vi "Wago Main Driver.vi"(10 "Remote Port":u16=502, 11 "Remote IP Address":string="172.16.90.113") -> (3 "System Data":string[][](array[string])=[["Station 1 Volt 1", "166.520"], ["Station 1 Volt 2", "0.030"], ["Station 2 Volt 1", "166.120"], ["Station 2 Volt 2", "90.720"], ["Station 3 Volt 1", "166.280"], ["Station 3 Volt 2", "91.440"], ["Station 4 Volt 1", "165.960"], ["Station 4 Volt 2", "94.400"], ["Station 5 Volt 1", "166.040"], ["Station 5 Volt 2", "94.800"], ["Station 6 Volt 1", "166.200"], ["Station 6 Volt 2", "93.280"], ["Station 7 Volt 1", "166.040"], ["Station 7 Volt 2", "90.720"], ["Station 8 Volt 1", "165.720"], ["Station 8 Volt 2", "88.320"], ["Room Humidity (Measured)", "175.560"], ["Room Temperature (Measured)", "183.880"], ["Spare 1", "0.000"], ["Spare 2", "0.000"], ["Supply Temperature (Measured)", "3.100"], ["Cooling Temperature (Measured)", "2.950"], ["Dehumidification Temperatuer (Measured)", "2.210"], ["Unused", "327.670"], ["Volt Rate 1", "5"], ["Volt Rate 2", "5"], ["Volt Rate 3", "0"], ["Volt Rate 4", "0"], ["Volt Rate 5", "0"], ["Volt Rate 6", "0"], ["Volt Rate 7", "0"], ["Volt Rate 8", "0"], ["Volt Window 1", "30"], ["Volt Window 2", "60"], ["Volt Window 3", "0"], ["Volt Window 4", "0"], ["Volt Window 5", "30"], ["Volt Window 6", "60"], ["Volt Window 7", "0"], ["Volt Window 8", "0"], ["Voltage Setpoint 1", "115.260"], ["Voltage Setpoint 2", "115.150"], ["Voltage Setpoint 3", "115.370"], ["Voltage Setpoint 4", "115.080"], ["Voltage Setpoint 5", "115.170"], ["Voltage Setpoint 6", "115.310"], ["Voltage Setpoint 7", "115.310"], ["Voltage Setpoint 8", "114.850"], ["Volt Range 1", "1"], ["Volt Range 2", "1"], ["Volt Range 3", "1"], ["Volt Range 4", "1"], ["Volt Range 5", "1"], ["Volt Range 6", "1"], ["Volt Range 7", "1"], ["Volt Range 8", "1"], ["Volt Polarity 1", "0"], ["Volt Polarity 2", "0"], ["Volt Polarity 3", "0"], ["Volt Polarity 4", "0"], ["Volt Polarity 5", "0"], ["Volt Polarity 6", "0"], ["Volt Polarity 7", "0"], ["Volt Polarity 8", "0"], ["Room Setpoint Temperature", "90.000"], ["Room Setpoint Humidity", "20.000"], ["Room Cool Temperature", "85.000"], ["Room Dehumidification Temperature", "75.000"], ["Room Run", "True"], ["Room OK", "False"], ["Room Testing", "False"], ["Emergency Stop", "True"], ["Chamber Door Switch", "True"], ["Safety Switch", "True"], ["Room Dry P", "200"], ["Room Dry I", "15000"], ["Room Humidity P", "400"], ["Room Humidity I", "15000"], ["Room Heat P", "1000"], ["Room Heat I", "2000"], ["Room Cool Temperature P", "500"], ["Room Cool Temperature I", "6000"], ["Room Dehumidification Temperature P", "500"], ["Room Dehumidification Temperature I", "6000"], ["Dehumidification Control (Wago Output)", "8191"], ["Cool Control (Wago Output)", "8129"], ["Steam Control (Wago Output)", "0"], ["Heat Control (Wago Output)", "12620"], ["Room Temperature (°F)", "90.140"], ["Room Humidity (%)", "41.960"], ["Supply Temperature (°F)", "87.670"], ["Cool Temperature (°F)", "85.060"], ["Dehumidification Temperature (°F)", "71.920"], ["Glycol Temperature (°F)", "0.000"], ["Heat Rate (%)", "23.140"], ["Steam Rate (%)", "0.000"], ["Cool Rate (%)", "24.810"], ["Dehumidification Rate (%)", "0.000"], ["Room Status", "0"], ["Door Enable", "1"], ["Station 1, Door 1", "0"], ["Station 1, Door 2", "0"], ["Station 1, Door 3", "0"], ["Station 2, Door 1", "0"], ["Station 2, Door 2", "0"], ["Station 2, Door 3", "0"], ["Station 3, Door 1", "0"], ["Station 3, Door 2", "0"], ["Station 3, Door 3", "0"], ["Station 4, Door 1", "0"], ["Station 4, Door 2", "0"], ["Station 4, Door 3", "0"], ["Station 5, Door 1", "1607"], ["Station 5, Door 2", "1607"], ["Station 5, Door 3", "1607"], ["Station 6, Door 1", "0"], ["Station 6, Door 2", "0"], ["Station 6, Door 3", "0"], ["Station 7, Door 1", "0"], ["Station 7, Door 2", "0"], ["Station 7, Door 3", "0"], ["Station 8, Door 1", "0"], ["Station 8, Door 2", "0"], ["Station 8, Door 3", "0"], ["Door Opener Enable", "True"], ["Volt Monitor 1", "115.260"], ["Volt Monitor 2", "115.150"], ["Volt Monitor 3", "115.370"], ["Volt Monitor 4", "115.080"], ["Volt Monitor 5", "115.170"], ["Volt Monitor 6", "115.310"], ["Volt Monitor 7", "115.310"], ["Volt Monitor 8", "114.850"], ["Volt Status 1", "1"], ["Volt Status 2", "1"], ["Volt Status 3", "1"], ["Volt Status 4", "1"], ["Volt Status 5", "1"], ["Volt Status 6", "1"], ["Volt Status 7", "1"], ["Volt Status 8", "1"], ["60 Hz Power", "True"], ["50 Hz Power", "False"], ["120V Range", "True"], ["240V Range", "False"], ["Ground Line", "False"], ["Ground Neutral", "True"], ["Measure Ground Leakage Current (mA)", "Measure GL"], ["Room OK", "True"], ["60 Hz Power", "True"], ["50 Hz Power", "False"], ["120V Range", "True"], ["240V Range", "False"], ["Ground Line", "False"], ["Ground Neutral", "True"], ["Measure Ground Leakage Current (mA)", "Disable GL Measure"], ["Fault", "False"], ["60 Hz Power", "True"], ["50 Hz Power", "False"], ["120V Range", "True"], ["240V Range", "False"], ["Ground Line", "False"], ["Ground Neutral", "True"], ["Measure Ground Leakage Current (mA)", "Disable GL Measure"], ["Room Heat", "True"], ["60 Hz Power", "True"], ["50 Hz Power", "False"], ["120V Range", "True"], ["240V Range", "False"], ["Ground Line", "False"], ["Ground Neutral", "True"], ["Measure Ground Leakage Current (mA)", "Disable GL Measure"], ["Room Blower", "True"], ["60 Hz Power", "True"], ["50 Hz Power", "False"], ["120V Range", "True"], ["240V Range", "False"], ["Ground Line", "False"], ["Ground Neutral", "True"], ["Measure Ground Leakage Current (mA)", "Disable GL Measure"], ["Spare", "False"], ["60 Hz Power", "True"], ["50 Hz Power", "False"], ["120V Range", "True"], ["240V Range", "False"], ["Ground Line", "False"], ["Ground Neutral", "True"], ["Measure Ground Leakage Current (mA)", "Disable GL Measure"], ["Room Pump", "True"], ["60 Hz Power", "True"], ["50 Hz Power", "False"], ["120V Range", "True"], ["240V Range", "False"], ["Ground Line", "False"], ["Ground Neutral", "True"], ["Measure Ground Leakage Current (mA)", "Disable GL Measure"], ["Room OK", "False"], ["60 Hz Power", "True"], ["50 Hz Power", "False"], ["120V Range", "True"], ["240V Range", "False"], ["Ground Line", "False"], ["Ground Neutral", "True"], ["Measure Ground Leakage Current (mA)", "Disable GL Measure"], ["Fault", "False"], ["Station 1 Freezer", "False"], ["Station 1 Cab", "False"], ["Station 1 Slide", "False"], ["Station 2 Freezer", "False"], ["Station 2 Cab", "False"], ["Station 2 Slide", "False"], ["Station 3 Freezer", "False"], ["Station 3 Cab", "False"], ["Station 3 Slide", "False"], ["Station 4 Freezer", "False"], ["Station 4 Cab", "False"], ["Station 4 Slide", "False"], ["Station 5 Freezer", "False"], ["Station 5 Cab", "False"], ["Station 5 Slide", "False"], ["Station 6 Freezer", "False"], ["Station 6 Cab", "False"], ["Station 6 Slide", "False"], ["Station 7 Freezer", "False"], ["Station 7 Cab", "False"], ["Station 7 Slide", "False"], ["Station 8 Freezer", "False"], ["Station 8 Cab", "False"], ["Station 8 Slide", "False"], ["Station 1 Volt Increase", "False"], ["Station 1 Volt Decrease", "False"], ["Station 2 Volt Increase", "False"], ["Station 2 Volt Decrease", "False"], ["Station 3 Volt Increase", "False"], ["Station 3 Volt Decrease", "False"], ["Station 4 Volt Increase", "False"], ["Station 4 Volt Decrease", "False"], ["Station 5 Volt Increase", "False"], ["Station 5 Volt Decrease", "False"], ["Station 6 Volt Increase", "False"], ["Station 6 Volt Decrease", "False"], ["Station 7 Volt Increase", "False"], ["Station 7 Volt Decrease", "False"], ["Station 8 Volt Increase", "False"], ["Station 8 Volt Decrease", "False"]])   [LabVIEW 2016]
uses:
  Type Definitions/Wago Main Control.ctl
  Type Definitions/Wago Output Data Process Image.ctl
  Type Definitions/Wago Room Condtions.ctl
  Type Definitions/Wago Door Relays.ctl
  Type Definitions/Wago Contactor Settings.ctl
  Type Definitions/Wago Ground Leakage.ctl
  Type Definitions/Wago Input Process Image.ctl
  Type Definitions/Wago Room PID Settings.ctl
  Type Definitions/Wago Measured Input Data.ctl
  Type Definitions/Wago Room Setpoint Targets.ctl
  Type Definitions/Wago Ground Leakage Relays.ctl
  Type Definitions/Wago Door Settings.ctl
  Type Definitions/Wago Door Relays By Station.ctl
  Type Definitions/Wago Door Operation.ctl
  Trunk/Refrigeration/RTS/Type Definitions/RTS Enable Door Openers.ctl
  Type Definitions/Wago Polarity Selector Relays.ctl
  Type Definitions/Wago Polarity Selector.ctl
  Type Definitions/Wago Room Enable.ctl
  Type Definitions/Wago Room Run.ctl
  Type Definitions/Wago Voltage Adjustment Parameters.ctl
  Trunk/Refrigeration/RTS/Type Definitions/RTS Frequency Selector.ctl
  Trunk/Refrigeration/RTS/Type Definitions/RTS Chamber Temperature Humidity Control.ctl
  Type Definitions/Wago Input Commands.ctl
  <vilib>/NI/Modbus Library/API/Wrapper/Create TCP Master.vi
  <vilib>/NI/Modbus Library/API/Master/Modbus Master.lvclass
  <vilib>/NI/Modbus Library/API/Wrapper/API Main.lvlib
panel:
  out "System Data to Save":string[][](array[string])=[["Room Temperature (°F)", "90.140"], ["Room Humidity (%)", "41.960"], ["Supply Temperature (°F)", "87.670"], ["Cool Temperature (°F)", "85.060"], ["Dehumidification Temperature (°F)", "71.920"], ["Glycol Temperature (°F)", "0.000"], ["Heat Rate (%)", "23.140"], ["Steam Rate (%)", "0.000"], ["Cool Rate (%)", "24.810"], ["Dehumidification Rate (%)", "0.000"], ["Room Status", "0"], ["Door Enable", "1"]]
  in  "Tab Control":enum32{"Setup Tab", "Relay Tab"}(tab)
  in  "Room Setpoints":T1={"Room Setpoint Temperature (*RM Dry Set P1)"=90.0, "Room Setpoint Humidity (*RM Hum Set P1)"=20.0, "Room Cool Temperature (*RM Cool Setp 1)"=65.0, "Room Dehum Temperature (*RM De Hum Set P1)"=60.0} {"Room Dehum Temperature (*RM De Hum Set P1)" min=30.0 max=120.0; "Room Cool Temperature (*RM Cool Setp 1)" min=30.0 max=120.0; "Room Setpoint Humidity (*RM Hum Set P1)" min=5.0 max=98.0; "Room Setpoint Temperature (*RM Dry Set P1)" min=40.0 max=120.0}
  in  "Path":path=path "C:/Technology Lab/NI-2010/Trunk/Refrigeration/RTS/Old System"
  in  "Reload PID":bool
  in  "Room PID Parameters":bool
  in  "Room PID Settings":T2={"Room Dry P(*RM Dry P1)"=2, "Room Dry I (*RM Dry I1)"=1500, "Room Humidity P (*RM Hum P1)"=4, "Room Humidity I (*RM Hum I1)"=1500, "Room Heat P (*RM Heat P1)"=10, "Room Heat I (*RM Heat I1)"=200, "Room Cool Temperature P (*RM Cool P1)"=5, "Room Cool Temperature I (*RM Cool I1)"=600, "Room Dehumid Temperature P (*RM Dehum P1)"=5, "Room Dehumid Temperature I (*RM Dehum I1)"=600} {"Room Dehumid Temperature I (*RM Dehum I1)" max=30000 step=1; "Room Dehumid Temperature P (*RM Dehum P1)" max=30000 step=1; "Room Cool Temperature I (*RM Cool I1)" max=30000 step=1; "Room Cool Temperature P (*RM Cool P1)" max=30000 step=1; "Room Heat I (*RM Heat I1)" max=30000 step=1; "Room Heat P (*RM Heat P1)" max=30000 step=1; "Room Humidity I (*RM Hum I1)" max=30000 step=1; "Room Humidity P (*RM Hum P1)" max=30000 step=1; "Room Dry I (*RM Dry I1)" max=30000 step=1; "Room Dry P(*RM Dry P1)" max=30000 step=1}
  in  "Chamber Setpoint":bool
  in  "Update Voltage Adjustment Parameters":bool
  in  "Voltage Adjustment Parameters":T3={"Volt Rate 1"=30, "Volt Rate 2"=30, "Volt Rate 3"=30, "Volt Rate 4"=30, "Volt Rate 5"=30, "Volt Rate 6"=30, "Volt Rate 7"=30, "Volt Rate 8"=30, "Volt Window 1 & 5"=10, "Volt Window 2 & 6"=10, "Volt Window 3 & 7 "=10, "Volt Window 4 & 8"=10}
  in  "Room OK?":T4
  in  "Room Run":T5
  in  "OK":bool
  in  "Voltage 8":dbl
  in  "Frequency 8":T6 items=["60 Hz", "50 Hz"]
  in  "Voltage 7":dbl
  in  "Frequency 7":T6 items=["60 Hz", "50 Hz"]
  in  "Voltage 6":dbl
  in  "Frequency 6":T6 items=["60 Hz", "50 Hz"]
  in  "Voltage 5":dbl
  in  "Frequency 5":T6 items=["60 Hz", "50 Hz"]
  in  "Voltage 4":dbl
  in  "Frequency 4":T6 items=["60 Hz", "50 Hz"]
  in  "Voltage 3":dbl
  in  "Frequency 3":T6 items=["60 Hz", "50 Hz"]
  in  "Voltage 2":dbl
  in  "Frequency 2":T6 items=["60 Hz", "50 Hz"]
  in  "Voltage":dbl
  in  "Frequency":T6 items=["60 Hz", "50 Hz"]
  in  "Ground Leak Relays":T7
  in  "Polarity Selector":T9
  in  "Station 8 CMD":bool
  in  "Station 7 CMD":bool
  in  "Station 6 CMD":bool
  in  "Station 5 CMD":bool
  in  "Station 4 CMD":bool
  in  "Station 3 CMD":bool
  in  "Station 2 CMD":bool
  in  "Station 1 CMD":bool
  in  "Door Settings":T11={"Station 1"={"Freezer"=enum."Clear Time Close Door", "Cab"=enum."Clear Time Close Door", "Slide"=enum."Clear Time Close Door"}, "Station 2"={"Freezer"=enum."Clear Time Close Door", "Cab"=enum."Clear Time Close Door", "Slide"=enum."Clear Time Close Door"}, "Station 3"={"Freezer"=enum."Clear Time Close Door", "Cab"=enum."Clear Time Close Door", "Slide"=enum."Clear Time Close Door"}, "Station 4"={"Freezer"=enum."Clear Time Close Door", "Cab"=enum."Clear Time Close Door", "Slide"=enum."Clear Time Close Door"}, "Station 5"={"Freezer"=enum."Clear Time Close Door", "Cab"=enum."Clear Time Close Door", "Slide"=enum."Clear Time Close Door"}, "Station 6"={"Freezer"=enum."Clear Time Close Door", "Cab"=enum."Clear Time Close Door", "Slide"=enum."Clear Time Close Door"}, "Station 7"={"Freezer"=enum."Clear Time Close Door", "Cab"=enum."Clear Time Close Door", "Slide"=enum."Clear Time Close Door"}, "Station 8"={"Freezer"=enum."Clear Time Close Door", "Cab"=enum."Clear Time Close Door", "Slide"=enum."Clear Time Close Door"}, "Door Enable"=enum."Enable Door Openers"}
  in  "Station Voltage Send 1":bool
  in  "Station Voltage Send 5":bool
  in  "Station Voltage Send 2":bool
  in  "Station Voltage Send 6":bool
  in  "Station Voltage Send 3":bool
  in  "Station Voltage Send 7":bool
  in  "Station Voltage Send 4":bool
  in  "Station Voltage Send 8":bool
  out "Wago Data Output":T15={"Output Data Process Image"={"Room Door Opener Status"={"Station 1, Door 1"=0, "Station 1, Door 2"=0, "Station 1, Door 3"=0, "Station 2, Door 1"=0, "Station 2, Door 2"=1615, "Station 2, Door 3"=0, "Station 3, Door 1"=1615, "Station 3, Door 2"=1611, "Station 3, Door 3"=0, "Station 4, Door 1"=4807, "Station 4, Door 2"=0, "Station 4, Door 3"=0, "Station 5, Door 1"=1615, "Station 5, Door 2"=0, "Station 5, Door 3"=1611, "Station 6, Door 1"=1611, "Station 6, Door 2"=0, "Station 6, Door 3"=4803, "Station 7, Door 1"=0, "Station 7, Door 2"=0, "Station 7, Door 3"=1611, "Station 8, Door 1"=0, "Station 8, Door 2"=1611, "Station 8, Door 3"=1611}, "Room Conditions (Measured)"={"twDoorEna(*Door Enable)"=1, "twStatus(*Rm Status1)"=0, "twRoomTemp (*Rm Dry1)"=90.14, "twRoomHum (*Rm Hum1)"=23.75, "twSuppTemp(*Rm Supp T1)"=87.49, "twCoolTemp(*Rm Cool T1)"=86.5, "twDehumTemp(*Rm Dehum T1)"=72.19, "twGlycolTemp(*Rm Gly T1-Not Used)"=0.0, "twDehumRate(*Rm Dehum Valve1)"=68.17, "twCoolRate(*Rm Cool Valve1)"=15.6, "twSteamRate(*Rm Steam Valve1)"=0.0, "twHeatRate (*Rm Heat Ctrl1)"=33.98}, "Chamber AO Controls (Controls Chamber)"={"twDehumCtrl (mA)"=249, "twCoolCtrl (mA)"=51, "twSteamCtrl (mA)"=0, "twHeatCtrl (mA)"=155}, "Variac Output(*All Check Out)"={"Station 1 Volt Increase"=FALSE, "Station 1 Volt Decrease"=FALSE, "Station 2 Volt Increase"=FALSE, "Station 2 Volt Decrease"=FALSE, "Station 3 Volt Increase"=FALSE, "Station 3 Volt Decrease"=FALSE, "Station 4 Volt Increase"=FALSE, "Station 4 Volt Decrease"=FALSE, "Station 5 Volt Increase"=FALSE, "Station 5 Volt Decrease"=FALSE, "Station 6 Volt Increase"=FALSE, "Station 6 Volt Decrease"=FALSE, "Station 7 Volt Increase"=FALSE, "Station 7 Volt Decrease"=FALSE, "Station 8 Volt Increase"=FALSE, "Station 8 Volt Decrease"=FALSE}, "Door Output Relays"={"Station 1 Freezer"=FALSE, "Station 1 Cab"=FALSE, "Station 1 Slide"=FALSE, "Station 2 Freezer"=FALSE, "Station 2 Cab"=FALSE, "Station 2 Slide"=FALSE, "Station 3 Freezer"=FALSE, "Station 3 Cab"=FALSE, "Station 3 Slide"=FALSE, "Station 4 Freezer"=FALSE, "Station 4 Cab"=FALSE, "Station 4 Slide"=FALSE, "Station 5 Freezer"=FALSE, "Station 5 Cab"=FALSE, "Station 5 Slide"=FALSE, "Station 6 Freezer"=FALSE, "Station 6 Cab"=FALSE, "Station 6 Slide"=FALSE, "Station 7 Freezer"=FALSE, "Station 7 Cab"=FALSE, "Station 7 Slide"=FALSE, "Station 8 Freezer"=FALSE, "Station 8 Cab"=FALSE, "Station 8 Slide"=FALSE, "Door Opener Enable"=TRUE}, "Wago Input Voltage Monitor (*Target_ All Check Out)"={"twWoltMon1"=115.06, "twWoltMon2"=115.3, "twWoltMon3"=115.37, "twWoltMon4"=115.21, "twWoltMon5"=115.39, "twWoltMon6"=115.22, "twWoltMon7"=115.26, "twWoltMon8"=119.98, "twVoltStat1"=1, "twVoltStat2"=1, "twVoltStat3"=1, "twVoltStat4"=1, "twVoltStat5"=1, "twVoltStat6"=1, "twVoltStat7"=1, "twVoltStat8"=1}, "Contactor Settings(*All Check Out)"={"Station 1"={"60 Hz Power"=TRUE, "50 Hz Power"=FALSE, "120V Range"=TRUE, "240V Range"=FALSE, "Ground Line"=FALSE, "Ground Neutral"=TRUE, "Room OK"=FALSE, "Ground Leakage"=enum."1 - Measure GL"}, "Station 2"={"60 Hz Power"=TRUE, "50 Hz Power"=FALSE, "120V Range"=TRUE, "240V Range"=FALSE, "Ground Line"=FALSE, "Ground Neutral"=TRUE, "Fault"=FALSE, "Ground Leakage"=enum."1 - Measure GL"}, "Station 3"={"60 Hz Power"=TRUE, "50 Hz Power"=FALSE, "120V Range"=TRUE, "240V Range"=FALSE, "Ground Line"=FALSE, "Ground Neutral"=TRUE, "Room Heat"=TRUE, "Ground Leakage"=enum."1 - Measure GL"}, "Station 4"={"60 Hz Power"=TRUE, "50 Hz Power"=FALSE, "120V Range"=TRUE, "240V Range"=FALSE, "Ground Line"=FALSE, "Ground Neutral"=TRUE, "Room Blower"=TRUE, "Ground Leakage"=enum."1 - Measure GL"}, "Station 5"={"60 Hz Power"=TRUE, "50 Hz Power"=FALSE, "120V Range"=TRUE, "240V Range"=FALSE, "Ground Line"=FALSE, "Ground Neutral"=TRUE, "Spare"=FALSE, "Ground Leakage"=enum."0 - Normal GL"}, "Station 6"={"60 Hz Power"=TRUE, "50 Hz Power"=FALSE, "120V Range"=TRUE, "240V Range"=FALSE, "Ground Line"=FALSE, "Ground Neutral"=TRUE, "Room Pump"=TRUE, "Ground Leakage"=enum."0 - Normal GL"}, "Station 7"={"60 Hz Power"=TRUE, "50 Hz Power"=FALSE, "120V Range"=TRUE, "240V Range"=FALSE, "Ground Line"=FALSE, "Ground Neutral"=TRUE, "Spare"=FALSE, "Ground Leakage"=enum."0 - Normal GL"}, "Station 8"={"60 Hz Power"=TRUE, "50 Hz Power"=FALSE, "120V Range"=TRUE, "240V Range"=FALSE, "Ground Line"=FALSE, "Ground Neutral"=TRUE, "Spare"=FALSE, "Ground Leakage"=enum."0 - Normal GL"}}}, "Input Process Image"={"fbEstop"=TRUE, "fbDoors"=TRUE, "fbSafety"=TRUE, "Input Variables"={"Station 1 Volt 1"=65.36, "Station 1 Volt 2"=65.12, "Station 2 Volt 1"=166.04, "Station 2 Volt 2"=77.04, "Station 3 Volt 1"=166.12, "Station 3 Volt 2"=80.08, "Station 4 Volt 1"=166.04, "Station 4 Volt 2"=86.32, "Station 5 Volt 1"=166.2, "Station 5 Volt 2"=89.84, "Station 6 Volt 1"=166.28, "Station 6 Volt 2"=81.76, "Station 7 Volt 1"=166.36, "Station 7 Votl 2"=78.64, "Station 8 Volt 1"=170.28, "Station 8 Volt 2"=75.76}, "Input Data"={"Room Humidity  (Measured)"=127.52, "Room Temperature (Measured)"=183.8, "Spare 1"=0.0, "Spare 2"=0.0, "Supply Temperature (Measured)"=3.1, "Cooling Temperature (Measured)"=3.03, "Dehumidification Temperature (Measured)"=2.21, "Un-used"=327.67}, "Software Constants"={"Volt Rate 1"=0, "Volt Rate 2"=0, "Volt Rate 3"=0, "Volt Rate 4"=0, "Volt Rate 5"=0, "Volt Rate 6"=0, "Volt Rate 7"=0, "Volt Rate 8"=0, "Volt Window 1"=0, "Volt Window 2"=1, "Volt Window 3"=0, "Volt Window 4"=0, "Volt Window 5"=0, "Volt Window 6"=1, "Volt Window 7"=0, "Volt Window 8"=0, "Voltage Range 1"=0, "Voltage Range 2"=0, "Voltage Range 3"=0, "Voltage Range 4"=0, "Voltage Range 5"=0, "Voltage Range 6"=0, "Voltage Range 7"=0, "Voltage Range 8"=0, "Voltage Polarity 1"=0, "Voltage Polarity 2"=0, "Voltage Polarity 3"=0, "Voltage Polarity 4"=0, "Voltage Polarity 5"=0, "Voltage Polarity 6"=0, "Voltage Polarity 7"=0, "Voltage Polarity 8"=0, "Room Run"=TRUE, "Room OK"=FALSE, "Room Testing"=FALSE, "Room PID Settings"={"Room Dry P(*RM Dry P1)"=2, "Room Dry I (*RM Dry I1)"=1500, "Room Humidity P (*RM Hum P1)"=4, "Room Humidity I (*RM Hum I1)"=1500, "Room Heat P (*RM Heat P1)"=10, "Room Heat I (*RM Heat I1)"=200, "Room Cool Temperature P (*RM Cool P1)"=5, "Room Cool Temperature I (*RM Cool I1)"=600, "Room Dehumid Temperature P (*RM Dehum P1)"=5, "Room Dehumid Temperature I (*RM Dehum I1)"=600}}, "Measured Input Data (Target)"={"Voltage Setpoint 1 (*Volt Set1)"=115.06, "Voltage Setpoint 2 (*Volt Set2)"=115.3, "Voltage Setpoint 3 (*Volt Set3)"=115.37, "Voltage Setpoint 4 (*Volt Set4)"=115.21, "Voltage Setpoint 5 (*Volt Set5)"=115.39, "Voltage Setpoint 6 (*Volt Set6)"=115.22, "Voltage Setpoint 7 (*Volt Set7)"=115.26, "Voltage Setpoint 8 (*Volt Set8)"=119.98, "Room Setpoints"={"Room Setpoint Temperature (*RM Dry Set P1)"=90.0, "Room Setpoint Humidity (*RM Hum Set P1)"=20.0, "Room Cool Temperature (*RM Cool Setp 1)"=85.0, "Room Dehum Temperature (*RM De Hum Set P1)"=70.0}}}, "System Send Data"=[], "System Data To Save"=[]} {"Input Process Image"."Software Constants"."Room PID Settings"."Room Dehumid Temperature I (*RM Dehum I1)" max=30000 step=1; "Input Process Image"."Software Constants"."Room PID Settings"."Room Dehumid Temperature P (*RM Dehum P1)" max=30000 step=1; "Input Process Image"."Software Constants"."Room PID Settings"."Room Cool Temperature I (*RM Cool I1)" max=30000 step=1; "Input Process Image"."Software Constants"."Room PID Settings"."Room Cool Temperature P (*RM Cool P1)" max=30000 step=1; "Input Process Image"."Software Constants"."Room PID Settings"."Room Heat I (*RM Heat I1)" max=30000 step=1; "Input Process Image"."Software Constants"."Room PID Settings"."Room Heat P (*RM Heat P1)" max=30000 step=1; "Input Process Image"."Software Constants"."Room PID Settings"."Room Humidity I (*RM Hum I1)" max=30000 step=1; "Input Process Image"."Software Constants"."Room PID Settings"."Room Humidity P (*RM Hum P1)" max=30000 step=1; "Input Process Image"."Software Constants"."Room PID Settings"."Room Dry I (*RM Dry I1)" max=30000 step=1; "Input Process Image"."Software Constants"."Room PID Settings"."Room Dry P(*RM Dry P1)" max=30000 step=1}
  in  "Wago Data Input":T15 {"Input Process Image"."Software Constants"."Room PID Settings"."Room Dehumid Temperature I (*RM Dehum I1)" max=30000 step=1; "Input Process Image"."Software Constants"."Room PID Settings"."Room Dehumid Temperature P (*RM Dehum P1)" max=30000 step=1; "Input Process Image"."Software Constants"."Room PID Settings"."Room Cool Temperature I (*RM Cool I1)" max=30000 step=1; "Input Process Image"."Software Constants"."Room PID Settings"."Room Cool Temperature P (*RM Cool P1)" max=30000 step=1; "Input Process Image"."Software Constants"."Room PID Settings"."Room Heat I (*RM Heat I1)" max=30000 step=1; "Input Process Image"."Software Constants"."Room PID Settings"."Room Heat P (*RM Heat P1)" max=30000 step=1; "Input Process Image"."Software Constants"."Room PID Settings"."Room Humidity I (*RM Hum I1)" max=30000 step=1; "Input Process Image"."Software Constants"."Room PID Settings"."Room Humidity P (*RM Hum P1)" max=30000 step=1; "Input Process Image"."Software Constants"."Room PID Settings"."Room Dry I (*RM Dry I1)" max=30000 step=1; "Input Process Image"."Software Constants"."Room PID Settings"."Room Dry P(*RM Dry P1)" max=30000 step=1}
  out "Error Out":errorcluster
  in  "Error In":errorcluster
  # "Need to pull directly from PLC..I cannont seem to\nfind the correct values :("
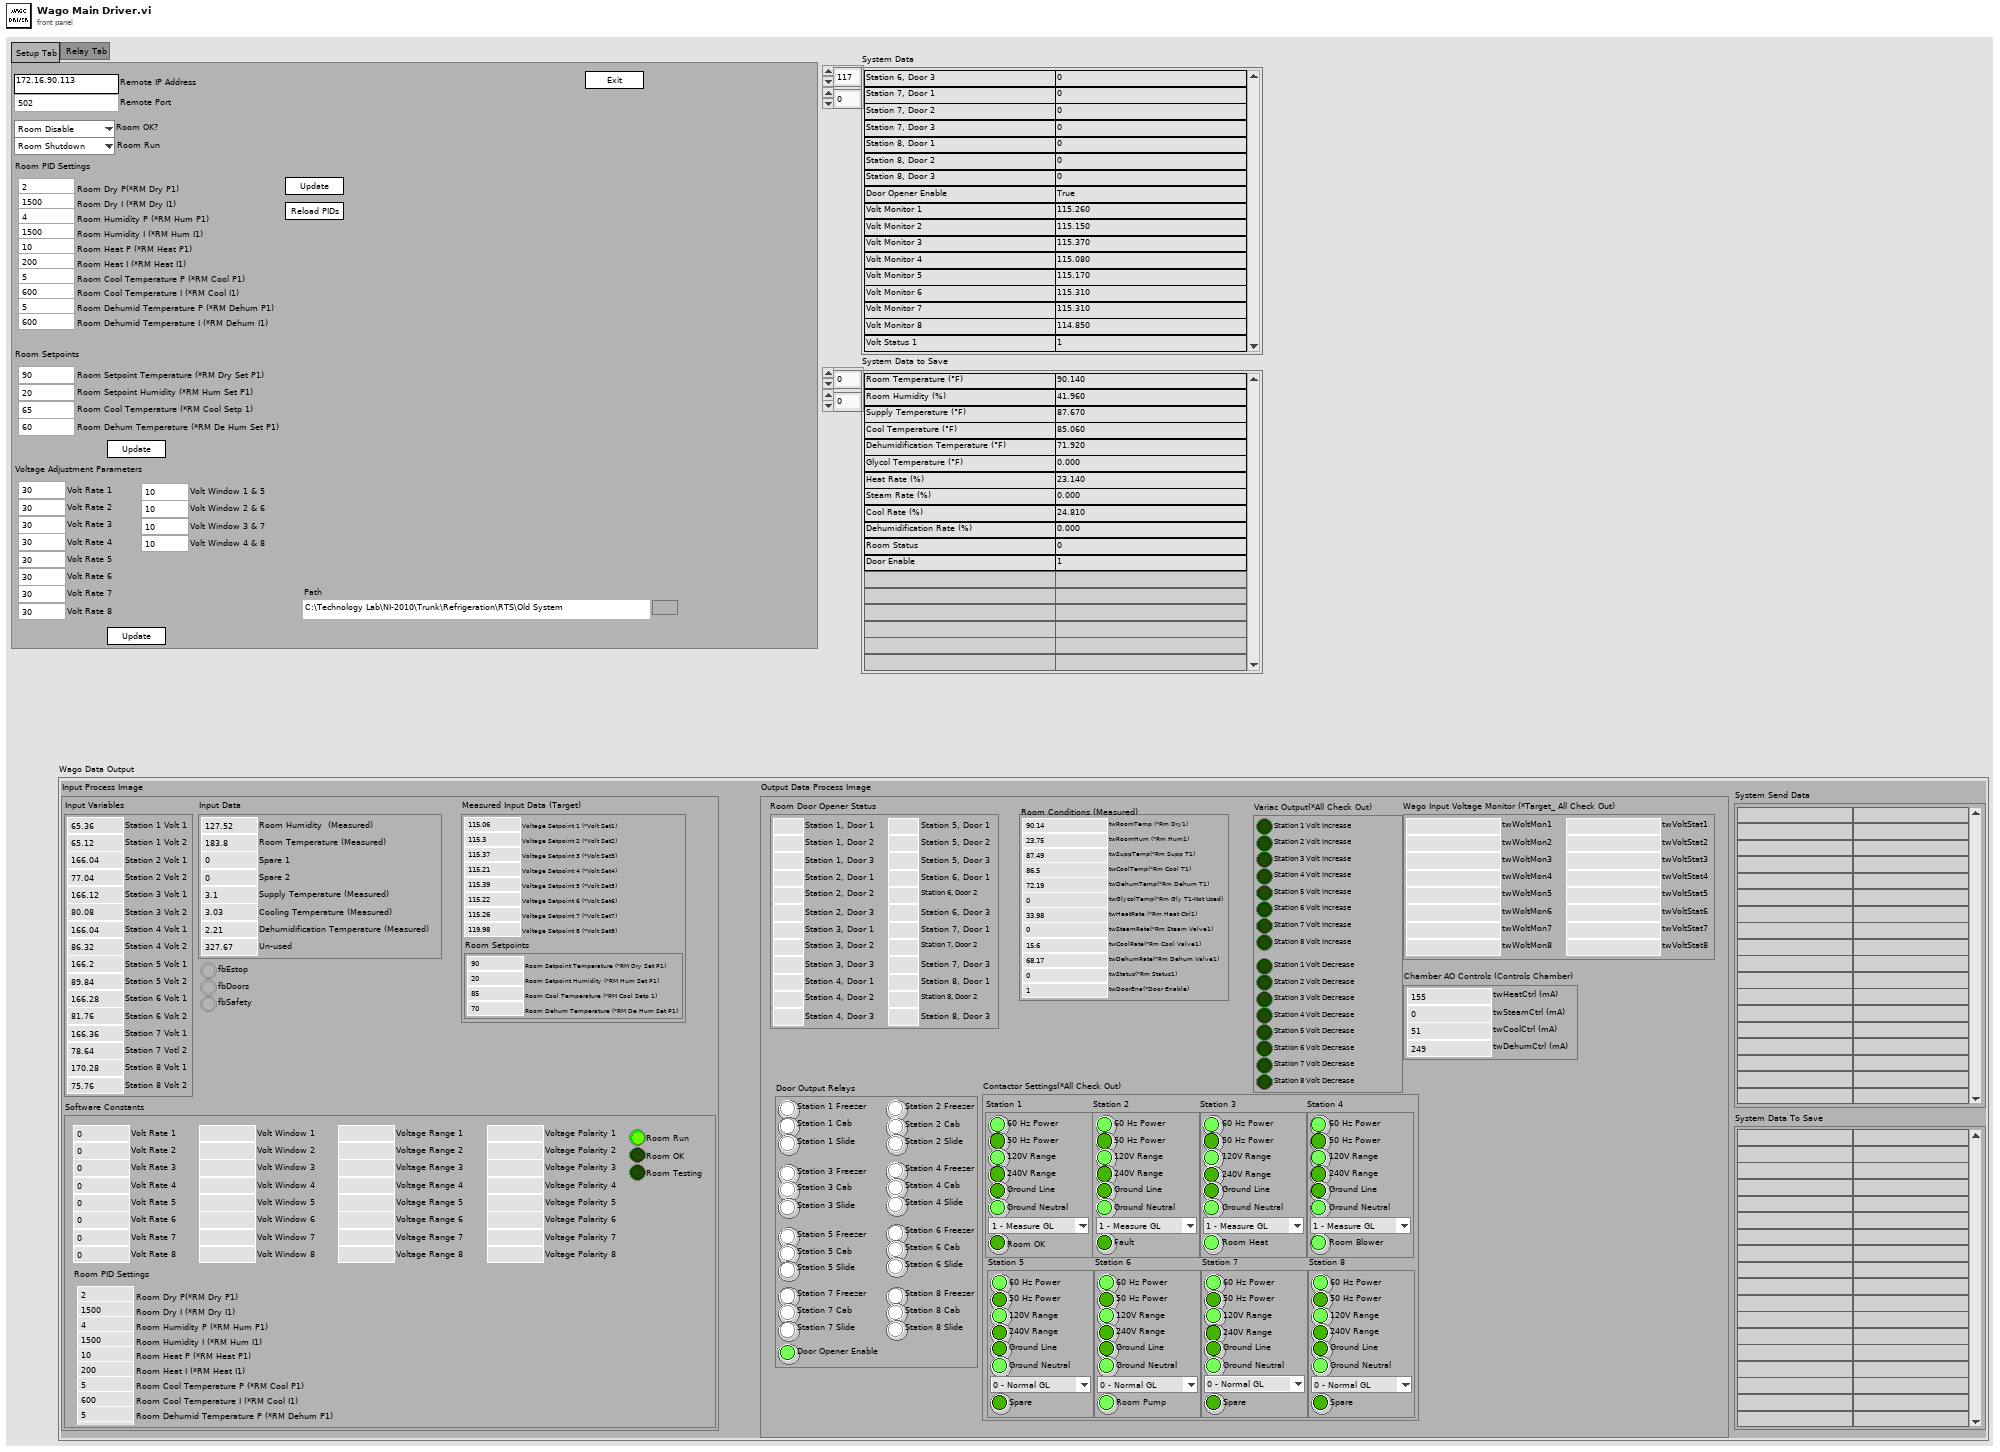
[diagram p1: front panel]
types:
  T1 = typedef "RTS Chamber Temperature Humidity Control.ctl" = cluster{"Room Setpoint Temperature (*RM Dry Set P1)":dbl, "Room Setpoint Humidity (*RM Hum Set P1)":dbl, "Room Cool Temperature (*RM Cool Setp 1)":dbl, "Room Dehum Temperature (*RM De Hum Set P1)":dbl}
  T2 = typedef "Wago Room PID Settings.ctl" = cluster{"Room Dry P(*RM Dry P1)":u16, "Room Dry I (*RM Dry I1)":u16, "Room Humidity P (*RM Hum P1)":u16, "Room Humidity I (*RM Hum I1)":u16, "Room Heat P (*RM Heat P1)":u16, "Room Heat I (*RM Heat I1)":u16, "Room Cool Temperature P (*RM Cool P1)":u16, "Room Cool Temperature I (*RM Cool I1)":u16, "Room Dehumid Temperature P (*RM Dehum P1)":u16, "Room Dehumid Temperature I (*RM Dehum I1)":u16}
  T3 = typedef "Wago Voltage Adjustment Parameters.ctl" = cluster{"Volt Rate 1":u16, "Volt Rate 2":u16, "Volt Rate 3":u16, "Volt Rate 4":u16, "Volt Rate 5":u16, "Volt Rate 6":u16, "Volt Rate 7":u16, "Volt Rate 8":u16, "Volt Window 1 & 5":u16, "Volt Window 2 & 6":u16, "Volt Window 3 & 7 ":u16, "Volt Window 4 & 8":u16}
  T4 = typedef "Wago Room Enable.ctl" = enum16{"Room Disable", "Room OK"}
  T5 = typedef "Wago Room Run.ctl" = enum16{"Room Shutdown", "Room Run"}
  T6 = typedef "RTS Frequency Selector.ctl" = u16
  T7 = typedef "Wago Ground Leakage Relays.ctl" = cluster{"Ground Leakage 1":T8, "Ground Leakage 2":T8, "Ground Leakage 3":T8, "Ground Leakage 4":T8, "Ground Leakage 5":T8, "Ground Leakage 6":T8, "Ground Leakage 7":T8, "Ground Leakage 8":T8}
  T8 = typedef "Wago Ground Leakage.ctl" = enum16{"0 - Normal GL", "1 - Measure GL"}
  T9 = typedef "Wago Polarity Selector Relays.ctl" = cluster{"Station 1":T10, "Station 2":T10, "Station 3":T10, "Station 4":T10, "Station 5":T10, "Station 6":T10, "Station 7":T10, "Station 8":T10}
  T10 = typedef "Wago Polarity Selector.ctl" = enum16{"Ground Neutral", "Ground Line"}
  T11 = typedef "Wago Door Settings.ctl" = cluster{"Station 1":T12, "Station 2":T12, "Station 3":T12, "Station 4":T12, "Station 5":T12, "Station 6":T12, "Station 7":T12, "Station 8":T12, "Door Enable":T14}
  T12 = typedef "Wago Door Relays By Station.ctl" = cluster{"Freezer":T13, "Cab":T13, "Slide":T13}
  T13 = typedef "Wago Door Operation.ctl" = enum16{"Clear Time Close Door", "Open Door", "Close Door", "PLC Timed Door Op"}
  T14 = typedef "RTS Enable Door Openers.ctl" = enum16{"Disable Door Openers", "Enable Door Openers"}
  T15 = typedef "Wago Main Control.ctl" = cluster{"Output Data Process Image":T16, "Input Process Image":T20, "System Send Data":string[][], "System Data To Save":string[][]}
  T16 = typedef "Wago Output Data Process Image.ctl" = cluster{"Room Door Opener Status":cluster{"Station 1, Door 1":u16, "Station 1, Door 2":u16, "Station 1, Door 3":u16, "Station 2, Door 1":u16, "Station 2, Door 2":u16, "Station 2, Door 3":u16, "Station 3, Door 1":u16, "Station 3, Door 2":u16, "Station 3, Door 3":u16, "Station 4, Door 1":u16, "Station 4, Door 2":u16, "Station 4, Door 3":u16, "Station 5, Door 1":u16, "Station 5, Door 2":u16, "Station 5, Door 3":u16, "Station 6, Door 1":u16, "Station 6, Door 2":u16, "Station 6, Door 3":u16, "Station 7, Door 1":u16, "Station 7, Door 2":u16, "Station 7, Door 3":u16, "Station 8, Door 1":u16, "Station 8, Door 2":u16, "Station 8, Door 3":u16}, "Room Conditions (Measured)":T17, "Chamber AO Controls (Controls Chamber)":cluster{"twDehumCtrl (mA)":u16, "twCoolCtrl (mA)":u16, "twSteamCtrl (mA)":u16, "twHeatCtrl (mA)":u16}, "Variac Output(*All Check Out)":cluster{"Station 1 Volt Increase":bool, "Station 1 Volt Decrease":bool, "Station 2 Volt Increase":bool, "Station 2 Volt Decrease":bool, "Station 3 Volt Increase":bool, "Station 3 Volt Decrease":bool, "Station 4 Volt Increase":bool, "Station 4 Volt Decrease":bool, "Station 5 Volt Increase":bool, "Station 5 Volt Decrease":bool, "Station 6 Volt Increase":bool, "Station 6 Volt Decrease":bool, "Station 7 Volt Increase":bool, "Station 7 Volt Decrease":bool, "Station 8 Volt Increase":bool, "Station 8 Volt Decrease":bool}, "Door Output Relays":T18, "Wago Input Voltage Monitor (*Target_ All Check Out)":cluster{"twWoltMon1":dbl, "twWoltMon2":dbl, "twWoltMon3":dbl, "twWoltMon4":dbl, "twWoltMon5":dbl, "twWoltMon6":dbl, "twWoltMon7":dbl, "twWoltMon8":dbl, "twVoltStat1":u16, "twVoltStat2":u16, "twVoltStat3":u16, "twVoltStat4":u16, "twVoltStat5":u16, "twVoltStat6":u16, "twVoltStat7":u16, "twVoltStat8":u16}, "Contactor Settings(*All Check Out)":T19}
  T17 = typedef "Wago Room Condtions.ctl" = cluster{"twDoorEna(*Door Enable)":u16, "twStatus(*Rm Status1)":u16, "twRoomTemp (*Rm Dry1)":dbl, "twRoomHum (*Rm Hum1)":dbl, "twSuppTemp(*Rm Supp T1)":dbl, "twCoolTemp(*Rm Cool T1)":dbl, "twDehumTemp(*Rm Dehum T1)":dbl, "twGlycolTemp(*Rm Gly T1-Not Used)":dbl, "twDehumRate(*Rm Dehum Valve1)":dbl, "twCoolRate(*Rm Cool Valve1)":dbl, "twSteamRate(*Rm Steam Valve1)":dbl, "twHeatRate (*Rm Heat Ctrl1)":dbl}
  T18 = typedef "Wago Door Relays.ctl" = cluster{"Station 1 Freezer":bool, "Station 1 Cab":bool, "Station 1 Slide":bool, "Station 2 Freezer":bool, "Station 2 Cab":bool, "Station 2 Slide":bool, "Station 3 Freezer":bool, "Station 3 Cab":bool, "Station 3 Slide":bool, "Station 4 Freezer":bool, "Station 4 Cab":bool, "Station 4 Slide":bool, "Station 5 Freezer":bool, "Station 5 Cab":bool, "Station 5 Slide":bool, "Station 6 Freezer":bool, "Station 6 Cab":bool, "Station 6 Slide":bool, "Station 7 Freezer":bool, "Station 7 Cab":bool, "Station 7 Slide":bool, "Station 8 Freezer":bool, "Station 8 Cab":bool, "Station 8 Slide":bool, "Door Opener Enable":bool}
  T19 = typedef "Wago Contactor Settings.ctl" = cluster{"Station 1":cluster{"60 Hz Power":bool, "50 Hz Power":bool, "120V Range":bool, "240V Range":bool, "Ground Line":bool, "Ground Neutral":bool, "Room OK":bool, "Ground Leakage":T8}, "Station 2":cluster{"60 Hz Power":bool, "50 Hz Power":bool, "120V Range":bool, "240V Range":bool, "Ground Line":bool, "Ground Neutral":bool, "Fault":bool, "Ground Leakage":T8}, "Station 3":cluster{"60 Hz Power":bool, "50 Hz Power":bool, "120V Range":bool, "240V Range":bool, "Ground Line":bool, "Ground Neutral":bool, "Room Heat":bool, "Ground Leakage":T8}, "Station 4":cluster{"60 Hz Power":bool, "50 Hz Power":bool, "120V Range":bool, "240V Range":bool, "Ground Line":bool, "Ground Neutral":bool, "Room Blower":bool, "Ground Leakage":T8}, "Station 5":cluster{"60 Hz Power":bool, "50 Hz Power":bool, "120V Range":bool, "240V Range":bool, "Ground Line":bool, "Ground Neutral":bool, "Spare":bool, "Ground Leakage":T8}, "Station 6":cluster{"60 Hz Power":bool, "50 Hz Power":bool, "120V Range":bool, "240V Range":bool, "Ground Line":bool, "Ground Neutral":bool, "Room Pump":bool, "Ground Leakage":T8}, "Station 7":cluster{"60 Hz Power":bool, "50 Hz Power":bool, "120V Range":bool, "240V Range":bool, "Ground Line":bool, "Ground Neutral":bool, "Spare":bool, "Ground Leakage":T8}, "Station 8":cluster{"60 Hz Power":bool, "50 Hz Power":bool, "120V Range":bool, "240V Range":bool, "Ground Line":bool, "Ground Neutral":bool, "Spare":bool, "Ground Leakage":T8}}
  T20 = typedef "Wago Input Process Image.ctl" = cluster{"fbEstop":bool, "fbDoors":bool, "fbSafety":bool, "Input Variables":cluster{"Station 1 Volt 1":dbl, "Station 1 Volt 2":dbl, "Station 2 Volt 1":dbl, "Station 2 Volt 2":dbl, "Station 3 Volt 1":dbl, "Station 3 Volt 2":dbl, "Station 4 Volt 1":dbl, "Station 4 Volt 2":dbl, "Station 5 Volt 1":dbl, "Station 5 Volt 2":dbl, "Station 6 Volt 1":dbl, "Station 6 Volt 2":dbl, "Station 7 Volt 1":dbl, "Station 7 Votl 2":dbl, "Station 8 Volt 1":dbl, "Station 8 Volt 2":dbl}, "Input Data":cluster{"Room Humidity  (Measured)":dbl, "Room Temperature (Measured)":dbl, "Spare 1":dbl, "Spare 2":dbl, "Supply Temperature (Measured)":dbl, "Cooling Temperature (Measured)":dbl, "Dehumidification Temperature (Measured)":dbl, "Un-used":dbl}, "Software Constants":cluster{"Volt Rate 1":u16, "Volt Rate 2":u16, "Volt Rate 3":u16, "Volt Rate 4":u16, "Volt Rate 5":u16, "Volt Rate 6":u16, "Volt Rate 7":u16, "Volt Rate 8":u16, "Volt Window 1":u16, "Volt Window 2":u16, "Volt Window 3":u16, "Volt Window 4":u16, "Volt Window 5":u16, "Volt Window 6":u16, "Volt Window 7":u16, "Volt Window 8":u16, "Voltage Range 1":u16, "Voltage Range 2":u16, "Voltage Range 3":u16, "Voltage Range 4":u16, "Voltage Range 5":u16, "Voltage Range 6":u16, "Voltage Range 7":u16, "Voltage Range 8":u16, "Voltage Polarity 1":u16, "Voltage Polarity 2":u16, "Voltage Polarity 3":u16, "Voltage Polarity 4":u16, "Voltage Polarity 5":u16, "Voltage Polarity 6":u16, "Voltage Polarity 7":u16, "Voltage Polarity 8":u16, "Room Run":bool, "Room OK":bool, "Room Testing":bool, "Room PID Settings":T2}, "Measured Input Data (Target)":T21}
  T21 = typedef "Wago Measured Input Data.ctl" = cluster{"Voltage Setpoint 1 (*Volt Set1)":dbl, "Voltage Setpoint 2 (*Volt Set2)":dbl, "Voltage Setpoint 3 (*Volt Set3)":dbl, "Voltage Setpoint 4 (*Volt Set4)":dbl, "Voltage Setpoint 5 (*Volt Set5)":dbl, "Voltage Setpoint 6 (*Volt Set6)":dbl, "Voltage Setpoint 7 (*Volt Set7)":dbl, "Voltage Setpoint 8 (*Volt Set8)":dbl, "Room Setpoints":T22}
  T22 = typedef "Wago Room Setpoint Targets.ctl" = cluster{"Room Setpoint Temperature (*RM Dry Set P1)":dbl, "Room Setpoint Humidity (*RM Hum Set P1)":dbl, "Room Cool Temperature (*RM Cool Setp 1)":dbl, "Room Dehum Temperature (*RM De Hum Set P1)":dbl}
  T23 = enum32{"invalid app kind", "Development System", "Run Time System", "Student Edition", "Embedded LabVIEW", "Evaluation", "Custom"}
  T24 = enum32{"Invalid", "Standard", "Closed", "Hidden", "Minimized", "Maximized"}
  T25 = cluster{"Core":cluster{"Current VI Reference":refnum<vi>, "Close Panel on Exit?":bool}, "Wago Data Input":T15}
  T26 = cluster{"Current VI Reference":refnum<vi>, "Close Panel on Exit?":bool}
  T27 = typedef "Wago Input Commands.ctl" = u16
  T28 = cluster{"Core":cluster{"Current VI Reference":refnum<vi>, "Close Panel on Exit?":bool}, "Your Boolean data":bool, "Your string data":string}
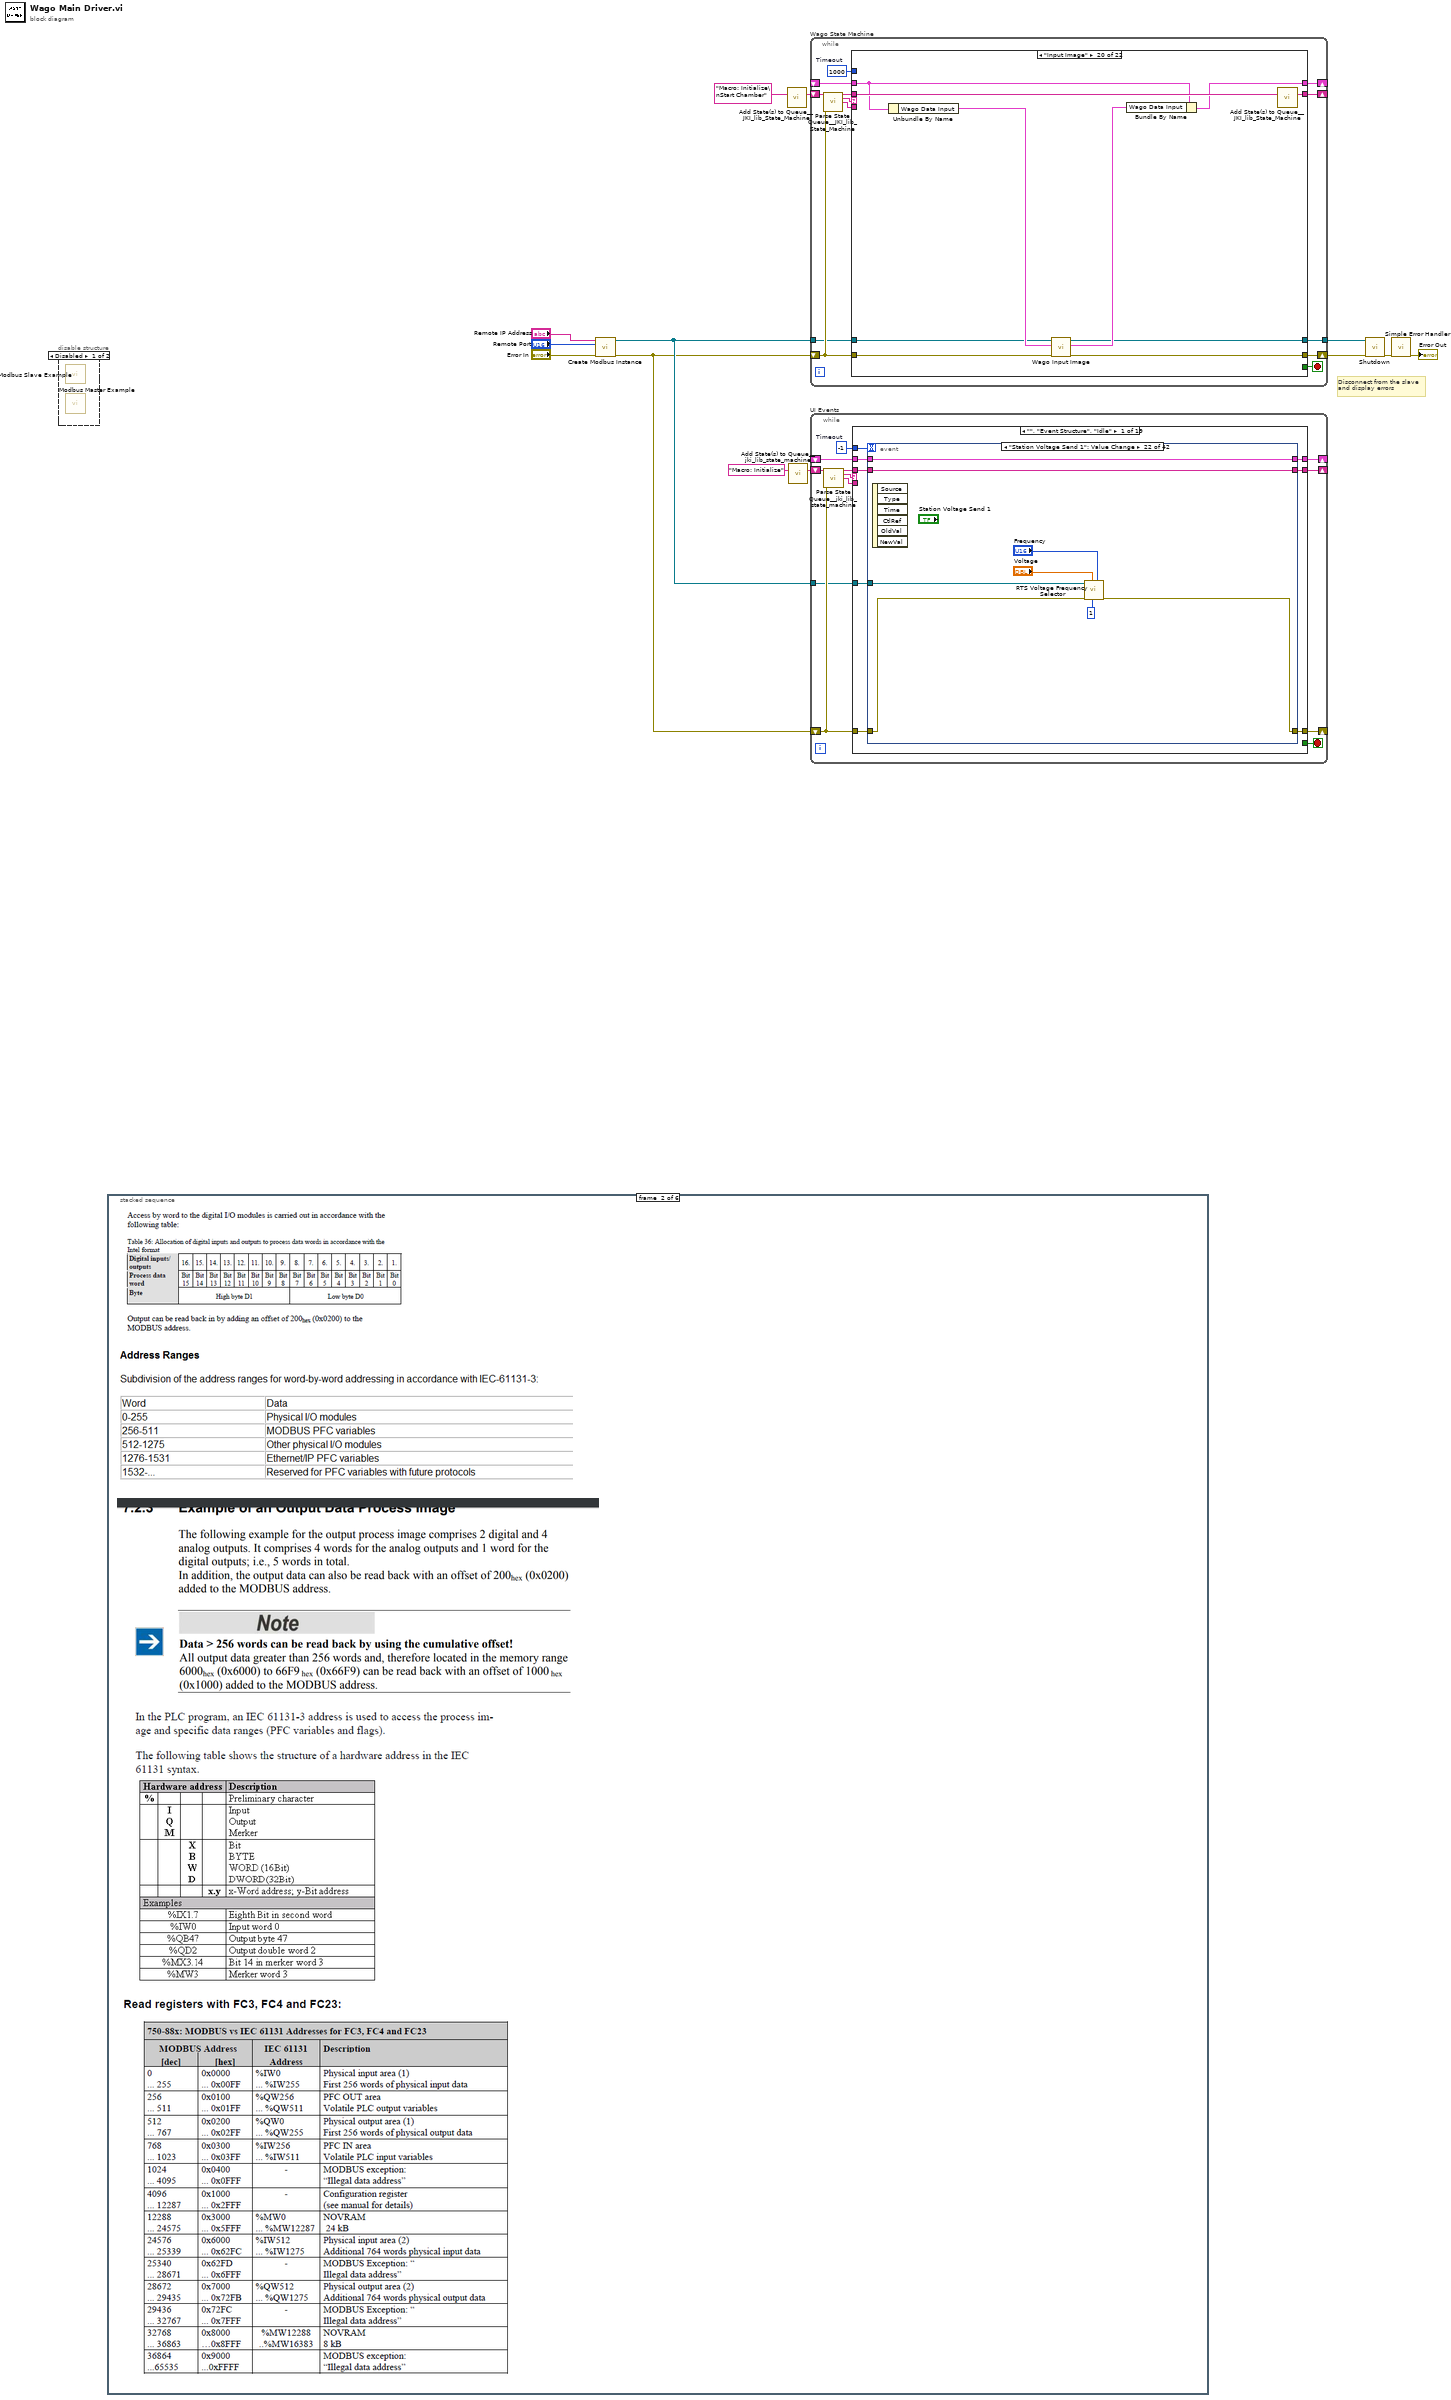
[diagram p0: block diagram]
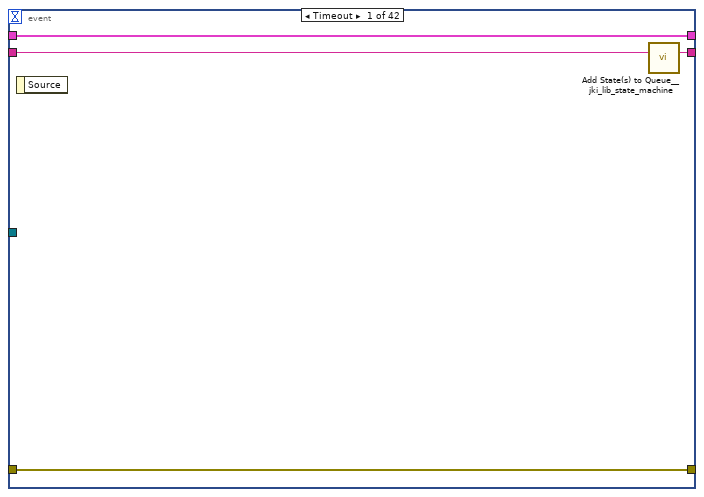
[diagram p2: hidden frame]
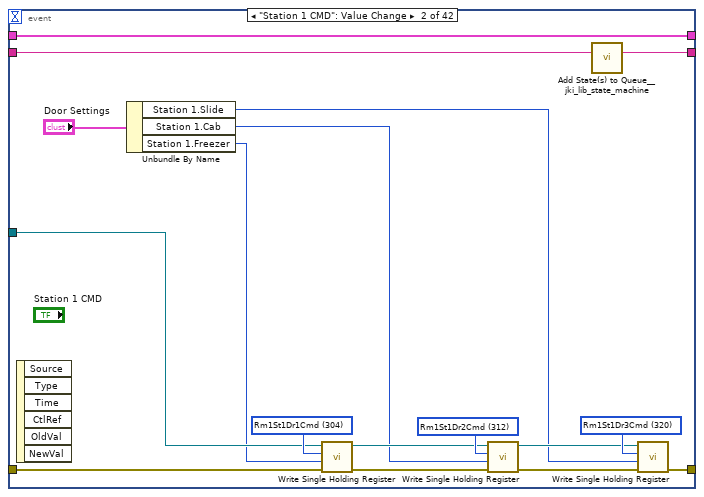
[diagram p3: hidden frame]
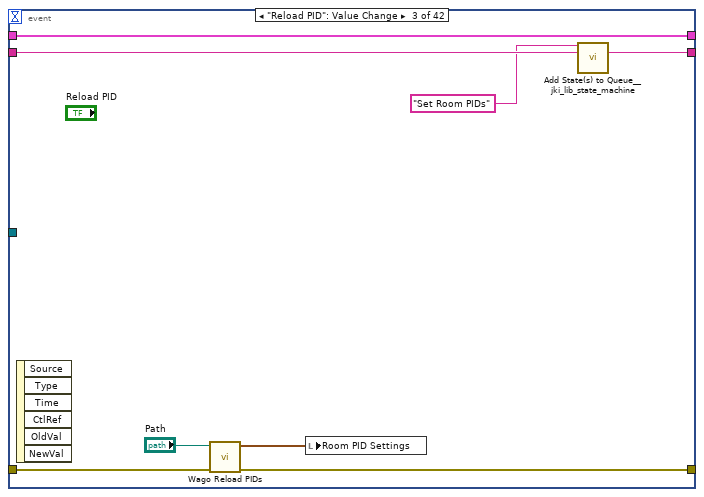
[diagram p4: hidden frame]
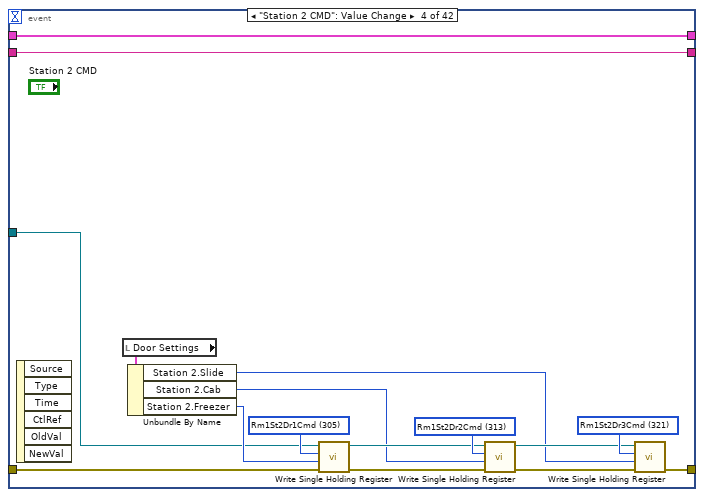
[diagram p5: hidden frame]
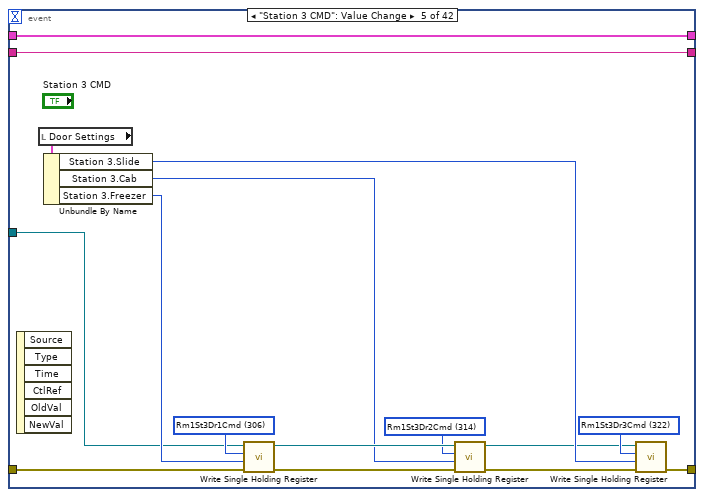
[diagram p6: hidden frame]
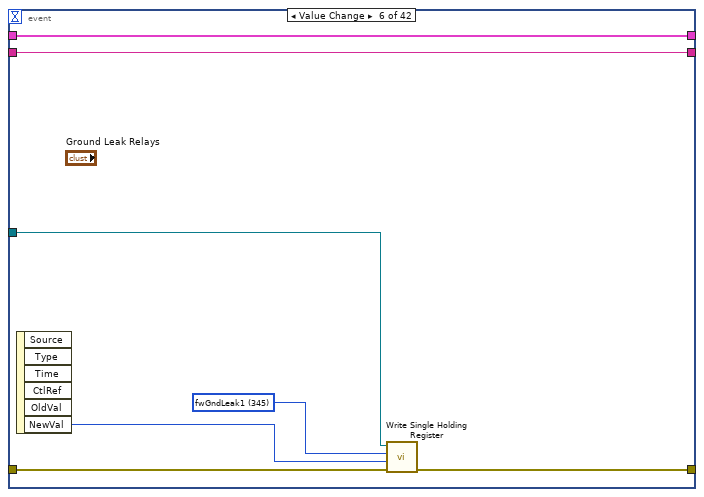
[diagram p7: hidden frame]
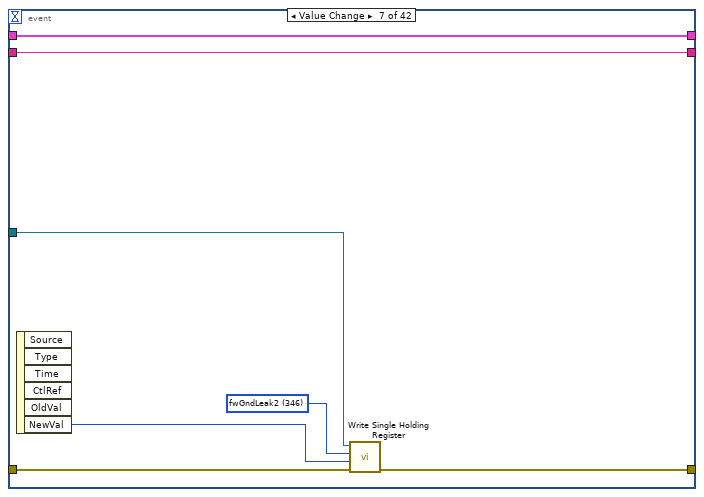
[diagram p8: hidden frame]
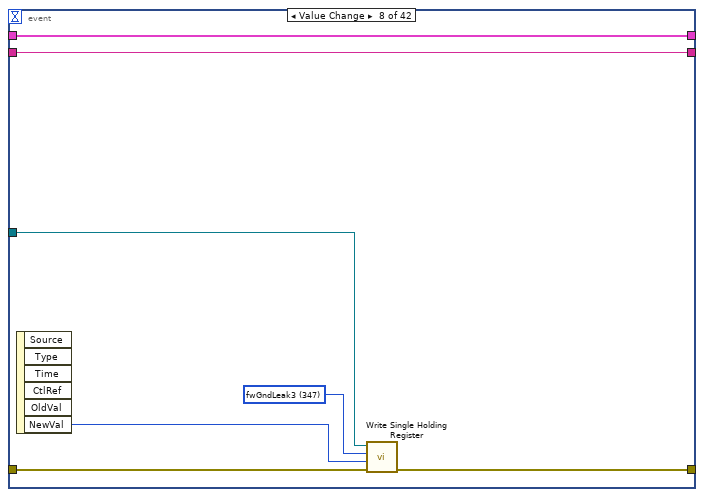
[diagram p9: hidden frame]
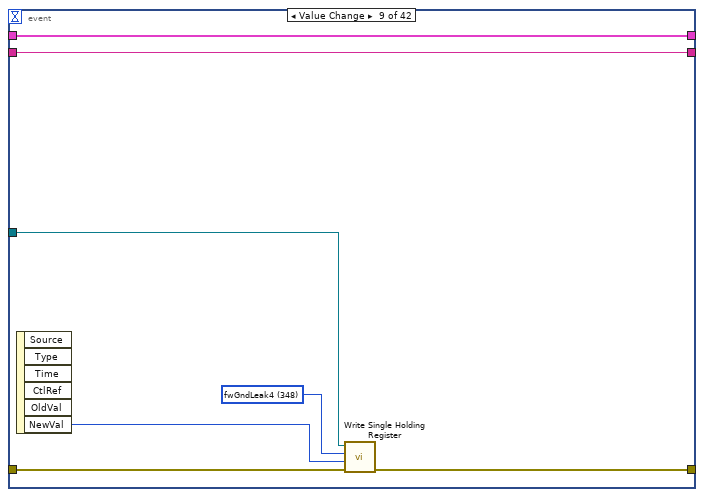
[diagram p10: hidden frame]
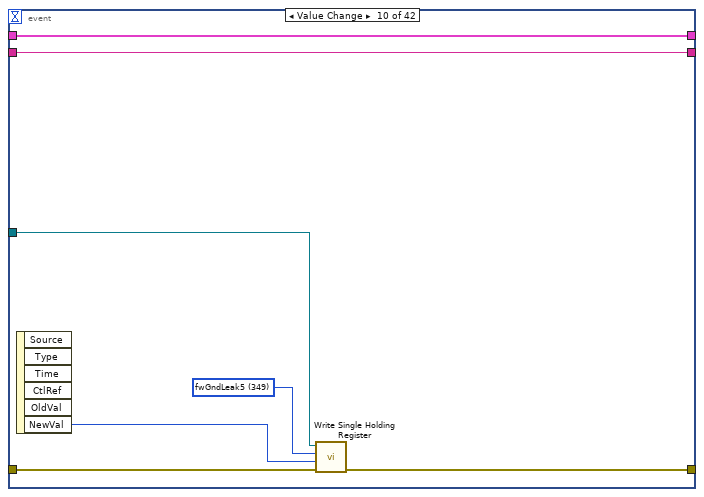
[diagram p11: hidden frame]
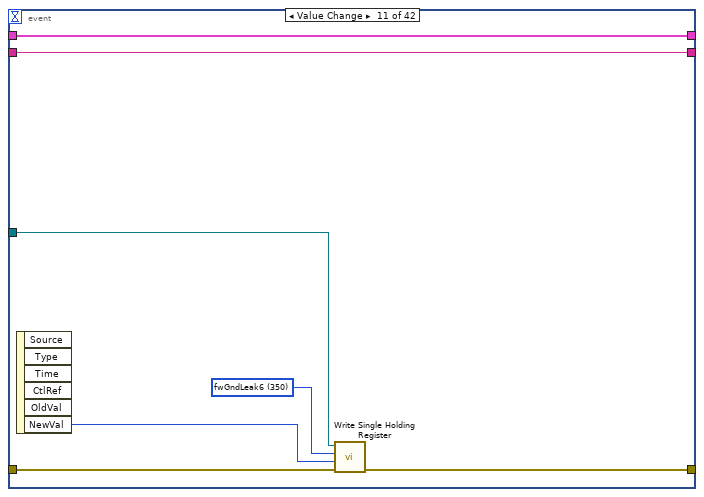
[diagram p12: hidden frame]
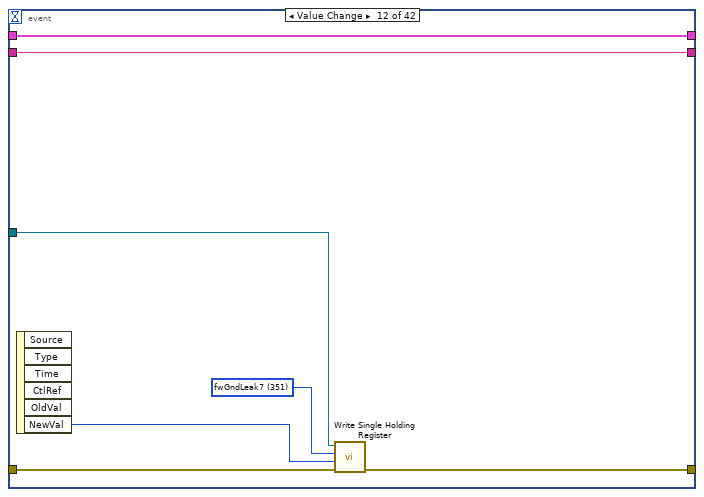
[diagram p13: hidden frame]
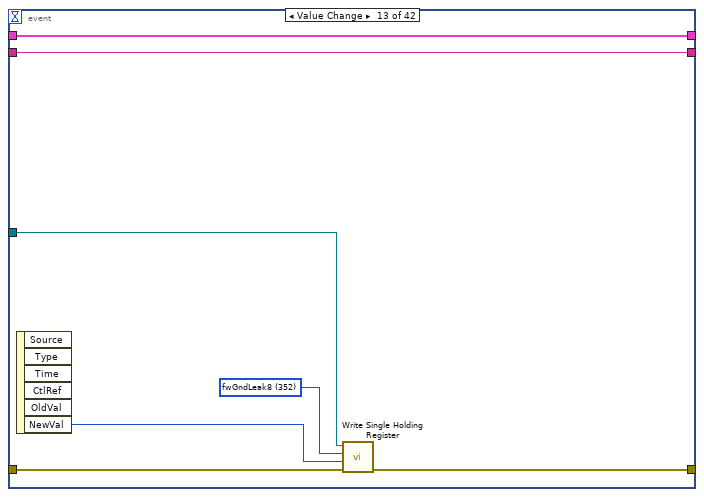
[diagram p14: hidden frame]
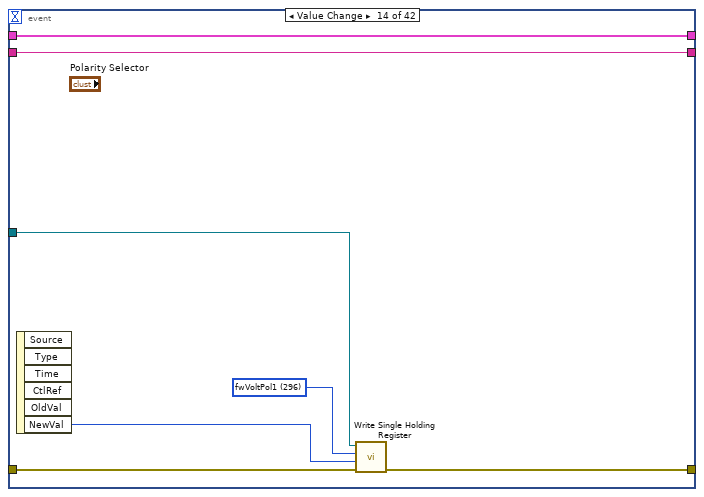
[diagram p15: hidden frame]
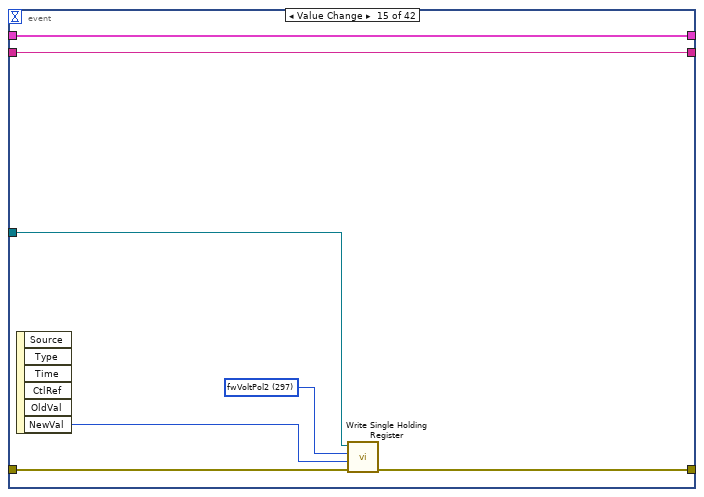
[diagram p16: hidden frame]
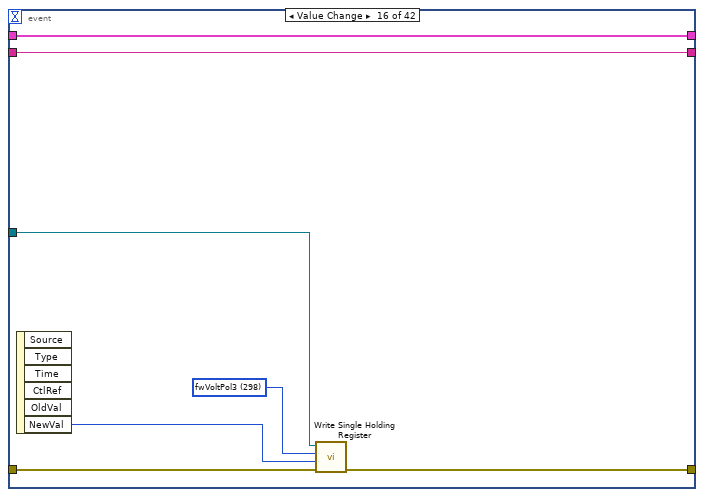
[diagram p17: hidden frame]
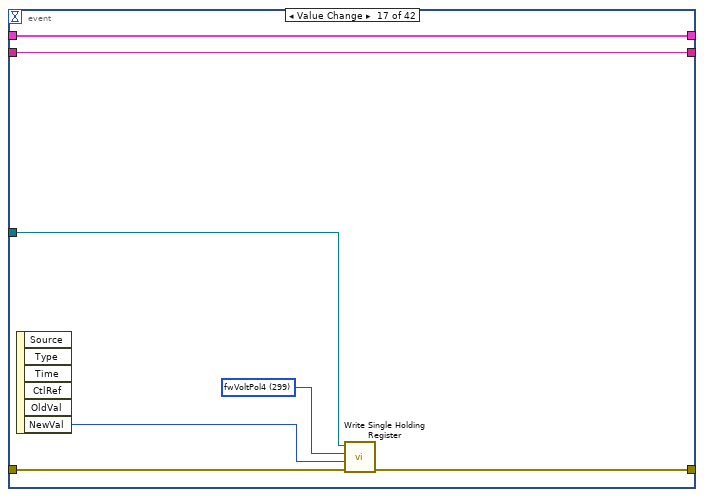
[diagram p18: hidden frame]
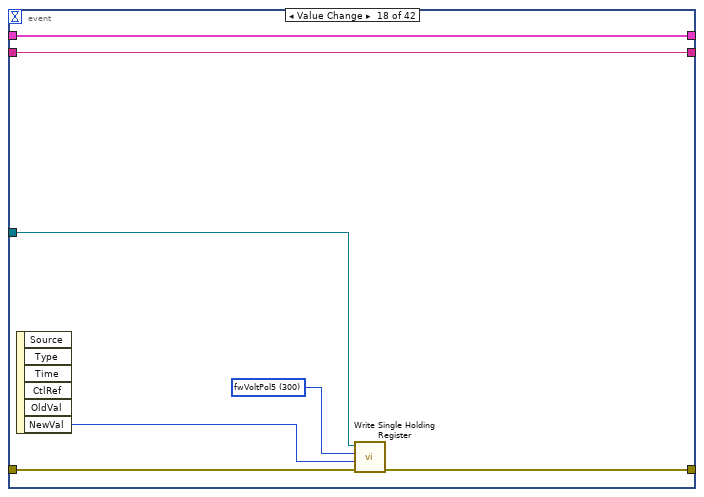
[diagram p19: hidden frame]
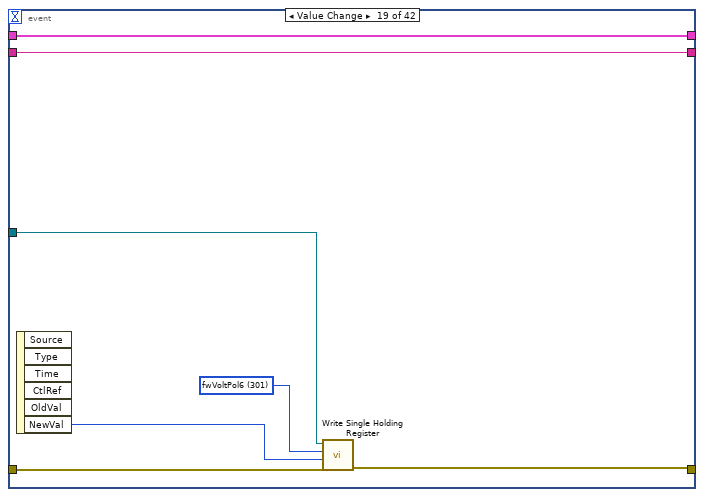
[diagram p20: hidden frame]
diagram:
  # "Disconnect from the slave\nand display errors"
  n1 = disable-structure shown="Disabled" {
    frame Disabled {
      n2 = call <vilib>:"Modbus Slave Example.vi"() -> ()  [unwired: 12 in]
      n3 = call <vilib>:"Modbus Master Example.vi"() -> ()  [unwired: 12 in]
    }
    frame Enabled {
    }
  }
  n4 = stacked-sequence {
    frame #0 {
    }
    frame #1 {
    }
    frame #2 {
    }
    frame #3 {
    }
    frame #4 {
    }
    frame #5 {
    }
  }
  n5 = call-poly <vilib>:"Create Modbus Instance.vi"("error in"="Error In", "port (502)"="Remote Port", "address"="Remote IP Address") -> ("error out"=w1:errorcluster, "TCP master instance"=w2:refnum<class "Modbus Master.lvclass">)  [unwired: 7 in]
  n6 = call <vilib>:"Add State(s) to Queue__JKI_lib_State_Machine.vi"("State(s) in (\"\")"="Macro: Initialize\nStart Chamber") -> ("States Out"=w8:string)  [unwired: 14 in]
  n7 = call <vilib>:"Add State(s) to Queue__jki_lib_state_machine.vi"("State(s) in (\"\")"="Macro: Initialize") -> ("States Out"=w4:string)  [unwired: 14 in]
  n8 = while "Wago State Machine" {
    shift-right: [w19] -> _
    shift-left: _ -> [w18]
    shift-right: [w22] -> w6
    shift-left: w1 -> [w16]
    shift-right: [w21] -> _
    shift-left: w8 -> [w23]
    tunnel: w2 -> [w15]
    tunnel: [w14] -> w5
    stop <- w20 stop-if-true
    w17 = 1000  # Timeout
    n9 = call <vilib>:"Parse State Queue__JKI_lib_State_Machine.vi"("State Queue"=w23, "Error In (no error)"=w16) -> ("Remaining States"=w25:string, "Current State"=w26:string, "Arguments"=w24:string)  [unwired: 11 in]
    n10 = case shown="\"Input Image\"" w26 {
      selector: w26 -> [_ _ w61 _ _ _ _ _ _ _ _ _ _ _ _ _ _ _ _ _ _ _]
      tunnel: w25 -> [w35 w59 w65 w84 w91 w97 w102 w109 w119 w121 w131 w136 w141 w148 w160 w187 w193 w204 w209 w219 w229 w237]
      tunnel: w24 -> [_ _ _ _ _ _ _ _ _ _ _ _ _ w143 w154 _ _ _ _ _ _ _]
      tunnel: w18 -> [w33 w56 w63 w75 w88 w95 w99 _ w120 w122 w126 w133 w139 w146 w156 w184 w190 w201 w206 w214 w224 w232]
      tunnel: [w32 w57 w67 w81 errorcluster {"status"=FALSE, "code"=0, "source"=""} ("error out") w94 w100 w106 w110 w124 w127 w134 w138 w144 w157 w185 w191 w202 w207 w216 w226 w234] -> w22
      tunnel: w16 -> [w31 w57 w66 w81 w87 w94 w100 w106 w111 w124 w128 w134 w138 w145 w158 w185 w191 w202 w207 w217 w227 w234]
      tunnel: [w34 w58 w64 w83 w90 w96 w101 w108 w119 w121 w130 w135 w140 w147 w159 w186 w192 w203 w208 w218 w228 w236] -> w21
      tunnel: [_ _ _ _ _ TRUE _ _ _ _ _ _ _ _ _ _ _ _ _ _ _ _] -> w20
      tunnel: [w30 w56 w63 w82 w88 w95 w99 w107 w120 w122 w126 w133 w139 w146 w156 w184 w190 w201 w206 w213 w223 w232] -> w19
      tunnel: w17 -> [w29 _ _ _ _ _ _ _ _ _ _ _ _ _ _ _ _ _ _ _ _ _]
      tunnel: w15 -> [w28 w55 w60 w72 w85 w92 w98 w103 w113 w123 w125 w132 w137 w142 w153 w183 w188 w194 w205 w211 w221 w235]
      tunnel: [w27 w55 w60 w72 w85 w92 w98 w103 w112 w123 w125 w132 w137 w142 w153 w183 w188 w194 w205 w210 w220 w235] -> w14
      frame "", "Event Structure", "Idle" {
        # "executes when the state queue is empty"
        n11 = event shown="[1] \"OK\": Value Change" {
          selector: _ -> [_ _ _]
          dyn-events: _ -> [_ _ _]
          timeout: w29 -> [_ _ _]
          tunnel: w35 -> [w41 w47 w54]
          tunnel: [w40 w46 w53] -> w34
          tunnel: w33 -> [w38 w44 w51]
          tunnel: [w39 w45 w52] -> w32
          tunnel: w31 -> [w39 w45 w52]
          tunnel: [w38 w44 w51] -> w30
          tunnel: [w36 w42 w48] -> w27
          tunnel: w28 -> [w36 w42 w48]
          event Timeout {
            n12 = event-data() -> ()  [unwired: 1 in, 1 out]
            n13 = call <vilib>:"Add State(s) to Queue__JKI_lib_State_Machine.vi"("State(s) in Front (\"\")"="Input Image\nOutput Image\nOutput Data", "State(s) in (\"\")"=w41) -> ("States Out"=w40:string)  [unwired: 13 in]
          }
          event "OK": Value Change {
            n14 = event-data() -> ()  [unwired: 1 in, 1 out]
            n15 = call <vilib>:"Add State(s) to Queue__JKI_lib_State_Machine.vi"("State(s) in Front (\"\")"="Macro: Exit", "State(s) in (\"\")"=w47) -> ("States Out"=w46:string)  [unwired: 13 in]
          }
          event Panel Close? {
            # "Discard the event because we'll close the front panel ourselves in Macro: Exit"
            # "Close Panel button (pressed) Event\n(this executes Macro: Exit to terminate the VI)"
            n16 = event-data() -> ()  [unwired: 1 in, 1 out]
            n17 = event-data("Discard?"=TRUE) -> ()  [unwired: 1 in, 1 out]
            n18 = call <vilib>:"Add State(s) to Queue__JKI_lib_State_Machine.vi"("State(s) in Front (\"\")"="Macro: Exit", "State(s) in (\"\")"=w54) -> ("States Out"=w53:string)  [unwired: 13 in]
          }
        }
      }
      frame "---------- Core ----------" {
        # "Do not put any code in this frame.\n(it is a separator no-op)"
        n19 = call <vilib>:"Add State(s) to Queue__JKI_lib_State_Machine.vi"("State(s) in (\"\")"=w59) -> ("States Out"=w58:string)  [unwired: 14 in]
      }
      frame Default {
        w70 = 42 items=["No error", "Argument error", "Memory is full", "Out of zone", "End of file", "File already open", "Generic file I/O error", "File not found", "File permission error", "Disk is full", "Duplicate path", "Too many files open", "System feature not enabled", "Resource file not found", "Cannot add resource", "Resource not found", "Image not found", "Image memory error", "Pen does not exist", "Config type invalid", "Config token not found", "Config parse error", "Config memory error", "Bad external code format", "Bad external code offset", "External code not present", "Null window", "Destroy window error", "Null menu", "Print aborted", "Bad print record", "Print driver error", "Windows error during printing", "Memory error during printing", "Print dialog error", "Generic print error", "Invalid device refnum", "Device not found", "Device parameter error", "Device unit error", "Cannot open device", "Device call aborted", "Generic error", "Cancelled by user", "Object ID too low", "Object ID too high", "Object not in heap", "Unknown heap", "Unknown object (invalid DefProc)", "Unknown object (DefProc not in table)", "Message out of range", "Invalid (null) method", "Unknown message", "Manager call not supported", "Bad address", "Network operation in progress", "Network operation timed out", "Connection is busy", "Network attribute not supported", "Network error", "Address in use", "System out of memory", "Connection aborted", "Connection refused", "Not connected", "Already connected", "Connection closed", "Initialization error (interapplication manager)", "Bad occurrence", "Wait on unbound occurrence handler", "Occurrence queue overflow", "Datalog type conflict", "Unused", "Unrecognized type (interapplication manager)", "Memory corrupt", "Failed to make temporary DLL", "Old CIN version", "Drag socket not found", "Failed to load drop-object", "Failed to register OLE object", "Failed to release OLE object", "Format specifier type mismatch", "Unknown format specifier", "Too few format specifiers", "Too many format specifiers", "Scan failed", "Newer CIN version", "Error converting to variant", "Runtime menu error", "Password tampered", "Variant attribute not found", "Incompatible variant data type", "Event data is not available", "Event Store is not present", "Occurrence is not found", "Event Queue is not created", "Event info is not available", "Refnum passed is NULL", "Error retrieving Class GUID", "Error retrieving CoClass GUID", "Error retrieving TypeLib GUID.", "Bad built application magic bytes.", "Specific driver is different from the specific driver associated with the Logical Name.", "There is no session opened to the class driver.", "Max Error", "MAX - Error with config objects", "MAX - Error loading configuration", "MAX - Group not supported"]
        # "Current State"
        # "Do not delete, rename, or modify this frame.\n(this is used to capture unhandled states and typos)"
        # "Handle mistyped state name (developer tool)"
        n20 = Format Into String(format string="Software Exception: Unhandled State \"%s\"." ("message"), error in=w66, w61) -> (resulting string=w69:string, error out=w68:errorcluster)  [unwired: 1 in]
        n21 = call <vilib>:"Error Cluster From Error Code.vi"("show call chain? (False)"=TRUE, "error in (no error)"=w68, "error message (\"\")"=w69, "error code (0)"=w70) -> ("error out"=w67:errorcluster)  [unwired: 5 in]
        n22 = call <vilib>:"Add State(s) to Queue__JKI_lib_State_Machine.vi"("State(s) in (\"\")"=w65) -> ("States Out"=w64:string)  [unwired: 14 in]
      }
      frame "Initialize Core Data" {
        # "Do not delete, rename, or modify this frame.\n(this is used to determine panel behavior on exit)"
        # "originally closed?"
        # "exe?"
        # "If panel starts closed or is an EXE, then close it when we exit"
        n23 = property class="VI"() -> ("Front Panel.Open"=w80:bool)  [unwired: 2 in, 2 out]
        n24 = property class="App"() -> ("App.Kind"=w79:T23)  [unwired: 2 in, 2 out]
        n25 = control-ref of="Current VI Reference"() -> (w73:refnum<vi>)
        n26 = Not(x=w80) -> (.not. x?=w77:bool)
        n27 = Equal?(x=w79, y=T23."Run Time System" ("Application:Kind")) -> (x = y?=w76:bool)
        n28 = Or(x=w77, y=w76) -> (x .or. y?=w74:bool)
        n29 = Bundle By Name(cluster=w75, "Core.Current VI Reference"=w73, "Core.Close Panel on Exit?"=w74) -> (w82:T25)
        n30 = call <vilib>:"Add State(s) to Queue__JKI_lib_State_Machine.vi"("State(s) in (\"\")"=w84) -> ("States Out"=w83:string)  [unwired: 14 in]
      }
      frame "Error Handler" {
        # "Unhandled Error -- Display it"
        # "Handle any errors here.\nYou can also output any states to clean-up after errors occur"
        # "Clear error"
        n31 = call <vilib>:"General Error Handler.vi"("error in (no error)"=w87) -> ()  [unwired: 10 in, 5 out]
        n32 = call <vilib>:"Add State(s) to Queue__JKI_lib_State_Machine.vi"("State(s) in Front (\"\")"="/* Post Error States", "State(s) in (\"\")"=w91) -> ("States Out"=w90:string)  [unwired: 13 in]
      }
      frame "Exit" {
        # "Do not put any code in this frame.\n(No errors that occur here will be handled.)"
        n33 = call <vilib>:"Add State(s) to Queue__JKI_lib_State_Machine.vi"("State(s) in (\"\")"=w97) -> ("States Out"=w96:string)  [unwired: 14 in]
      }
      frame "---------- Data ----------" {
        # "Do not put any code in this frame.\n(It is a separator no-op. You can make a copy of this frame to create a new Data frame)"
        n34 = call <vilib>:"Add State(s) to Queue__JKI_lib_State_Machine.vi"("State(s) in (\"\")"=w102) -> ("States Out"=w101:string)  [unwired: 14 in]
      }
      frame "Data: Initialize" {
        w105 = T26 {"Current VI Reference"=refnum, "Close Panel on Exit?"=FALSE}  # Core
        # "Initialize the shift-register data, here.\n(data names are defined by what you wire into the bundle function)"
        n35 = Bundle("Core"=w105, "Wago Data Input"="Wago Data Input") -> (w107:T25)  [unwired: 1 in]
        n36 = call <vilib>:"Add State(s) to Queue__JKI_lib_State_Machine.vi"("State(s) in (\"\")"=w109) -> ("States Out"=w108:string)  [unwired: 14 in]
      }
      frame "Start Chamber" {
        w114 = u16 1 ("register to write")
        w117 = T27 332 items=["fwS1Volt1"=0, "fwS1Volt2"=1, "fwS2Volt1"=2, "fwS2Volt2"=3, "fwS3Volt1"=4, "fwS3Volt2"=5, "fwS4Volt1"=6, "fwS4Volt2"=7, "fwS5Volt1"=8, "fwS5Volt2"=9, "fwS6Volt1"=10, "fwS6Volt2 "=11, "fwS7Volt1"=12, "fwS7Volt2"=13, "fwS8Volt1"=14, "fwS8Volt2"=15, "fwRoomHum"=16, "fwRoomTemp"=17, "fwAISpare1"=18, "fwAISpare2"=19, "fwSuppTemp"=20, "fwCoolTemp"=21, "fwDehumTemp"=22, "fwUnused"=23, "Bool Inputs"=24, "gwVoltRate1"=256, "gwVoltRate2"=257, "gwVoltRate3"=258, "gwVoltRate4"=259, "gwVoltRate5"=260, "gwVoltRate6"=261, "gwVoltRate7"=262, "gwVoltRate8"=263, "gwVoltWindow5/1"=264, "gwVoltWindow6/2"=265, "gwVoltWindow7/3"=266, "gwVoltWindow8/4"=267, "fwVoltSet1"=272, "fwVoltSet2"=273, "fwVoltSet3"=274, "fwVoltSet4"=275, "fwVoltSet5"=276, "fwVoltSet6"=277, "fwVoltSet7"=278, "fwVoltSet8"=279, "fwVoltRng1"=280, "fwVoltRng2"=281, "fwVoltRng3"=282, "fwVoltRng4"=283, "fwVoltRng5"=284, "fwVoltRng6"=285, "fwVoltRng7"=286, "fwVoltRng8"=287, "fwVoltPol1"=296, "fwVoltPol2"=297, "fwVoltPol3"=298, "fwVoltPol4"=299, "fwVoltPol5"=300, "fwVoltPol6"=301, "fwVoltPol7"=302, "fwVoltPol8"=303, "Rm1St1Dr1Cmd"=304, "Rm1St2Dr1Cmd"=305, "Rm1St3Dr1Cmd"=306, "Rm1St4Dr1Cmd"=307, "Rm1St5Dr1Cmd"=308, "Rm1St6Dr1Cmd"=309, "Rm1St7Dr1Cmd"=310, "Rm1St8Dr1Cmd"=311, "Rm1St1Dr2Cmd"=312, "Rm1St2Dr2Cmd"=313, "Rm1St3Dr2Cmd"=314, "Rm1St4Dr2Cmd"=315, "Rm1St5Dr2Cmd"=316, "Rm1St6Dr2Cmd"=317, "Rm1St7Dr2Cmd"=318, "Rm1St8Dr2Cmd"=319, "Rm1St1Dr3Cmd"=320, "Rm1St2Dr3Cmd"=321, "Rm1St3Dr3Cmd"=322, "Rm1St4Dr3Cmd"=323, "Rm1St5Dr3Cmd"=324, "Rm1St6Dr3Cmd"=325, "Rm1St7Dr3Cmd"=326, "Rm1St8Dr3Cmd"=327, "fwRmTempSP"=328, "fwRmHumSP"=329, "fwCoolTempSP"=330, "fwDehumTempSP"=331, "fwRmRun"=332, "fwRmOk"=333, "fwTesting"=334, "fwRmDryP"=335, "fwRmDryI"=336, "fwRmHumP"=337, "fwRmHumI"=338, "fwRmHeatP"=339, "fwRmHeatI"=340, "fwCoolTempP"=341, "fwCoolTempI"=342, "fwDehumTempP"=343, "fwDehumTempI"=344, "fwGndLeak1"=345, "fwGndLeak2"=346, "fwGndLeak3"=347, "fwGndLeak4"=348, "fwGndLeak5"=349, "fwGndLeak6"=350, "fwGndLeak7"=351, "fwGndLeak8"=352, "Rm1OpenerCmd"=353] ("Ring")
        w118 = T27 333 items=["fwS1Volt1"=0, "fwS1Volt2"=1, "fwS2Volt1"=2, "fwS2Volt2"=3, "fwS3Volt1"=4, "fwS3Volt2"=5, "fwS4Volt1"=6, "fwS4Volt2"=7, "fwS5Volt1"=8, "fwS5Volt2"=9, "fwS6Volt1"=10, "fwS6Volt2 "=11, "fwS7Volt1"=12, "fwS7Volt2"=13, "fwS8Volt1"=14, "fwS8Volt2"=15, "fwRoomHum"=16, "fwRoomTemp"=17, "fwAISpare1"=18, "fwAISpare2"=19, "fwSuppTemp"=20, "fwCoolTemp"=21, "fwDehumTemp"=22, "fwUnused"=23, "Bool Inputs"=24, "gwVoltRate1"=256, "gwVoltRate2"=257, "gwVoltRate3"=258, "gwVoltRate4"=259, "gwVoltRate5"=260, "gwVoltRate6"=261, "gwVoltRate7"=262, "gwVoltRate8"=263, "gwVoltWindow5/1"=264, "gwVoltWindow6/2"=265, "gwVoltWindow7/3"=266, "gwVoltWindow8/4"=267, "fwVoltSet1"=272, "fwVoltSet2"=273, "fwVoltSet3"=274, "fwVoltSet4"=275, "fwVoltSet5"=276, "fwVoltSet6"=277, "fwVoltSet7"=278, "fwVoltSet8"=279, "fwVoltRng1"=280, "fwVoltRng2"=281, "fwVoltRng3"=282, "fwVoltRng4"=283, "fwVoltRng5"=284, "fwVoltRng6"=285, "fwVoltRng7"=286, "fwVoltRng8"=287, "fwVoltPol1"=296, "fwVoltPol2"=297, "fwVoltPol3"=298, "fwVoltPol4"=299, "fwVoltPol5"=300, "fwVoltPol6"=301, "fwVoltPol7"=302, "fwVoltPol8"=303, "Rm1St1Dr1Cmd"=304, "Rm1St2Dr1Cmd"=305, "Rm1St3Dr1Cmd"=306, "Rm1St4Dr1Cmd"=307, "Rm1St5Dr1Cmd"=308, "Rm1St6Dr1Cmd"=309, "Rm1St7Dr1Cmd"=310, "Rm1St8Dr1Cmd"=311, "Rm1St1Dr2Cmd"=312, "Rm1St2Dr2Cmd"=313, "Rm1St3Dr2Cmd"=314, "Rm1St4Dr2Cmd"=315, "Rm1St5Dr2Cmd"=316, "Rm1St6Dr2Cmd"=317, "Rm1St7Dr2Cmd"=318, "Rm1St8Dr2Cmd"=319, "Rm1St1Dr3Cmd"=320, "Rm1St2Dr3Cmd"=321, "Rm1St3Dr3Cmd"=322, "Rm1St4Dr3Cmd"=323, "Rm1St5Dr3Cmd"=324, "Rm1St6Dr3Cmd"=325, "Rm1St7Dr3Cmd"=326, "Rm1St8Dr3Cmd"=327, "fwRmTempSP"=328, "fwRmHumSP"=329, "fwCoolTempSP"=330, "fwDehumTempSP"=331, "fwRmRun"=332, "fwRmOk"=333, "fwTesting"=334, "fwRmDryP"=335, "fwRmDryI"=336, "fwRmHumP"=337, "fwRmHumI"=338, "fwRmHeatP"=339, "fwRmHeatI"=340, "fwCoolTempP"=341, "fwCoolTempI"=342, "fwDehumTempP"=343, "fwDehumTempI"=344, "fwGndLeak1"=345, "fwGndLeak2"=346, "fwGndLeak3"=347, "fwGndLeak4"=348, "fwGndLeak5"=349, "fwGndLeak6"=350, "fwGndLeak7"=351, "fwGndLeak8"=352, "Rm1OpenerCmd"=353] ("Ring")
        n37 = call-dynamic "Write Single Holding Register.vi"("error in"=w111, "register to write"=w114, "address"=w118, "Modbus master in"=w113) -> ("error out"=w116:errorcluster, "Modbus master out"=w115:refnum<class "Modbus Master.lvclass">)  [unwired: 6 in]
        n38 = call-dynamic "Write Single Holding Register.vi"("error in"=w116, "register to write"=w114, "address"=w117, "Modbus master in"=w115) -> ("error out"=w110:errorcluster, "Modbus master out"=w112:refnum<class "Modbus Master.lvclass">)  [unwired: 6 in]
      }
      frame "Load Chamber PIDs" {
        # "Initialize the shift-register data, here.\n(data names are defined by what you wire into the bundle function)"
      }
      frame "Data: Cleanup" {
        # "Cleanup any data and references, here.\n(this is called automatically, by the Macro: Exit)"
        n39 = Unbundle By Name(w126) -> ("Core.Current VI Reference"=w129:refnum<vi>)
        n40 = Close Reference(reference=w129, error in (no error)=w128) -> (error out=w127:errorcluster)
        n41 = call <vilib>:"Add State(s) to Queue__JKI_lib_State_Machine.vi"("State(s) in (\"\")"=w131) -> ("States Out"=w130:string)  [unwired: 14 in]
      }
      frame "---------- UI ----------" {
        # "Do not put any code in this frame.\n(It is a separator no-op. You can make a copy of this frame to create a new UI frame)"
        n42 = call <vilib>:"Add State(s) to Queue__JKI_lib_State_Machine.vi"("State(s) in (\"\")"=w136) -> ("States Out"=w135:string)  [unwired: 14 in]
      }
      frame "UI: Initialize" {
        # "Start the chamber"
        n43 = call <vilib>:"Add State(s) to Queue__JKI_lib_State_Machine.vi"("State(s) in (\"\")"=w141) -> ("States Out"=w140:string)  [unwired: 14 in]
      }
      frame "UI: Cursor Set" {
        # "Argument"
        # "Set and Unset Cursor Busy.\n(Usage: \"UI: Cursor Set >> Busy|Idle\")"
        n44 = case shown="\"Idle\", Default" w143 {
          tunnel: w145 -> [w150 w152]
          tunnel: [w149 w151] -> w144
          frame "Idle", Default {
            n45 = call <vilib>:"Unset Busy.vi"("error in (no error)"=w150) -> ("error out"=w149:errorcluster)  [unwired: 10 in]
          }
          frame "Busy" {
            n46 = call <vilib>:"Set Busy.vi"("error in (no error)"=w152) -> ("error out"=w151:errorcluster)  [unwired: 9 in, 1 out]
          }
        }
        n47 = call <vilib>:"Add State(s) to Queue__JKI_lib_State_Machine.vi"("State(s) in (\"\")"=w148) -> ("States Out"=w147:string)  [unwired: 14 in]
      }
      frame "UI: Front Panel State" {
        # "Argument"
        # "Set Front Panel Open or Closed\n(Usage: \"UI: Front Panel State >> Open|Close\")"
        n48 = Unbundle By Name(w156) -> ("Core.Current VI Reference"=w155:refnum<vi>)
        n49 = case shown="\"Open\", Default" w154 {
          tunnel: w158 -> [w164 w177]
          tunnel: [w166 w178] -> w157
          tunnel: w155 -> [w165 w175]
          frame "Open", Default {
            n50 = property class="VI"(reference=w165, error in=w164) -> (reference out=w162:refnum<vi>, error out=w163:errorcluster, "Front Panel.Open"=w161:bool)
            n51 = case shown="False" w161 {
              tunnel: [w169 w172] -> w166
              tunnel: w163 -> [w168 w172]
              tunnel: w162 -> [w167 _]
              frame False {
                n52 = invoke class="VI" method="FP.Open"(reference=w167, error in=w168, "Activate"=TRUE, "State"=T24."Standard") -> (error out=w169:errorcluster)  [unwired: 1 in, 4 out]
              }
              frame True {
              }
            }
          }
          frame "Close" {
            n53 = property class="VI"(reference=w175, error in=w177) -> (reference out=w174:refnum<vi>, error out=w176:errorcluster, "Front Panel.Open"=w173:bool)
            n54 = case shown="True" w173 {
              tunnel: [w179 w182] -> w178
              tunnel: w176 -> [w179 w181]
              tunnel: w174 -> [_ w180]
              frame False {
              }
              frame True {
                n55 = invoke class="VI" method="FP.Close"(reference=w180, error in=w181) -> (error out=w182:errorcluster)  [unwired: 1 in, 2 out]
              }
            }
          }
        }
        n56 = call <vilib>:"Add State(s) to Queue__JKI_lib_State_Machine.vi"("State(s) in (\"\")"=w160) -> ("States Out"=w159:string)  [unwired: 14 in]
      }
      frame "---------- Macro ----------" {
        # "Do not put any code in this frame.\n(It is a separator no-op. You can make a copy of this frame to create a new Macro frame)"
        n57 = call <vilib>:"Add State(s) to Queue__JKI_lib_State_Machine.vi"("State(s) in (\"\")"=w187) -> ("States Out"=w186:string)  [unwired: 14 in]
      }
      frame "Macro: Initialize" {
        w189 = "Data: Initialize\nInitialize Core Data\nUI: Initialize\nUI: Front Panel State >> Open"  # Data: Initialize Initialize Core Data UI: Initialize UI: Front Panel State >> Open
        # "Initialization Macro\n(This is called once, when the VI starts)"
        n58 = call <vilib>:"Add State(s) to Queue__JKI_lib_State_Machine.vi"("State(s) in Front (\"\")"=w189, "State(s) in (\"\")"=w193) -> ("States Out"=w192:string)  [unwired: 13 in]
      }
      frame "Macro: Exit" {
        # "Exit Macro\n(This is called once, when the VI exits)"
        n59 = Unbundle By Name(w201) -> ("Core.Close Panel on Exit?"=w200:bool)
        n60 = Select(t="UI: Front Panel State >> Close", s=w200, f="") -> (s? t:f=w197:string)
        n61 = call <vilib>:"Add State(s) to Queue__JKI_lib_State_Machine.vi"("State(s) in (\"\")"=w197, "State(s) at Back (\"\")"="Data: Cleanup\nExit") -> ("States Out"=w195:string)  [unwired: 13 in]
        n62 = call <vilib>:"Add State(s) to Queue__JKI_lib_State_Machine.vi"("State(s) in Front (\"\")"=w195, "State(s) in (\"\")"=w204) -> ("States Out"=w203:string)  [unwired: 13 in]
      }
      frame "---------- New Category ----------" {
        # "Template Separator\n(You can make a copy of, or modify, this frame)"
        n63 = call <vilib>:"Add State(s) to Queue__JKI_lib_State_Machine.vi"("State(s) in (\"\")"=w209) -> ("States Out"=w208:string)  [unwired: 14 in]
      }
      frame "Input Image" {
        n64 = Unbundle By Name(w214) -> ("Wago Data Input"=w215:T15)
        n65 = call "Wago Input Image.vi"("Error In"=w217, "Wago Data Input"=w215, "Modbus Master in"=w211) -> ("Error Out"=w216:errorcluster, "Wago Data Output"=w212:T15, "Modbus master out"=w210:refnum<class "Modbus Master.lvclass">)  [unwired: 6 in]
        n66 = Bundle By Name(cluster=w214, "Wago Data Input"=w212) -> (w213:T25)
        n67 = call <vilib>:"Add State(s) to Queue__JKI_lib_State_Machine.vi"("State(s) in (\"\")"=w219) -> ("States Out"=w218:string)  [unwired: 14 in]
      }
      frame "Output Image" {
        n68 = Unbundle By Name(w224) -> ("Wago Data Input"=w225:T15)
        n69 = call "Wago Output Image.vi"("error in (no error)"=w227, "Wago Data"=w225, "Modbus Master in"=w221) -> ("error out"=w226:errorcluster, "Wago Data Output"=w222:T15, "Modbus Master out"=w220:refnum<class "Modbus Master.lvclass">)  [unwired: 6 in]
        n70 = Bundle By Name(cluster=w224, "Wago Data Input"=w222) -> (w223:T25)
        n71 = call <vilib>:"Add State(s) to Queue__JKI_lib_State_Machine.vi"("State(s) in (\"\")"=w229) -> ("States Out"=w228:string)  [unwired: 14 in]
      }
      frame "Output Data" {
        n72 = Unbundle By Name(w232) -> ("Wago Data Input"=→"Wago Data Output":T15, "Wago Data Input.System Send Data"=→"System Data":string[][], "Wago Data Input.System Data To Save"=→"System Data to Save":string[][])
        n73 = call <vilib>:"Add State(s) to Queue__JKI_lib_State_Machine.vi"("State(s) in (\"\")"=w237) -> ("States Out"=w236:string)  [unwired: 14 in]
      }
    }
  }
  n74 = while "UI Events" {
    shift-right: [w242] -> _
    shift-left: _ -> [w241]
    shift-right: [w245] -> _
    shift-left: w1 -> [w239]
    shift-right: [w244] -> _
    shift-left: w4 -> [w246]
    tunnel: w2 -> [w238]
    stop <- w243 stop-if-true
    w240 = -1  # Timeout
    n75 = call <vilib>:"Parse State Queue__jki_lib_state_machine.vi"("State Queue"=w246, "Error In (no error)"=w239) -> ("Remaining States"=w248:string, "Current State"=w249:string, "Arguments"=w247:string)  [unwired: 11 in]
    n76 = case shown="\"\", \"Event Structure\", \"Idle\"" w249 {
      selector: w249 -> [_ _ w628 _ _ _ _ _ _ _ _ _ _ _ _ _ _ _ _]
      tunnel: w248 -> [w257 w627 w632 w650 w656 w661 w665 w672 w678 w682 w686 w692 w703 w729 w734 w744 w748 w755 w759]
      tunnel: w247 -> [_ _ _ _ _ _ _ _ _ _ _ w687 w697 _ _ _ _ _ _]
      tunnel: w241 -> [w255 w624 w630 w641 w653 w659 w662 _ w673 w679 w684 w690 w699 w726 w731 w741 w745 w753 w756]
      tunnel: [w254 w625 w634 w647 errorcluster {"status"=FALSE, "code"=0, "source"=""} ("error out") w658 w663 w669 w674 w680 w683 w688 w700 w727 w732 w742 w746 w750 w757] -> w245
      tunnel: w239 -> [w253 w625 w633 w647 w652 w658 w663 w669 w675 w680 w683 w689 w701 w727 w732 w742 w746 w751 w757]
      tunnel: [w256 w626 w631 w649 w655 w660 w664 w671 w677 w681 w685 w691 w702 w728 w733 w743 w747 w754 w758] -> w244
      tunnel: [_ _ _ _ _ TRUE _ _ _ _ _ _ _ _ _ _ _ _ _] -> w243
      tunnel: [w252 w624 w630 w648 w653 w659 w662 w670 w673 w679 w684 w690 w699 w726 w731 w741 w745 w753 w756] -> w242
      tunnel: w240 -> [w251 _ _ _ _ _ _ _ _ _ _ _ _ _ _ _ _ _ _]
      tunnel: w238 -> [w250 _ _ _ _ _ _ _ _ _ _ _ _ _ _ _ _ w749 _]
      frame "", "Event Structure", "Idle" {
        n77 = event shown="[21] \"Station Voltage Send 1\": Value Change" {
          selector: _ -> [_ _ _ _ _ _ _ _ _ _ _ _ _ _ _ _ _ _ _ _ _ _ _ _ _ _ _ _ _ _ _ _ _ _ _ _ _ _ _ _ _ _]
          dyn-events: _ -> [_ _ _ _ _ _ _ _ _ _ _ _ _ _ _ _ _ _ _ _ _ _ _ _ _ _ _ _ _ _ _ _ _ _ _ _ _ _ _ _ _ _]
          timeout: w251 -> [_ _ _ _ _ _ _ _ _ _ _ _ _ _ _ _ _ _ _ _ _ _ _ _ _ _ _ _ _ _ _ _ _ _ _ _ _ _ _ _ _ _]
          tunnel: w257 -> [w261 w263 w285 w301 w317 w324 w331 w338 w345 w352 w359 w361 w373 w380 w387 w394 w401 w408 w415 w422 w424 w437 w445 w453 w462 w469 w477 w485 w494 w509 w511 w541 w557 w563 w580 w587 w595 w600 w604 w611 w617 w623]
          tunnel: [w260 w262 w284 w301 w317 w324 w331 w338 w345 w352 w359 w361 w373 w380 w387 w394 w401 w408 w415 w422 w424 w437 w445 w453 w462 w469 w477 w485 w494 w509 w511 w541 w557 w563 w580 w587 w595 w600 w603 w611 w616 w622] -> w256
          tunnel: w255 -> [w258 w275 w286 w302 w318 w325 w332 w339 w346 w353 w360 w362 w374 w381 w388 w395 w402 w409 w416 w423 w425 w438 w446 w454 w461 w470 w478 w486 w493 w510 w512 w542 w558 w564 w581 w588 w594 w601 w606 w612 w614 w620]
          tunnel: [w259 w270 w281 w289 w309 w321 w328 w335 w342 w349 w356 w365 w370 w377 w384 w391 w398 w405 w412 w419 w429 w434 w442 w450 w458 w466 w471 w479 w487 w497 w515 w529 w545 w567 w577 w585 w591 w598 w605 w609 w615 w621] -> w254
          tunnel: w253 -> [w259 w277 w282 w292 w310 w322 w329 w336 w343 w350 w357 w366 w371 w378 w385 w392 w399 w406 w413 w420 w427 w436 w443 w451 w459 w467 w472 w480 w488 w496 w514 w528 w544 w565 w578 w586 w592 w599 w605 w610 w615 w621]
          tunnel: [w258 w275 w286 w302 w318 w325 w332 w339 w346 w353 w360 w362 w374 w381 w388 w395 w402 w409 w416 w423 w425 w438 w446 w454 w461 w470 w478 w486 w493 w510 w512 w542 w558 w564 w581 w588 w594 w601 w606 w612 w614 w620] -> w252
          tunnel: w250 -> [_ w276 _ w287 w308 w319 w327 w334 w341 w348 w355 w364 w369 w375 w382 w390 w397 w404 w411 w418 w428 w435 w441 w449 w460 w465 w475 w483 w491 w495 w513 w527 w543 w566 w576 w582 w590 w597 _ w608 _ _]
          event Timeout {
            n78 = event-data() -> ()  [unwired: 1 in, 1 out]
            n79 = call <vilib>:"Add State(s) to Queue__jki_lib_state_machine.vi"("State(s) in (\"\")"=w261) -> ("States Out"=w260:string)  [unwired: 14 in]
          }
          event "Station 1 CMD": Value Change {
            w273 = T27 320 items=["fwS1Volt1"=0, "fwS1Volt2"=1, "fwS2Volt1"=2, "fwS2Volt2"=3, "fwS3Volt1"=4, "fwS3Volt2"=5, "fwS4Volt1"=6, "fwS4Volt2"=7, "fwS5Volt1"=8, "fwS5Volt2"=9, "fwS6Volt1"=10, "fwS6Volt2 "=11, "fwS7Volt1"=12, "fwS7Volt2"=13, "fwS8Volt1"=14, "fwS8Volt2"=15, "fwRoomHum"=16, "fwRoomTemp"=17, "fwAISpare1"=18, "fwAISpare2"=19, "fwSuppTemp"=20, "fwCoolTemp"=21, "fwDehumTemp"=22, "fwUnused"=23, "Bool Inputs"=24, "gwVoltRate1"=256, "gwVoltRate2"=257, "gwVoltRate3"=258, "gwVoltRate4"=259, "gwVoltRate5"=260, "gwVoltRate6"=261, "gwVoltRate7"=262, "gwVoltRate8"=263, "gwVoltWindow5/1"=264, "gwVoltWindow6/2"=265, "gwVoltWindow7/3"=266, "gwVoltWindow8/4"=267, "fwVoltSet1"=272, "fwVoltSet2"=273, "fwVoltSet3"=274, "fwVoltSet4"=275, "fwVoltSet5"=276, "fwVoltSet6"=277, "fwVoltSet7"=278, "fwVoltSet8"=279, "fwVoltRng1"=280, "fwVoltRng2"=281, "fwVoltRng3"=282, "fwVoltRng4"=283, "fwVoltRng5"=284, "fwVoltRng6"=285, "fwVoltRng7"=286, "fwVoltRng8"=287, "fwVoltPol1"=296, "fwVoltPol2"=297, "fwVoltPol3"=298, "fwVoltPol4"=299, "fwVoltPol5"=300, "fwVoltPol6"=301, "fwVoltPol7"=302, "fwVoltPol8"=303, "Rm1St1Dr1Cmd"=304, "Rm1St2Dr1Cmd"=305, "Rm1St3Dr1Cmd"=306, "Rm1St4Dr1Cmd"=307, "Rm1St5Dr1Cmd"=308, "Rm1St6Dr1Cmd"=309, "Rm1St7Dr1Cmd"=310, "Rm1St8Dr1Cmd"=311, "Rm1St1Dr2Cmd"=312, "Rm1St2Dr2Cmd"=313, "Rm1St3Dr2Cmd"=314, "Rm1St4Dr2Cmd"=315, "Rm1St5Dr2Cmd"=316, "Rm1St6Dr2Cmd"=317, "Rm1St7Dr2Cmd"=318, "Rm1St8Dr2Cmd"=319, "Rm1St1Dr3Cmd"=320, "Rm1St2Dr3Cmd"=321, "Rm1St3Dr3Cmd"=322, "Rm1St4Dr3Cmd"=323, "Rm1St5Dr3Cmd"=324, "Rm1St6Dr3Cmd"=325, "Rm1St7Dr3Cmd"=326, "Rm1St8Dr3Cmd"=327, "fwRmTempSP"=328, "fwRmHumSP"=329, "fwCoolTempSP"=330, "fwDehumTempSP"=331, "fwRmRun"=332, "fwRmOk"=333, "fwTesting"=334, "fwRmDryP"=335, "fwRmDryI"=336, "fwRmHumP"=337, "fwRmHumI"=338, "fwRmHeatP"=339, "fwRmHeatI"=340, "fwCoolTempP"=341, "fwCoolTempI"=342, "fwDehumTempP"=343, "fwDehumTempI"=344, "fwGndLeak1"=345, "fwGndLeak2"=346, "fwGndLeak3"=347, "fwGndLeak4"=348, "fwGndLeak5"=349, "fwGndLeak6"=350, "fwGndLeak7"=351, "fwGndLeak8"=352, "Rm1OpenerCmd"=353] ("Ring")
            w274 = T27 312 items=["fwS1Volt1"=0, "fwS1Volt2"=1, "fwS2Volt1"=2, "fwS2Volt2"=3, "fwS3Volt1"=4, "fwS3Volt2"=5, "fwS4Volt1"=6, "fwS4Volt2"=7, "fwS5Volt1"=8, "fwS5Volt2"=9, "fwS6Volt1"=10, "fwS6Volt2 "=11, "fwS7Volt1"=12, "fwS7Volt2"=13, "fwS8Volt1"=14, "fwS8Volt2"=15, "fwRoomHum"=16, "fwRoomTemp"=17, "fwAISpare1"=18, "fwAISpare2"=19, "fwSuppTemp"=20, "fwCoolTemp"=21, "fwDehumTemp"=22, "fwUnused"=23, "Bool Inputs"=24, "gwVoltRate1"=256, "gwVoltRate2"=257, "gwVoltRate3"=258, "gwVoltRate4"=259, "gwVoltRate5"=260, "gwVoltRate6"=261, "gwVoltRate7"=262, "gwVoltRate8"=263, "gwVoltWindow5/1"=264, "gwVoltWindow6/2"=265, "gwVoltWindow7/3"=266, "gwVoltWindow8/4"=267, "fwVoltSet1"=272, "fwVoltSet2"=273, "fwVoltSet3"=274, "fwVoltSet4"=275, "fwVoltSet5"=276, "fwVoltSet6"=277, "fwVoltSet7"=278, "fwVoltSet8"=279, "fwVoltRng1"=280, "fwVoltRng2"=281, "fwVoltRng3"=282, "fwVoltRng4"=283, "fwVoltRng5"=284, "fwVoltRng6"=285, "fwVoltRng7"=286, "fwVoltRng8"=287, "fwVoltPol1"=296, "fwVoltPol2"=297, "fwVoltPol3"=298, "fwVoltPol4"=299, "fwVoltPol5"=300, "fwVoltPol6"=301, "fwVoltPol7"=302, "fwVoltPol8"=303, "Rm1St1Dr1Cmd"=304, "Rm1St2Dr1Cmd"=305, "Rm1St3Dr1Cmd"=306, "Rm1St4Dr1Cmd"=307, "Rm1St5Dr1Cmd"=308, "Rm1St6Dr1Cmd"=309, "Rm1St7Dr1Cmd"=310, "Rm1St8Dr1Cmd"=311, "Rm1St1Dr2Cmd"=312, "Rm1St2Dr2Cmd"=313, "Rm1St3Dr2Cmd"=314, "Rm1St4Dr2Cmd"=315, "Rm1St5Dr2Cmd"=316, "Rm1St6Dr2Cmd"=317, "Rm1St7Dr2Cmd"=318, "Rm1St8Dr2Cmd"=319, "Rm1St1Dr3Cmd"=320, "Rm1St2Dr3Cmd"=321, "Rm1St3Dr3Cmd"=322, "Rm1St4Dr3Cmd"=323, "Rm1St5Dr3Cmd"=324, "Rm1St6Dr3Cmd"=325, "Rm1St7Dr3Cmd"=326, "Rm1St8Dr3Cmd"=327, "fwRmTempSP"=328, "fwRmHumSP"=329, "fwCoolTempSP"=330, "fwDehumTempSP"=331, "fwRmRun"=332, "fwRmOk"=333, "fwTesting"=334, "fwRmDryP"=335, "fwRmDryI"=336, "fwRmHumP"=337, "fwRmHumI"=338, "fwRmHeatP"=339, "fwRmHeatI"=340, "fwCoolTempP"=341, "fwCoolTempI"=342, "fwDehumTempP"=343, "fwDehumTempI"=344, "fwGndLeak1"=345, "fwGndLeak2"=346, "fwGndLeak3"=347, "fwGndLeak4"=348, "fwGndLeak5"=349, "fwGndLeak6"=350, "fwGndLeak7"=351, "fwGndLeak8"=352, "Rm1OpenerCmd"=353] ("Ring")
            w278 = T27 304 items=["fwS1Volt1"=0, "fwS1Volt2"=1, "fwS2Volt1"=2, "fwS2Volt2"=3, "fwS3Volt1"=4, "fwS3Volt2"=5, "fwS4Volt1"=6, "fwS4Volt2"=7, "fwS5Volt1"=8, "fwS5Volt2"=9, "fwS6Volt1"=10, "fwS6Volt2 "=11, "fwS7Volt1"=12, "fwS7Volt2"=13, "fwS8Volt1"=14, "fwS8Volt2"=15, "fwRoomHum"=16, "fwRoomTemp"=17, "fwAISpare1"=18, "fwAISpare2"=19, "fwSuppTemp"=20, "fwCoolTemp"=21, "fwDehumTemp"=22, "fwUnused"=23, "Bool Inputs"=24, "gwVoltRate1"=256, "gwVoltRate2"=257, "gwVoltRate3"=258, "gwVoltRate4"=259, "gwVoltRate5"=260, "gwVoltRate6"=261, "gwVoltRate7"=262, "gwVoltRate8"=263, "gwVoltWindow5/1"=264, "gwVoltWindow6/2"=265, "gwVoltWindow7/3"=266, "gwVoltWindow8/4"=267, "fwVoltSet1"=272, "fwVoltSet2"=273, "fwVoltSet3"=274, "fwVoltSet4"=275, "fwVoltSet5"=276, "fwVoltSet6"=277, "fwVoltSet7"=278, "fwVoltSet8"=279, "fwVoltRng1"=280, "fwVoltRng2"=281, "fwVoltRng3"=282, "fwVoltRng4"=283, "fwVoltRng5"=284, "fwVoltRng6"=285, "fwVoltRng7"=286, "fwVoltRng8"=287, "fwVoltPol1"=296, "fwVoltPol2"=297, "fwVoltPol3"=298, "fwVoltPol4"=299, "fwVoltPol5"=300, "fwVoltPol6"=301, "fwVoltPol7"=302, "fwVoltPol8"=303, "Rm1St1Dr1Cmd"=304, "Rm1St2Dr1Cmd"=305, "Rm1St3Dr1Cmd"=306, "Rm1St4Dr1Cmd"=307, "Rm1St5Dr1Cmd"=308, "Rm1St6Dr1Cmd"=309, "Rm1St7Dr1Cmd"=310, "Rm1St8Dr1Cmd"=311, "Rm1St1Dr2Cmd"=312, "Rm1St2Dr2Cmd"=313, "Rm1St3Dr2Cmd"=314, "Rm1St4Dr2Cmd"=315, "Rm1St5Dr2Cmd"=316, "Rm1St6Dr2Cmd"=317, "Rm1St7Dr2Cmd"=318, "Rm1St8Dr2Cmd"=319, "Rm1St1Dr3Cmd"=320, "Rm1St2Dr3Cmd"=321, "Rm1St3Dr3Cmd"=322, "Rm1St4Dr3Cmd"=323, "Rm1St5Dr3Cmd"=324, "Rm1St6Dr3Cmd"=325, "Rm1St7Dr3Cmd"=326, "Rm1St8Dr3Cmd"=327, "fwRmTempSP"=328, "fwRmHumSP"=329, "fwCoolTempSP"=330, "fwDehumTempSP"=331, "fwRmRun"=332, "fwRmOk"=333, "fwTesting"=334, "fwRmDryP"=335, "fwRmDryI"=336, "fwRmHumP"=337, "fwRmHumI"=338, "fwRmHeatP"=339, "fwRmHeatI"=340, "fwCoolTempP"=341, "fwCoolTempI"=342, "fwDehumTempP"=343, "fwDehumTempI"=344, "fwGndLeak1"=345, "fwGndLeak2"=346, "fwGndLeak3"=347, "fwGndLeak4"=348, "fwGndLeak5"=349, "fwGndLeak6"=350, "fwGndLeak7"=351, "fwGndLeak8"=352, "Rm1OpenerCmd"=353] ("Ring")
            n80 = event-data() -> ()  [unwired: 1 in, 6 out]
            n81 = Unbundle By Name("Door Settings") -> ("Station 1.Slide"=w264:T13, "Station 1.Cab"=w265:T13, "Station 1.Freezer"=w266:T13)
            n82 = call-dynamic "Write Single Holding Register.vi"("error in"=w277, "register to write"=w266, "address"=w278, "Modbus master in"=w276) -> ("error out"=w272:errorcluster, "Modbus master out"=w269:refnum<class "Modbus Master.lvclass">)  [unwired: 6 in]
            n83 = call-dynamic "Write Single Holding Register.vi"("error in"=w272, "register to write"=w265, "address"=w274, "Modbus master in"=w269) -> ("error out"=w271:errorcluster, "Modbus master out"=w268:refnum<class "Modbus Master.lvclass">)  [unwired: 6 in]
            n84 = call <vilib>:"Add State(s) to Queue__jki_lib_state_machine.vi"("State(s) in (\"\")"=w263) -> ("States Out"=w262:string)  [unwired: 14 in]
            n85 = call-dynamic "Write Single Holding Register.vi"("error in"=w271, "register to write"=w264, "address"=w273, "Modbus master in"=w268) -> ("error out"=w270:errorcluster)  [unwired: 6 in, 1 out]
          }
          event "Reload PID": Value Change {
            n86 = event-data() -> ()  [unwired: 1 in, 6 out]
            n87 = call "Wago Reload PIDs.vi"("Error In"=w282, "Path"="Path") -> ("Error Out"=w281:errorcluster, "Room PID Settings"=w280:T2)  [unwired: 8 in]
            n88 = local write "Room PID Settings"(w280) -> ()
            n89 = call <vilib>:"Add State(s) to Queue__jki_lib_state_machine.vi"("State(s) in Front (\"\")"="Set Room PIDs" ("State(s) in Front (\"\")"), "State(s) in (\"\")"=w285) -> ("States Out"=w284:string)  [unwired: 13 in]
          }
          event "Station 2 CMD": Value Change {
            w298 = T27 321 items=["fwS1Volt1"=0, "fwS1Volt2"=1, "fwS2Volt1"=2, "fwS2Volt2"=3, "fwS3Volt1"=4, "fwS3Volt2"=5, "fwS4Volt1"=6, "fwS4Volt2"=7, "fwS5Volt1"=8, "fwS5Volt2"=9, "fwS6Volt1"=10, "fwS6Volt2 "=11, "fwS7Volt1"=12, "fwS7Volt2"=13, "fwS8Volt1"=14, "fwS8Volt2"=15, "fwRoomHum"=16, "fwRoomTemp"=17, "fwAISpare1"=18, "fwAISpare2"=19, "fwSuppTemp"=20, "fwCoolTemp"=21, "fwDehumTemp"=22, "fwUnused"=23, "Bool Inputs"=24, "gwVoltRate1"=256, "gwVoltRate2"=257, "gwVoltRate3"=258, "gwVoltRate4"=259, "gwVoltRate5"=260, "gwVoltRate6"=261, "gwVoltRate7"=262, "gwVoltRate8"=263, "gwVoltWindow5/1"=264, "gwVoltWindow6/2"=265, "gwVoltWindow7/3"=266, "gwVoltWindow8/4"=267, "fwVoltSet1"=272, "fwVoltSet2"=273, "fwVoltSet3"=274, "fwVoltSet4"=275, "fwVoltSet5"=276, "fwVoltSet6"=277, "fwVoltSet7"=278, "fwVoltSet8"=279, "fwVoltRng1"=280, "fwVoltRng2"=281, "fwVoltRng3"=282, "fwVoltRng4"=283, "fwVoltRng5"=284, "fwVoltRng6"=285, "fwVoltRng7"=286, "fwVoltRng8"=287, "fwVoltPol1"=296, "fwVoltPol2"=297, "fwVoltPol3"=298, "fwVoltPol4"=299, "fwVoltPol5"=300, "fwVoltPol6"=301, "fwVoltPol7"=302, "fwVoltPol8"=303, "Rm1St1Dr1Cmd"=304, "Rm1St2Dr1Cmd"=305, "Rm1St3Dr1Cmd"=306, "Rm1St4Dr1Cmd"=307, "Rm1St5Dr1Cmd"=308, "Rm1St6Dr1Cmd"=309, "Rm1St7Dr1Cmd"=310, "Rm1St8Dr1Cmd"=311, "Rm1St1Dr2Cmd"=312, "Rm1St2Dr2Cmd"=313, "Rm1St3Dr2Cmd"=314, "Rm1St4Dr2Cmd"=315, "Rm1St5Dr2Cmd"=316, "Rm1St6Dr2Cmd"=317, "Rm1St7Dr2Cmd"=318, "Rm1St8Dr2Cmd"=319, "Rm1St1Dr3Cmd"=320, "Rm1St2Dr3Cmd"=321, "Rm1St3Dr3Cmd"=322, "Rm1St4Dr3Cmd"=323, "Rm1St5Dr3Cmd"=324, "Rm1St6Dr3Cmd"=325, "Rm1St7Dr3Cmd"=326, "Rm1St8Dr3Cmd"=327, "fwRmTempSP"=328, "fwRmHumSP"=329, "fwCoolTempSP"=330, "fwDehumTempSP"=331, "fwRmRun"=332, "fwRmOk"=333, "fwTesting"=334, "fwRmDryP"=335, "fwRmDryI"=336, "fwRmHumP"=337, "fwRmHumI"=338, "fwRmHeatP"=339, "fwRmHeatI"=340, "fwCoolTempP"=341, "fwCoolTempI"=342, "fwDehumTempP"=343, "fwDehumTempI"=344, "fwGndLeak1"=345, "fwGndLeak2"=346, "fwGndLeak3"=347, "fwGndLeak4"=348, "fwGndLeak5"=349, "fwGndLeak6"=350, "fwGndLeak7"=351, "fwGndLeak8"=352, "Rm1OpenerCmd"=353] ("Ring")
            w299 = T27 313 items=["fwS1Volt1"=0, "fwS1Volt2"=1, "fwS2Volt1"=2, "fwS2Volt2"=3, "fwS3Volt1"=4, "fwS3Volt2"=5, "fwS4Volt1"=6, "fwS4Volt2"=7, "fwS5Volt1"=8, "fwS5Volt2"=9, "fwS6Volt1"=10, "fwS6Volt2 "=11, "fwS7Volt1"=12, "fwS7Volt2"=13, "fwS8Volt1"=14, "fwS8Volt2"=15, "fwRoomHum"=16, "fwRoomTemp"=17, "fwAISpare1"=18, "fwAISpare2"=19, "fwSuppTemp"=20, "fwCoolTemp"=21, "fwDehumTemp"=22, "fwUnused"=23, "Bool Inputs"=24, "gwVoltRate1"=256, "gwVoltRate2"=257, "gwVoltRate3"=258, "gwVoltRate4"=259, "gwVoltRate5"=260, "gwVoltRate6"=261, "gwVoltRate7"=262, "gwVoltRate8"=263, "gwVoltWindow5/1"=264, "gwVoltWindow6/2"=265, "gwVoltWindow7/3"=266, "gwVoltWindow8/4"=267, "fwVoltSet1"=272, "fwVoltSet2"=273, "fwVoltSet3"=274, "fwVoltSet4"=275, "fwVoltSet5"=276, "fwVoltSet6"=277, "fwVoltSet7"=278, "fwVoltSet8"=279, "fwVoltRng1"=280, "fwVoltRng2"=281, "fwVoltRng3"=282, "fwVoltRng4"=283, "fwVoltRng5"=284, "fwVoltRng6"=285, "fwVoltRng7"=286, "fwVoltRng8"=287, "fwVoltPol1"=296, "fwVoltPol2"=297, "fwVoltPol3"=298, "fwVoltPol4"=299, "fwVoltPol5"=300, "fwVoltPol6"=301, "fwVoltPol7"=302, "fwVoltPol8"=303, "Rm1St1Dr1Cmd"=304, "Rm1St2Dr1Cmd"=305, "Rm1St3Dr1Cmd"=306, "Rm1St4Dr1Cmd"=307, "Rm1St5Dr1Cmd"=308, "Rm1St6Dr1Cmd"=309, "Rm1St7Dr1Cmd"=310, "Rm1St8Dr1Cmd"=311, "Rm1St1Dr2Cmd"=312, "Rm1St2Dr2Cmd"=313, "Rm1St3Dr2Cmd"=314, "Rm1St4Dr2Cmd"=315, "Rm1St5Dr2Cmd"=316, "Rm1St6Dr2Cmd"=317, "Rm1St7Dr2Cmd"=318, "Rm1St8Dr2Cmd"=319, "Rm1St1Dr3Cmd"=320, "Rm1St2Dr3Cmd"=321, "Rm1St3Dr3Cmd"=322, "Rm1St4Dr3Cmd"=323, "Rm1St5Dr3Cmd"=324, "Rm1St6Dr3Cmd"=325, "Rm1St7Dr3Cmd"=326, "Rm1St8Dr3Cmd"=327, "fwRmTempSP"=328, "fwRmHumSP"=329, "fwCoolTempSP"=330, "fwDehumTempSP"=331, "fwRmRun"=332, "fwRmOk"=333, "fwTesting"=334, "fwRmDryP"=335, "fwRmDryI"=336, "fwRmHumP"=337, "fwRmHumI"=338, "fwRmHeatP"=339, "fwRmHeatI"=340, "fwCoolTempP"=341, "fwCoolTempI"=342, "fwDehumTempP"=343, "fwDehumTempI"=344, "fwGndLeak1"=345, "fwGndLeak2"=346, "fwGndLeak3"=347, "fwGndLeak4"=348, "fwGndLeak5"=349, "fwGndLeak6"=350, "fwGndLeak7"=351, "fwGndLeak8"=352, "Rm1OpenerCmd"=353] ("Ring")
            w300 = T27 305 items=["fwS1Volt1"=0, "fwS1Volt2"=1, "fwS2Volt1"=2, "fwS2Volt2"=3, "fwS3Volt1"=4, "fwS3Volt2"=5, "fwS4Volt1"=6, "fwS4Volt2"=7, "fwS5Volt1"=8, "fwS5Volt2"=9, "fwS6Volt1"=10, "fwS6Volt2 "=11, "fwS7Volt1"=12, "fwS7Volt2"=13, "fwS8Volt1"=14, "fwS8Volt2"=15, "fwRoomHum"=16, "fwRoomTemp"=17, "fwAISpare1"=18, "fwAISpare2"=19, "fwSuppTemp"=20, "fwCoolTemp"=21, "fwDehumTemp"=22, "fwUnused"=23, "Bool Inputs"=24, "gwVoltRate1"=256, "gwVoltRate2"=257, "gwVoltRate3"=258, "gwVoltRate4"=259, "gwVoltRate5"=260, "gwVoltRate6"=261, "gwVoltRate7"=262, "gwVoltRate8"=263, "gwVoltWindow5/1"=264, "gwVoltWindow6/2"=265, "gwVoltWindow7/3"=266, "gwVoltWindow8/4"=267, "fwVoltSet1"=272, "fwVoltSet2"=273, "fwVoltSet3"=274, "fwVoltSet4"=275, "fwVoltSet5"=276, "fwVoltSet6"=277, "fwVoltSet7"=278, "fwVoltSet8"=279, "fwVoltRng1"=280, "fwVoltRng2"=281, "fwVoltRng3"=282, "fwVoltRng4"=283, "fwVoltRng5"=284, "fwVoltRng6"=285, "fwVoltRng7"=286, "fwVoltRng8"=287, "fwVoltPol1"=296, "fwVoltPol2"=297, "fwVoltPol3"=298, "fwVoltPol4"=299, "fwVoltPol5"=300, "fwVoltPol6"=301, "fwVoltPol7"=302, "fwVoltPol8"=303, "Rm1St1Dr1Cmd"=304, "Rm1St2Dr1Cmd"=305, "Rm1St3Dr1Cmd"=306, "Rm1St4Dr1Cmd"=307, "Rm1St5Dr1Cmd"=308, "Rm1St6Dr1Cmd"=309, "Rm1St7Dr1Cmd"=310, "Rm1St8Dr1Cmd"=311, "Rm1St1Dr2Cmd"=312, "Rm1St2Dr2Cmd"=313, "Rm1St3Dr2Cmd"=314, "Rm1St4Dr2Cmd"=315, "Rm1St5Dr2Cmd"=316, "Rm1St6Dr2Cmd"=317, "Rm1St7Dr2Cmd"=318, "Rm1St8Dr2Cmd"=319, "Rm1St1Dr3Cmd"=320, "Rm1St2Dr3Cmd"=321, "Rm1St3Dr3Cmd"=322, "Rm1St4Dr3Cmd"=323, "Rm1St5Dr3Cmd"=324, "Rm1St6Dr3Cmd"=325, "Rm1St7Dr3Cmd"=326, "Rm1St8Dr3Cmd"=327, "fwRmTempSP"=328, "fwRmHumSP"=329, "fwCoolTempSP"=330, "fwDehumTempSP"=331, "fwRmRun"=332, "fwRmOk"=333, "fwTesting"=334, "fwRmDryP"=335, "fwRmDryI"=336, "fwRmHumP"=337, "fwRmHumI"=338, "fwRmHeatP"=339, "fwRmHeatI"=340, "fwCoolTempP"=341, "fwCoolTempI"=342, "fwDehumTempP"=343, "fwDehumTempI"=344, "fwGndLeak1"=345, "fwGndLeak2"=346, "fwGndLeak3"=347, "fwGndLeak4"=348, "fwGndLeak5"=349, "fwGndLeak6"=350, "fwGndLeak7"=351, "fwGndLeak8"=352, "Rm1OpenerCmd"=353] ("Ring")
            n90 = event-data() -> ()  [unwired: 1 in, 6 out]
            n91 = local read "Door Settings"() -> (w288:T11)
            n92 = Unbundle By Name(w288) -> ("Station 2.Slide"=w293:T13, "Station 2.Cab"=w294:T13, "Station 2.Freezer"=w295:T13)
            n93 = call-dynamic "Write Single Holding Register.vi"("error in"=w292, "register to write"=w295, "address"=w300, "Modbus master in"=w287) -> ("error out"=w291:errorcluster, "Modbus master out"=w297:refnum<class "Modbus Master.lvclass">)  [unwired: 6 in]
            n94 = call-dynamic "Write Single Holding Register.vi"("error in"=w291, "register to write"=w294, "address"=w299, "Modbus master in"=w297) -> ("error out"=w290:errorcluster, "Modbus master out"=w296:refnum<class "Modbus Master.lvclass">)  [unwired: 6 in]
            n95 = call-dynamic "Write Single Holding Register.vi"("error in"=w290, "register to write"=w293, "address"=w298, "Modbus master in"=w296) -> ("error out"=w289:errorcluster)  [unwired: 6 in, 1 out]
          }
          event "Station 3 CMD": Value Change {
            w306 = T27 322 items=["fwS1Volt1"=0, "fwS1Volt2"=1, "fwS2Volt1"=2, "fwS2Volt2"=3, "fwS3Volt1"=4, "fwS3Volt2"=5, "fwS4Volt1"=6, "fwS4Volt2"=7, "fwS5Volt1"=8, "fwS5Volt2"=9, "fwS6Volt1"=10, "fwS6Volt2 "=11, "fwS7Volt1"=12, "fwS7Volt2"=13, "fwS8Volt1"=14, "fwS8Volt2"=15, "fwRoomHum"=16, "fwRoomTemp"=17, "fwAISpare1"=18, "fwAISpare2"=19, "fwSuppTemp"=20, "fwCoolTemp"=21, "fwDehumTemp"=22, "fwUnused"=23, "Bool Inputs"=24, "gwVoltRate1"=256, "gwVoltRate2"=257, "gwVoltRate3"=258, "gwVoltRate4"=259, "gwVoltRate5"=260, "gwVoltRate6"=261, "gwVoltRate7"=262, "gwVoltRate8"=263, "gwVoltWindow5/1"=264, "gwVoltWindow6/2"=265, "gwVoltWindow7/3"=266, "gwVoltWindow8/4"=267, "fwVoltSet1"=272, "fwVoltSet2"=273, "fwVoltSet3"=274, "fwVoltSet4"=275, "fwVoltSet5"=276, "fwVoltSet6"=277, "fwVoltSet7"=278, "fwVoltSet8"=279, "fwVoltRng1"=280, "fwVoltRng2"=281, "fwVoltRng3"=282, "fwVoltRng4"=283, "fwVoltRng5"=284, "fwVoltRng6"=285, "fwVoltRng7"=286, "fwVoltRng8"=287, "fwVoltPol1"=296, "fwVoltPol2"=297, "fwVoltPol3"=298, "fwVoltPol4"=299, "fwVoltPol5"=300, "fwVoltPol6"=301, "fwVoltPol7"=302, "fwVoltPol8"=303, "Rm1St1Dr1Cmd"=304, "Rm1St2Dr1Cmd"=305, "Rm1St3Dr1Cmd"=306, "Rm1St4Dr1Cmd"=307, "Rm1St5Dr1Cmd"=308, "Rm1St6Dr1Cmd"=309, "Rm1St7Dr1Cmd"=310, "Rm1St8Dr1Cmd"=311, "Rm1St1Dr2Cmd"=312, "Rm1St2Dr2Cmd"=313, "Rm1St3Dr2Cmd"=314, "Rm1St4Dr2Cmd"=315, "Rm1St5Dr2Cmd"=316, "Rm1St6Dr2Cmd"=317, "Rm1St7Dr2Cmd"=318, "Rm1St8Dr2Cmd"=319, "Rm1St1Dr3Cmd"=320, "Rm1St2Dr3Cmd"=321, "Rm1St3Dr3Cmd"=322, "Rm1St4Dr3Cmd"=323, "Rm1St5Dr3Cmd"=324, "Rm1St6Dr3Cmd"=325, "Rm1St7Dr3Cmd"=326, "Rm1St8Dr3Cmd"=327, "fwRmTempSP"=328, "fwRmHumSP"=329, "fwCoolTempSP"=330, "fwDehumTempSP"=331, "fwRmRun"=332, "fwRmOk"=333, "fwTesting"=334, "fwRmDryP"=335, "fwRmDryI"=336, "fwRmHumP"=337, "fwRmHumI"=338, "fwRmHeatP"=339, "fwRmHeatI"=340, "fwCoolTempP"=341, "fwCoolTempI"=342, "fwDehumTempP"=343, "fwDehumTempI"=344, "fwGndLeak1"=345, "fwGndLeak2"=346, "fwGndLeak3"=347, "fwGndLeak4"=348, "fwGndLeak5"=349, "fwGndLeak6"=350, "fwGndLeak7"=351, "fwGndLeak8"=352, "Rm1OpenerCmd"=353] ("Ring")
            w307 = T27 314 items=["fwS1Volt1"=0, "fwS1Volt2"=1, "fwS2Volt1"=2, "fwS2Volt2"=3, "fwS3Volt1"=4, "fwS3Volt2"=5, "fwS4Volt1"=6, "fwS4Volt2"=7, "fwS5Volt1"=8, "fwS5Volt2"=9, "fwS6Volt1"=10, "fwS6Volt2 "=11, "fwS7Volt1"=12, "fwS7Volt2"=13, "fwS8Volt1"=14, "fwS8Volt2"=15, "fwRoomHum"=16, "fwRoomTemp"=17, "fwAISpare1"=18, "fwAISpare2"=19, "fwSuppTemp"=20, "fwCoolTemp"=21, "fwDehumTemp"=22, "fwUnused"=23, "Bool Inputs"=24, "gwVoltRate1"=256, "gwVoltRate2"=257, "gwVoltRate3"=258, "gwVoltRate4"=259, "gwVoltRate5"=260, "gwVoltRate6"=261, "gwVoltRate7"=262, "gwVoltRate8"=263, "gwVoltWindow5/1"=264, "gwVoltWindow6/2"=265, "gwVoltWindow7/3"=266, "gwVoltWindow8/4"=267, "fwVoltSet1"=272, "fwVoltSet2"=273, "fwVoltSet3"=274, "fwVoltSet4"=275, "fwVoltSet5"=276, "fwVoltSet6"=277, "fwVoltSet7"=278, "fwVoltSet8"=279, "fwVoltRng1"=280, "fwVoltRng2"=281, "fwVoltRng3"=282, "fwVoltRng4"=283, "fwVoltRng5"=284, "fwVoltRng6"=285, "fwVoltRng7"=286, "fwVoltRng8"=287, "fwVoltPol1"=296, "fwVoltPol2"=297, "fwVoltPol3"=298, "fwVoltPol4"=299, "fwVoltPol5"=300, "fwVoltPol6"=301, "fwVoltPol7"=302, "fwVoltPol8"=303, "Rm1St1Dr1Cmd"=304, "Rm1St2Dr1Cmd"=305, "Rm1St3Dr1Cmd"=306, "Rm1St4Dr1Cmd"=307, "Rm1St5Dr1Cmd"=308, "Rm1St6Dr1Cmd"=309, "Rm1St7Dr1Cmd"=310, "Rm1St8Dr1Cmd"=311, "Rm1St1Dr2Cmd"=312, "Rm1St2Dr2Cmd"=313, "Rm1St3Dr2Cmd"=314, "Rm1St4Dr2Cmd"=315, "Rm1St5Dr2Cmd"=316, "Rm1St6Dr2Cmd"=317, "Rm1St7Dr2Cmd"=318, "Rm1St8Dr2Cmd"=319, "Rm1St1Dr3Cmd"=320, "Rm1St2Dr3Cmd"=321, "Rm1St3Dr3Cmd"=322, "Rm1St4Dr3Cmd"=323, "Rm1St5Dr3Cmd"=324, "Rm1St6Dr3Cmd"=325, "Rm1St7Dr3Cmd"=326, "Rm1St8Dr3Cmd"=327, "fwRmTempSP"=328, "fwRmHumSP"=329, "fwCoolTempSP"=330, "fwDehumTempSP"=331, "fwRmRun"=332, "fwRmOk"=333, "fwTesting"=334, "fwRmDryP"=335, "fwRmDryI"=336, "fwRmHumP"=337, "fwRmHumI"=338, "fwRmHeatP"=339, "fwRmHeatI"=340, "fwCoolTempP"=341, "fwCoolTempI"=342, "fwDehumTempP"=343, "fwDehumTempI"=344, "fwGndLeak1"=345, "fwGndLeak2"=346, "fwGndLeak3"=347, "fwGndLeak4"=348, "fwGndLeak5"=349, "fwGndLeak6"=350, "fwGndLeak7"=351, "fwGndLeak8"=352, "Rm1OpenerCmd"=353] ("Ring")
            w316 = T27 306 items=["fwS1Volt1"=0, "fwS1Volt2"=1, "fwS2Volt1"=2, "fwS2Volt2"=3, "fwS3Volt1"=4, "fwS3Volt2"=5, "fwS4Volt1"=6, "fwS4Volt2"=7, "fwS5Volt1"=8, "fwS5Volt2"=9, "fwS6Volt1"=10, "fwS6Volt2 "=11, "fwS7Volt1"=12, "fwS7Volt2"=13, "fwS8Volt1"=14, "fwS8Volt2"=15, "fwRoomHum"=16, "fwRoomTemp"=17, "fwAISpare1"=18, "fwAISpare2"=19, "fwSuppTemp"=20, "fwCoolTemp"=21, "fwDehumTemp"=22, "fwUnused"=23, "Bool Inputs"=24, "gwVoltRate1"=256, "gwVoltRate2"=257, "gwVoltRate3"=258, "gwVoltRate4"=259, "gwVoltRate5"=260, "gwVoltRate6"=261, "gwVoltRate7"=262, "gwVoltRate8"=263, "gwVoltWindow5/1"=264, "gwVoltWindow6/2"=265, "gwVoltWindow7/3"=266, "gwVoltWindow8/4"=267, "fwVoltSet1"=272, "fwVoltSet2"=273, "fwVoltSet3"=274, "fwVoltSet4"=275, "fwVoltSet5"=276, "fwVoltSet6"=277, "fwVoltSet7"=278, "fwVoltSet8"=279, "fwVoltRng1"=280, "fwVoltRng2"=281, "fwVoltRng3"=282, "fwVoltRng4"=283, "fwVoltRng5"=284, "fwVoltRng6"=285, "fwVoltRng7"=286, "fwVoltRng8"=287, "fwVoltPol1"=296, "fwVoltPol2"=297, "fwVoltPol3"=298, "fwVoltPol4"=299, "fwVoltPol5"=300, "fwVoltPol6"=301, "fwVoltPol7"=302, "fwVoltPol8"=303, "Rm1St1Dr1Cmd"=304, "Rm1St2Dr1Cmd"=305, "Rm1St3Dr1Cmd"=306, "Rm1St4Dr1Cmd"=307, "Rm1St5Dr1Cmd"=308, "Rm1St6Dr1Cmd"=309, "Rm1St7Dr1Cmd"=310, "Rm1St8Dr1Cmd"=311, "Rm1St1Dr2Cmd"=312, "Rm1St2Dr2Cmd"=313, "Rm1St3Dr2Cmd"=314, "Rm1St4Dr2Cmd"=315, "Rm1St5Dr2Cmd"=316, "Rm1St6Dr2Cmd"=317, "Rm1St7Dr2Cmd"=318, "Rm1St8Dr2Cmd"=319, "Rm1St1Dr3Cmd"=320, "Rm1St2Dr3Cmd"=321, "Rm1St3Dr3Cmd"=322, "Rm1St4Dr3Cmd"=323, "Rm1St5Dr3Cmd"=324, "Rm1St6Dr3Cmd"=325, "Rm1St7Dr3Cmd"=326, "Rm1St8Dr3Cmd"=327, "fwRmTempSP"=328, "fwRmHumSP"=329, "fwCoolTempSP"=330, "fwDehumTempSP"=331, "fwRmRun"=332, "fwRmOk"=333, "fwTesting"=334, "fwRmDryP"=335, "fwRmDryI"=336, "fwRmHumP"=337, "fwRmHumI"=338, "fwRmHeatP"=339, "fwRmHeatI"=340, "fwCoolTempP"=341, "fwCoolTempI"=342, "fwDehumTempP"=343, "fwDehumTempI"=344, "fwGndLeak1"=345, "fwGndLeak2"=346, "fwGndLeak3"=347, "fwGndLeak4"=348, "fwGndLeak5"=349, "fwGndLeak6"=350, "fwGndLeak7"=351, "fwGndLeak8"=352, "Rm1OpenerCmd"=353] ("Ring")
            n96 = event-data() -> ()  [unwired: 1 in, 6 out]
            n97 = local read "Door Settings"() -> (w311:T11)
            n98 = Unbundle By Name(w311) -> ("Station 3.Slide"=w312:T13, "Station 3.Cab"=w313:T13, "Station 3.Freezer"=w314:T13)
            n99 = call-dynamic "Write Single Holding Register.vi"("error in"=w310, "register to write"=w314, "address"=w316, "Modbus master in"=w308) -> ("error out"=w304:errorcluster, "Modbus master out"=w315:refnum<class "Modbus Master.lvclass">)  [unwired: 6 in]
            n100 = call-dynamic "Write Single Holding Register.vi"("error in"=w304, "register to write"=w313, "address"=w307, "Modbus master in"=w315) -> ("error out"=w303:errorcluster, "Modbus master out"=w305:refnum<class "Modbus Master.lvclass">)  [unwired: 6 in]
            n101 = call-dynamic "Write Single Holding Register.vi"("error in"=w303, "register to write"=w312, "address"=w306, "Modbus master in"=w305) -> ("error out"=w309:errorcluster)  [unwired: 6 in, 1 out]
          }
          event Value Change {
            w323 = T27 345 items=["fwS1Volt1"=0, "fwS1Volt2"=1, "fwS2Volt1"=2, "fwS2Volt2"=3, "fwS3Volt1"=4, "fwS3Volt2"=5, "fwS4Volt1"=6, "fwS4Volt2"=7, "fwS5Volt1"=8, "fwS5Volt2"=9, "fwS6Volt1"=10, "fwS6Volt2 "=11, "fwS7Volt1"=12, "fwS7Volt2"=13, "fwS8Volt1"=14, "fwS8Volt2"=15, "fwRoomHum"=16, "fwRoomTemp"=17, "fwAISpare1"=18, "fwAISpare2"=19, "fwSuppTemp"=20, "fwCoolTemp"=21, "fwDehumTemp"=22, "fwUnused"=23, "Bool Inputs"=24, "gwVoltRate1"=256, "gwVoltRate2"=257, "gwVoltRate3"=258, "gwVoltRate4"=259, "gwVoltRate5"=260, "gwVoltRate6"=261, "gwVoltRate7"=262, "gwVoltRate8"=263, "gwVoltWindow5/1"=264, "gwVoltWindow6/2"=265, "gwVoltWindow7/3"=266, "gwVoltWindow8/4"=267, "fwVoltSet1"=272, "fwVoltSet2"=273, "fwVoltSet3"=274, "fwVoltSet4"=275, "fwVoltSet5"=276, "fwVoltSet6"=277, "fwVoltSet7"=278, "fwVoltSet8"=279, "fwVoltRng1"=280, "fwVoltRng2"=281, "fwVoltRng3"=282, "fwVoltRng4"=283, "fwVoltRng5"=284, "fwVoltRng6"=285, "fwVoltRng7"=286, "fwVoltRng8"=287, "fwVoltPol1"=296, "fwVoltPol2"=297, "fwVoltPol3"=298, "fwVoltPol4"=299, "fwVoltPol5"=300, "fwVoltPol6"=301, "fwVoltPol7"=302, "fwVoltPol8"=303, "Rm1St1Dr1Cmd"=304, "Rm1St2Dr1Cmd"=305, "Rm1St3Dr1Cmd"=306, "Rm1St4Dr1Cmd"=307, "Rm1St5Dr1Cmd"=308, "Rm1St6Dr1Cmd"=309, "Rm1St7Dr1Cmd"=310, "Rm1St8Dr1Cmd"=311, "Rm1St1Dr2Cmd"=312, "Rm1St2Dr2Cmd"=313, "Rm1St3Dr2Cmd"=314, "Rm1St4Dr2Cmd"=315, "Rm1St5Dr2Cmd"=316, "Rm1St6Dr2Cmd"=317, "Rm1St7Dr2Cmd"=318, "Rm1St8Dr2Cmd"=319, "Rm1St1Dr3Cmd"=320, "Rm1St2Dr3Cmd"=321, "Rm1St3Dr3Cmd"=322, "Rm1St4Dr3Cmd"=323, "Rm1St5Dr3Cmd"=324, "Rm1St6Dr3Cmd"=325, "Rm1St7Dr3Cmd"=326, "Rm1St8Dr3Cmd"=327, "fwRmTempSP"=328, "fwRmHumSP"=329, "fwCoolTempSP"=330, "fwDehumTempSP"=331, "fwRmRun"=332, "fwRmOk"=333, "fwTesting"=334, "fwRmDryP"=335, "fwRmDryI"=336, "fwRmHumP"=337, "fwRmHumI"=338, "fwRmHeatP"=339, "fwRmHeatI"=340, "fwCoolTempP"=341, "fwCoolTempI"=342, "fwDehumTempP"=343, "fwDehumTempI"=344, "fwGndLeak1"=345, "fwGndLeak2"=346, "fwGndLeak3"=347, "fwGndLeak4"=348, "fwGndLeak5"=349, "fwGndLeak6"=350, "fwGndLeak7"=351, "fwGndLeak8"=352, "Rm1OpenerCmd"=353] ("Ring")
            n102 = event-data() -> ("NewVal"=w320:T8)  [unwired: 1 in, 5 out]
            n103 = call-dynamic "Write Single Holding Register.vi"("error in"=w322, "register to write"=w320, "address"=w323, "Modbus master in"=w319) -> ("error out"=w321:errorcluster)  [unwired: 6 in, 1 out]
          }
          event Value Change {
            w330 = T27 346 items=["fwS1Volt1"=0, "fwS1Volt2"=1, "fwS2Volt1"=2, "fwS2Volt2"=3, "fwS3Volt1"=4, "fwS3Volt2"=5, "fwS4Volt1"=6, "fwS4Volt2"=7, "fwS5Volt1"=8, "fwS5Volt2"=9, "fwS6Volt1"=10, "fwS6Volt2 "=11, "fwS7Volt1"=12, "fwS7Volt2"=13, "fwS8Volt1"=14, "fwS8Volt2"=15, "fwRoomHum"=16, "fwRoomTemp"=17, "fwAISpare1"=18, "fwAISpare2"=19, "fwSuppTemp"=20, "fwCoolTemp"=21, "fwDehumTemp"=22, "fwUnused"=23, "Bool Inputs"=24, "gwVoltRate1"=256, "gwVoltRate2"=257, "gwVoltRate3"=258, "gwVoltRate4"=259, "gwVoltRate5"=260, "gwVoltRate6"=261, "gwVoltRate7"=262, "gwVoltRate8"=263, "gwVoltWindow5/1"=264, "gwVoltWindow6/2"=265, "gwVoltWindow7/3"=266, "gwVoltWindow8/4"=267, "fwVoltSet1"=272, "fwVoltSet2"=273, "fwVoltSet3"=274, "fwVoltSet4"=275, "fwVoltSet5"=276, "fwVoltSet6"=277, "fwVoltSet7"=278, "fwVoltSet8"=279, "fwVoltRng1"=280, "fwVoltRng2"=281, "fwVoltRng3"=282, "fwVoltRng4"=283, "fwVoltRng5"=284, "fwVoltRng6"=285, "fwVoltRng7"=286, "fwVoltRng8"=287, "fwVoltPol1"=296, "fwVoltPol2"=297, "fwVoltPol3"=298, "fwVoltPol4"=299, "fwVoltPol5"=300, "fwVoltPol6"=301, "fwVoltPol7"=302, "fwVoltPol8"=303, "Rm1St1Dr1Cmd"=304, "Rm1St2Dr1Cmd"=305, "Rm1St3Dr1Cmd"=306, "Rm1St4Dr1Cmd"=307, "Rm1St5Dr1Cmd"=308, "Rm1St6Dr1Cmd"=309, "Rm1St7Dr1Cmd"=310, "Rm1St8Dr1Cmd"=311, "Rm1St1Dr2Cmd"=312, "Rm1St2Dr2Cmd"=313, "Rm1St3Dr2Cmd"=314, "Rm1St4Dr2Cmd"=315, "Rm1St5Dr2Cmd"=316, "Rm1St6Dr2Cmd"=317, "Rm1St7Dr2Cmd"=318, "Rm1St8Dr2Cmd"=319, "Rm1St1Dr3Cmd"=320, "Rm1St2Dr3Cmd"=321, "Rm1St3Dr3Cmd"=322, "Rm1St4Dr3Cmd"=323, "Rm1St5Dr3Cmd"=324, "Rm1St6Dr3Cmd"=325, "Rm1St7Dr3Cmd"=326, "Rm1St8Dr3Cmd"=327, "fwRmTempSP"=328, "fwRmHumSP"=329, "fwCoolTempSP"=330, "fwDehumTempSP"=331, "fwRmRun"=332, "fwRmOk"=333, "fwTesting"=334, "fwRmDryP"=335, "fwRmDryI"=336, "fwRmHumP"=337, "fwRmHumI"=338, "fwRmHeatP"=339, "fwRmHeatI"=340, "fwCoolTempP"=341, "fwCoolTempI"=342, "fwDehumTempP"=343, "fwDehumTempI"=344, "fwGndLeak1"=345, "fwGndLeak2"=346, "fwGndLeak3"=347, "fwGndLeak4"=348, "fwGndLeak5"=349, "fwGndLeak6"=350, "fwGndLeak7"=351, "fwGndLeak8"=352, "Rm1OpenerCmd"=353] ("Ring")
            n104 = event-data() -> ("NewVal"=w326:T8)  [unwired: 1 in, 5 out]
            n105 = call-dynamic "Write Single Holding Register.vi"("error in"=w329, "register to write"=w326, "address"=w330, "Modbus master in"=w327) -> ("error out"=w328:errorcluster)  [unwired: 6 in, 1 out]
          }
          event Value Change {
            w337 = T27 347 items=["fwS1Volt1"=0, "fwS1Volt2"=1, "fwS2Volt1"=2, "fwS2Volt2"=3, "fwS3Volt1"=4, "fwS3Volt2"=5, "fwS4Volt1"=6, "fwS4Volt2"=7, "fwS5Volt1"=8, "fwS5Volt2"=9, "fwS6Volt1"=10, "fwS6Volt2 "=11, "fwS7Volt1"=12, "fwS7Volt2"=13, "fwS8Volt1"=14, "fwS8Volt2"=15, "fwRoomHum"=16, "fwRoomTemp"=17, "fwAISpare1"=18, "fwAISpare2"=19, "fwSuppTemp"=20, "fwCoolTemp"=21, "fwDehumTemp"=22, "fwUnused"=23, "Bool Inputs"=24, "gwVoltRate1"=256, "gwVoltRate2"=257, "gwVoltRate3"=258, "gwVoltRate4"=259, "gwVoltRate5"=260, "gwVoltRate6"=261, "gwVoltRate7"=262, "gwVoltRate8"=263, "gwVoltWindow5/1"=264, "gwVoltWindow6/2"=265, "gwVoltWindow7/3"=266, "gwVoltWindow8/4"=267, "fwVoltSet1"=272, "fwVoltSet2"=273, "fwVoltSet3"=274, "fwVoltSet4"=275, "fwVoltSet5"=276, "fwVoltSet6"=277, "fwVoltSet7"=278, "fwVoltSet8"=279, "fwVoltRng1"=280, "fwVoltRng2"=281, "fwVoltRng3"=282, "fwVoltRng4"=283, "fwVoltRng5"=284, "fwVoltRng6"=285, "fwVoltRng7"=286, "fwVoltRng8"=287, "fwVoltPol1"=296, "fwVoltPol2"=297, "fwVoltPol3"=298, "fwVoltPol4"=299, "fwVoltPol5"=300, "fwVoltPol6"=301, "fwVoltPol7"=302, "fwVoltPol8"=303, "Rm1St1Dr1Cmd"=304, "Rm1St2Dr1Cmd"=305, "Rm1St3Dr1Cmd"=306, "Rm1St4Dr1Cmd"=307, "Rm1St5Dr1Cmd"=308, "Rm1St6Dr1Cmd"=309, "Rm1St7Dr1Cmd"=310, "Rm1St8Dr1Cmd"=311, "Rm1St1Dr2Cmd"=312, "Rm1St2Dr2Cmd"=313, "Rm1St3Dr2Cmd"=314, "Rm1St4Dr2Cmd"=315, "Rm1St5Dr2Cmd"=316, "Rm1St6Dr2Cmd"=317, "Rm1St7Dr2Cmd"=318, "Rm1St8Dr2Cmd"=319, "Rm1St1Dr3Cmd"=320, "Rm1St2Dr3Cmd"=321, "Rm1St3Dr3Cmd"=322, "Rm1St4Dr3Cmd"=323, "Rm1St5Dr3Cmd"=324, "Rm1St6Dr3Cmd"=325, "Rm1St7Dr3Cmd"=326, "Rm1St8Dr3Cmd"=327, "fwRmTempSP"=328, "fwRmHumSP"=329, "fwCoolTempSP"=330, "fwDehumTempSP"=331, "fwRmRun"=332, "fwRmOk"=333, "fwTesting"=334, "fwRmDryP"=335, "fwRmDryI"=336, "fwRmHumP"=337, "fwRmHumI"=338, "fwRmHeatP"=339, "fwRmHeatI"=340, "fwCoolTempP"=341, "fwCoolTempI"=342, "fwDehumTempP"=343, "fwDehumTempI"=344, "fwGndLeak1"=345, "fwGndLeak2"=346, "fwGndLeak3"=347, "fwGndLeak4"=348, "fwGndLeak5"=349, "fwGndLeak6"=350, "fwGndLeak7"=351, "fwGndLeak8"=352, "Rm1OpenerCmd"=353] ("Ring")
            n106 = event-data() -> ("NewVal"=w333:T8)  [unwired: 1 in, 5 out]
            n107 = call-dynamic "Write Single Holding Register.vi"("error in"=w336, "register to write"=w333, "address"=w337, "Modbus master in"=w334) -> ("error out"=w335:errorcluster)  [unwired: 6 in, 1 out]
          }
          event Value Change {
            w344 = T27 348 items=["fwS1Volt1"=0, "fwS1Volt2"=1, "fwS2Volt1"=2, "fwS2Volt2"=3, "fwS3Volt1"=4, "fwS3Volt2"=5, "fwS4Volt1"=6, "fwS4Volt2"=7, "fwS5Volt1"=8, "fwS5Volt2"=9, "fwS6Volt1"=10, "fwS6Volt2 "=11, "fwS7Volt1"=12, "fwS7Volt2"=13, "fwS8Volt1"=14, "fwS8Volt2"=15, "fwRoomHum"=16, "fwRoomTemp"=17, "fwAISpare1"=18, "fwAISpare2"=19, "fwSuppTemp"=20, "fwCoolTemp"=21, "fwDehumTemp"=22, "fwUnused"=23, "Bool Inputs"=24, "gwVoltRate1"=256, "gwVoltRate2"=257, "gwVoltRate3"=258, "gwVoltRate4"=259, "gwVoltRate5"=260, "gwVoltRate6"=261, "gwVoltRate7"=262, "gwVoltRate8"=263, "gwVoltWindow5/1"=264, "gwVoltWindow6/2"=265, "gwVoltWindow7/3"=266, "gwVoltWindow8/4"=267, "fwVoltSet1"=272, "fwVoltSet2"=273, "fwVoltSet3"=274, "fwVoltSet4"=275, "fwVoltSet5"=276, "fwVoltSet6"=277, "fwVoltSet7"=278, "fwVoltSet8"=279, "fwVoltRng1"=280, "fwVoltRng2"=281, "fwVoltRng3"=282, "fwVoltRng4"=283, "fwVoltRng5"=284, "fwVoltRng6"=285, "fwVoltRng7"=286, "fwVoltRng8"=287, "fwVoltPol1"=296, "fwVoltPol2"=297, "fwVoltPol3"=298, "fwVoltPol4"=299, "fwVoltPol5"=300, "fwVoltPol6"=301, "fwVoltPol7"=302, "fwVoltPol8"=303, "Rm1St1Dr1Cmd"=304, "Rm1St2Dr1Cmd"=305, "Rm1St3Dr1Cmd"=306, "Rm1St4Dr1Cmd"=307, "Rm1St5Dr1Cmd"=308, "Rm1St6Dr1Cmd"=309, "Rm1St7Dr1Cmd"=310, "Rm1St8Dr1Cmd"=311, "Rm1St1Dr2Cmd"=312, "Rm1St2Dr2Cmd"=313, "Rm1St3Dr2Cmd"=314, "Rm1St4Dr2Cmd"=315, "Rm1St5Dr2Cmd"=316, "Rm1St6Dr2Cmd"=317, "Rm1St7Dr2Cmd"=318, "Rm1St8Dr2Cmd"=319, "Rm1St1Dr3Cmd"=320, "Rm1St2Dr3Cmd"=321, "Rm1St3Dr3Cmd"=322, "Rm1St4Dr3Cmd"=323, "Rm1St5Dr3Cmd"=324, "Rm1St6Dr3Cmd"=325, "Rm1St7Dr3Cmd"=326, "Rm1St8Dr3Cmd"=327, "fwRmTempSP"=328, "fwRmHumSP"=329, "fwCoolTempSP"=330, "fwDehumTempSP"=331, "fwRmRun"=332, "fwRmOk"=333, "fwTesting"=334, "fwRmDryP"=335, "fwRmDryI"=336, "fwRmHumP"=337, "fwRmHumI"=338, "fwRmHeatP"=339, "fwRmHeatI"=340, "fwCoolTempP"=341, "fwCoolTempI"=342, "fwDehumTempP"=343, "fwDehumTempI"=344, "fwGndLeak1"=345, "fwGndLeak2"=346, "fwGndLeak3"=347, "fwGndLeak4"=348, "fwGndLeak5"=349, "fwGndLeak6"=350, "fwGndLeak7"=351, "fwGndLeak8"=352, "Rm1OpenerCmd"=353] ("Ring")
            n108 = event-data() -> ("NewVal"=w340:T8)  [unwired: 1 in, 5 out]
            n109 = call-dynamic "Write Single Holding Register.vi"("error in"=w343, "register to write"=w340, "address"=w344, "Modbus master in"=w341) -> ("error out"=w342:errorcluster)  [unwired: 6 in, 1 out]
          }
          event Value Change {
            w351 = T27 349 items=["fwS1Volt1"=0, "fwS1Volt2"=1, "fwS2Volt1"=2, "fwS2Volt2"=3, "fwS3Volt1"=4, "fwS3Volt2"=5, "fwS4Volt1"=6, "fwS4Volt2"=7, "fwS5Volt1"=8, "fwS5Volt2"=9, "fwS6Volt1"=10, "fwS6Volt2 "=11, "fwS7Volt1"=12, "fwS7Volt2"=13, "fwS8Volt1"=14, "fwS8Volt2"=15, "fwRoomHum"=16, "fwRoomTemp"=17, "fwAISpare1"=18, "fwAISpare2"=19, "fwSuppTemp"=20, "fwCoolTemp"=21, "fwDehumTemp"=22, "fwUnused"=23, "Bool Inputs"=24, "gwVoltRate1"=256, "gwVoltRate2"=257, "gwVoltRate3"=258, "gwVoltRate4"=259, "gwVoltRate5"=260, "gwVoltRate6"=261, "gwVoltRate7"=262, "gwVoltRate8"=263, "gwVoltWindow5/1"=264, "gwVoltWindow6/2"=265, "gwVoltWindow7/3"=266, "gwVoltWindow8/4"=267, "fwVoltSet1"=272, "fwVoltSet2"=273, "fwVoltSet3"=274, "fwVoltSet4"=275, "fwVoltSet5"=276, "fwVoltSet6"=277, "fwVoltSet7"=278, "fwVoltSet8"=279, "fwVoltRng1"=280, "fwVoltRng2"=281, "fwVoltRng3"=282, "fwVoltRng4"=283, "fwVoltRng5"=284, "fwVoltRng6"=285, "fwVoltRng7"=286, "fwVoltRng8"=287, "fwVoltPol1"=296, "fwVoltPol2"=297, "fwVoltPol3"=298, "fwVoltPol4"=299, "fwVoltPol5"=300, "fwVoltPol6"=301, "fwVoltPol7"=302, "fwVoltPol8"=303, "Rm1St1Dr1Cmd"=304, "Rm1St2Dr1Cmd"=305, "Rm1St3Dr1Cmd"=306, "Rm1St4Dr1Cmd"=307, "Rm1St5Dr1Cmd"=308, "Rm1St6Dr1Cmd"=309, "Rm1St7Dr1Cmd"=310, "Rm1St8Dr1Cmd"=311, "Rm1St1Dr2Cmd"=312, "Rm1St2Dr2Cmd"=313, "Rm1St3Dr2Cmd"=314, "Rm1St4Dr2Cmd"=315, "Rm1St5Dr2Cmd"=316, "Rm1St6Dr2Cmd"=317, "Rm1St7Dr2Cmd"=318, "Rm1St8Dr2Cmd"=319, "Rm1St1Dr3Cmd"=320, "Rm1St2Dr3Cmd"=321, "Rm1St3Dr3Cmd"=322, "Rm1St4Dr3Cmd"=323, "Rm1St5Dr3Cmd"=324, "Rm1St6Dr3Cmd"=325, "Rm1St7Dr3Cmd"=326, "Rm1St8Dr3Cmd"=327, "fwRmTempSP"=328, "fwRmHumSP"=329, "fwCoolTempSP"=330, "fwDehumTempSP"=331, "fwRmRun"=332, "fwRmOk"=333, "fwTesting"=334, "fwRmDryP"=335, "fwRmDryI"=336, "fwRmHumP"=337, "fwRmHumI"=338, "fwRmHeatP"=339, "fwRmHeatI"=340, "fwCoolTempP"=341, "fwCoolTempI"=342, "fwDehumTempP"=343, "fwDehumTempI"=344, "fwGndLeak1"=345, "fwGndLeak2"=346, "fwGndLeak3"=347, "fwGndLeak4"=348, "fwGndLeak5"=349, "fwGndLeak6"=350, "fwGndLeak7"=351, "fwGndLeak8"=352, "Rm1OpenerCmd"=353] ("Ring")
            n110 = event-data() -> ("NewVal"=w347:T8)  [unwired: 1 in, 5 out]
            n111 = call-dynamic "Write Single Holding Register.vi"("error in"=w350, "register to write"=w347, "address"=w351, "Modbus master in"=w348) -> ("error out"=w349:errorcluster)  [unwired: 6 in, 1 out]
          }
          event Value Change {
            w358 = T27 350 items=["fwS1Volt1"=0, "fwS1Volt2"=1, "fwS2Volt1"=2, "fwS2Volt2"=3, "fwS3Volt1"=4, "fwS3Volt2"=5, "fwS4Volt1"=6, "fwS4Volt2"=7, "fwS5Volt1"=8, "fwS5Volt2"=9, "fwS6Volt1"=10, "fwS6Volt2 "=11, "fwS7Volt1"=12, "fwS7Volt2"=13, "fwS8Volt1"=14, "fwS8Volt2"=15, "fwRoomHum"=16, "fwRoomTemp"=17, "fwAISpare1"=18, "fwAISpare2"=19, "fwSuppTemp"=20, "fwCoolTemp"=21, "fwDehumTemp"=22, "fwUnused"=23, "Bool Inputs"=24, "gwVoltRate1"=256, "gwVoltRate2"=257, "gwVoltRate3"=258, "gwVoltRate4"=259, "gwVoltRate5"=260, "gwVoltRate6"=261, "gwVoltRate7"=262, "gwVoltRate8"=263, "gwVoltWindow5/1"=264, "gwVoltWindow6/2"=265, "gwVoltWindow7/3"=266, "gwVoltWindow8/4"=267, "fwVoltSet1"=272, "fwVoltSet2"=273, "fwVoltSet3"=274, "fwVoltSet4"=275, "fwVoltSet5"=276, "fwVoltSet6"=277, "fwVoltSet7"=278, "fwVoltSet8"=279, "fwVoltRng1"=280, "fwVoltRng2"=281, "fwVoltRng3"=282, "fwVoltRng4"=283, "fwVoltRng5"=284, "fwVoltRng6"=285, "fwVoltRng7"=286, "fwVoltRng8"=287, "fwVoltPol1"=296, "fwVoltPol2"=297, "fwVoltPol3"=298, "fwVoltPol4"=299, "fwVoltPol5"=300, "fwVoltPol6"=301, "fwVoltPol7"=302, "fwVoltPol8"=303, "Rm1St1Dr1Cmd"=304, "Rm1St2Dr1Cmd"=305, "Rm1St3Dr1Cmd"=306, "Rm1St4Dr1Cmd"=307, "Rm1St5Dr1Cmd"=308, "Rm1St6Dr1Cmd"=309, "Rm1St7Dr1Cmd"=310, "Rm1St8Dr1Cmd"=311, "Rm1St1Dr2Cmd"=312, "Rm1St2Dr2Cmd"=313, "Rm1St3Dr2Cmd"=314, "Rm1St4Dr2Cmd"=315, "Rm1St5Dr2Cmd"=316, "Rm1St6Dr2Cmd"=317, "Rm1St7Dr2Cmd"=318, "Rm1St8Dr2Cmd"=319, "Rm1St1Dr3Cmd"=320, "Rm1St2Dr3Cmd"=321, "Rm1St3Dr3Cmd"=322, "Rm1St4Dr3Cmd"=323, "Rm1St5Dr3Cmd"=324, "Rm1St6Dr3Cmd"=325, "Rm1St7Dr3Cmd"=326, "Rm1St8Dr3Cmd"=327, "fwRmTempSP"=328, "fwRmHumSP"=329, "fwCoolTempSP"=330, "fwDehumTempSP"=331, "fwRmRun"=332, "fwRmOk"=333, "fwTesting"=334, "fwRmDryP"=335, "fwRmDryI"=336, "fwRmHumP"=337, "fwRmHumI"=338, "fwRmHeatP"=339, "fwRmHeatI"=340, "fwCoolTempP"=341, "fwCoolTempI"=342, "fwDehumTempP"=343, "fwDehumTempI"=344, "fwGndLeak1"=345, "fwGndLeak2"=346, "fwGndLeak3"=347, "fwGndLeak4"=348, "fwGndLeak5"=349, "fwGndLeak6"=350, "fwGndLeak7"=351, "fwGndLeak8"=352, "Rm1OpenerCmd"=353] ("Ring")
            n112 = event-data() -> ("NewVal"=w354:T8)  [unwired: 1 in, 5 out]
            n113 = call-dynamic "Write Single Holding Register.vi"("error in"=w357, "register to write"=w354, "address"=w358, "Modbus master in"=w355) -> ("error out"=w356:errorcluster)  [unwired: 6 in, 1 out]
          }
          event Value Change {
            w367 = T27 351 items=["fwS1Volt1"=0, "fwS1Volt2"=1, "fwS2Volt1"=2, "fwS2Volt2"=3, "fwS3Volt1"=4, "fwS3Volt2"=5, "fwS4Volt1"=6, "fwS4Volt2"=7, "fwS5Volt1"=8, "fwS5Volt2"=9, "fwS6Volt1"=10, "fwS6Volt2 "=11, "fwS7Volt1"=12, "fwS7Volt2"=13, "fwS8Volt1"=14, "fwS8Volt2"=15, "fwRoomHum"=16, "fwRoomTemp"=17, "fwAISpare1"=18, "fwAISpare2"=19, "fwSuppTemp"=20, "fwCoolTemp"=21, "fwDehumTemp"=22, "fwUnused"=23, "Bool Inputs"=24, "gwVoltRate1"=256, "gwVoltRate2"=257, "gwVoltRate3"=258, "gwVoltRate4"=259, "gwVoltRate5"=260, "gwVoltRate6"=261, "gwVoltRate7"=262, "gwVoltRate8"=263, "gwVoltWindow5/1"=264, "gwVoltWindow6/2"=265, "gwVoltWindow7/3"=266, "gwVoltWindow8/4"=267, "fwVoltSet1"=272, "fwVoltSet2"=273, "fwVoltSet3"=274, "fwVoltSet4"=275, "fwVoltSet5"=276, "fwVoltSet6"=277, "fwVoltSet7"=278, "fwVoltSet8"=279, "fwVoltRng1"=280, "fwVoltRng2"=281, "fwVoltRng3"=282, "fwVoltRng4"=283, "fwVoltRng5"=284, "fwVoltRng6"=285, "fwVoltRng7"=286, "fwVoltRng8"=287, "fwVoltPol1"=296, "fwVoltPol2"=297, "fwVoltPol3"=298, "fwVoltPol4"=299, "fwVoltPol5"=300, "fwVoltPol6"=301, "fwVoltPol7"=302, "fwVoltPol8"=303, "Rm1St1Dr1Cmd"=304, "Rm1St2Dr1Cmd"=305, "Rm1St3Dr1Cmd"=306, "Rm1St4Dr1Cmd"=307, "Rm1St5Dr1Cmd"=308, "Rm1St6Dr1Cmd"=309, "Rm1St7Dr1Cmd"=310, "Rm1St8Dr1Cmd"=311, "Rm1St1Dr2Cmd"=312, "Rm1St2Dr2Cmd"=313, "Rm1St3Dr2Cmd"=314, "Rm1St4Dr2Cmd"=315, "Rm1St5Dr2Cmd"=316, "Rm1St6Dr2Cmd"=317, "Rm1St7Dr2Cmd"=318, "Rm1St8Dr2Cmd"=319, "Rm1St1Dr3Cmd"=320, "Rm1St2Dr3Cmd"=321, "Rm1St3Dr3Cmd"=322, "Rm1St4Dr3Cmd"=323, "Rm1St5Dr3Cmd"=324, "Rm1St6Dr3Cmd"=325, "Rm1St7Dr3Cmd"=326, "Rm1St8Dr3Cmd"=327, "fwRmTempSP"=328, "fwRmHumSP"=329, "fwCoolTempSP"=330, "fwDehumTempSP"=331, "fwRmRun"=332, "fwRmOk"=333, "fwTesting"=334, "fwRmDryP"=335, "fwRmDryI"=336, "fwRmHumP"=337, "fwRmHumI"=338, "fwRmHeatP"=339, "fwRmHeatI"=340, "fwCoolTempP"=341, "fwCoolTempI"=342, "fwDehumTempP"=343, "fwDehumTempI"=344, "fwGndLeak1"=345, "fwGndLeak2"=346, "fwGndLeak3"=347, "fwGndLeak4"=348, "fwGndLeak5"=349, "fwGndLeak6"=350, "fwGndLeak7"=351, "fwGndLeak8"=352, "Rm1OpenerCmd"=353] ("Ring")
            n114 = event-data() -> ("NewVal"=w363:T8)  [unwired: 1 in, 5 out]
            n115 = call-dynamic "Write Single Holding Register.vi"("error in"=w366, "register to write"=w363, "address"=w367, "Modbus master in"=w364) -> ("error out"=w365:errorcluster)  [unwired: 6 in, 1 out]
          }
          event Value Change {
            w372 = T27 352 items=["fwS1Volt1"=0, "fwS1Volt2"=1, "fwS2Volt1"=2, "fwS2Volt2"=3, "fwS3Volt1"=4, "fwS3Volt2"=5, "fwS4Volt1"=6, "fwS4Volt2"=7, "fwS5Volt1"=8, "fwS5Volt2"=9, "fwS6Volt1"=10, "fwS6Volt2 "=11, "fwS7Volt1"=12, "fwS7Volt2"=13, "fwS8Volt1"=14, "fwS8Volt2"=15, "fwRoomHum"=16, "fwRoomTemp"=17, "fwAISpare1"=18, "fwAISpare2"=19, "fwSuppTemp"=20, "fwCoolTemp"=21, "fwDehumTemp"=22, "fwUnused"=23, "Bool Inputs"=24, "gwVoltRate1"=256, "gwVoltRate2"=257, "gwVoltRate3"=258, "gwVoltRate4"=259, "gwVoltRate5"=260, "gwVoltRate6"=261, "gwVoltRate7"=262, "gwVoltRate8"=263, "gwVoltWindow5/1"=264, "gwVoltWindow6/2"=265, "gwVoltWindow7/3"=266, "gwVoltWindow8/4"=267, "fwVoltSet1"=272, "fwVoltSet2"=273, "fwVoltSet3"=274, "fwVoltSet4"=275, "fwVoltSet5"=276, "fwVoltSet6"=277, "fwVoltSet7"=278, "fwVoltSet8"=279, "fwVoltRng1"=280, "fwVoltRng2"=281, "fwVoltRng3"=282, "fwVoltRng4"=283, "fwVoltRng5"=284, "fwVoltRng6"=285, "fwVoltRng7"=286, "fwVoltRng8"=287, "fwVoltPol1"=296, "fwVoltPol2"=297, "fwVoltPol3"=298, "fwVoltPol4"=299, "fwVoltPol5"=300, "fwVoltPol6"=301, "fwVoltPol7"=302, "fwVoltPol8"=303, "Rm1St1Dr1Cmd"=304, "Rm1St2Dr1Cmd"=305, "Rm1St3Dr1Cmd"=306, "Rm1St4Dr1Cmd"=307, "Rm1St5Dr1Cmd"=308, "Rm1St6Dr1Cmd"=309, "Rm1St7Dr1Cmd"=310, "Rm1St8Dr1Cmd"=311, "Rm1St1Dr2Cmd"=312, "Rm1St2Dr2Cmd"=313, "Rm1St3Dr2Cmd"=314, "Rm1St4Dr2Cmd"=315, "Rm1St5Dr2Cmd"=316, "Rm1St6Dr2Cmd"=317, "Rm1St7Dr2Cmd"=318, "Rm1St8Dr2Cmd"=319, "Rm1St1Dr3Cmd"=320, "Rm1St2Dr3Cmd"=321, "Rm1St3Dr3Cmd"=322, "Rm1St4Dr3Cmd"=323, "Rm1St5Dr3Cmd"=324, "Rm1St6Dr3Cmd"=325, "Rm1St7Dr3Cmd"=326, "Rm1St8Dr3Cmd"=327, "fwRmTempSP"=328, "fwRmHumSP"=329, "fwCoolTempSP"=330, "fwDehumTempSP"=331, "fwRmRun"=332, "fwRmOk"=333, "fwTesting"=334, "fwRmDryP"=335, "fwRmDryI"=336, "fwRmHumP"=337, "fwRmHumI"=338, "fwRmHeatP"=339, "fwRmHeatI"=340, "fwCoolTempP"=341, "fwCoolTempI"=342, "fwDehumTempP"=343, "fwDehumTempI"=344, "fwGndLeak1"=345, "fwGndLeak2"=346, "fwGndLeak3"=347, "fwGndLeak4"=348, "fwGndLeak5"=349, "fwGndLeak6"=350, "fwGndLeak7"=351, "fwGndLeak8"=352, "Rm1OpenerCmd"=353] ("Ring")
            n116 = event-data() -> ("NewVal"=w368:T8)  [unwired: 1 in, 5 out]
            n117 = call-dynamic "Write Single Holding Register.vi"("error in"=w371, "register to write"=w368, "address"=w372, "Modbus master in"=w369) -> ("error out"=w370:errorcluster)  [unwired: 6 in, 1 out]
          }
          event Value Change {
            w379 = T27 296 items=["fwS1Volt1"=0, "fwS1Volt2"=1, "fwS2Volt1"=2, "fwS2Volt2"=3, "fwS3Volt1"=4, "fwS3Volt2"=5, "fwS4Volt1"=6, "fwS4Volt2"=7, "fwS5Volt1"=8, "fwS5Volt2"=9, "fwS6Volt1"=10, "fwS6Volt2 "=11, "fwS7Volt1"=12, "fwS7Volt2"=13, "fwS8Volt1"=14, "fwS8Volt2"=15, "fwRoomHum"=16, "fwRoomTemp"=17, "fwAISpare1"=18, "fwAISpare2"=19, "fwSuppTemp"=20, "fwCoolTemp"=21, "fwDehumTemp"=22, "fwUnused"=23, "Bool Inputs"=24, "gwVoltRate1"=256, "gwVoltRate2"=257, "gwVoltRate3"=258, "gwVoltRate4"=259, "gwVoltRate5"=260, "gwVoltRate6"=261, "gwVoltRate7"=262, "gwVoltRate8"=263, "gwVoltWindow5/1"=264, "gwVoltWindow6/2"=265, "gwVoltWindow7/3"=266, "gwVoltWindow8/4"=267, "fwVoltSet1"=272, "fwVoltSet2"=273, "fwVoltSet3"=274, "fwVoltSet4"=275, "fwVoltSet5"=276, "fwVoltSet6"=277, "fwVoltSet7"=278, "fwVoltSet8"=279, "fwVoltRng1"=280, "fwVoltRng2"=281, "fwVoltRng3"=282, "fwVoltRng4"=283, "fwVoltRng5"=284, "fwVoltRng6"=285, "fwVoltRng7"=286, "fwVoltRng8"=287, "fwVoltPol1"=296, "fwVoltPol2"=297, "fwVoltPol3"=298, "fwVoltPol4"=299, "fwVoltPol5"=300, "fwVoltPol6"=301, "fwVoltPol7"=302, "fwVoltPol8"=303, "Rm1St1Dr1Cmd"=304, "Rm1St2Dr1Cmd"=305, "Rm1St3Dr1Cmd"=306, "Rm1St4Dr1Cmd"=307, "Rm1St5Dr1Cmd"=308, "Rm1St6Dr1Cmd"=309, "Rm1St7Dr1Cmd"=310, "Rm1St8Dr1Cmd"=311, "Rm1St1Dr2Cmd"=312, "Rm1St2Dr2Cmd"=313, "Rm1St3Dr2Cmd"=314, "Rm1St4Dr2Cmd"=315, "Rm1St5Dr2Cmd"=316, "Rm1St6Dr2Cmd"=317, "Rm1St7Dr2Cmd"=318, "Rm1St8Dr2Cmd"=319, "Rm1St1Dr3Cmd"=320, "Rm1St2Dr3Cmd"=321, "Rm1St3Dr3Cmd"=322, "Rm1St4Dr3Cmd"=323, "Rm1St5Dr3Cmd"=324, "Rm1St6Dr3Cmd"=325, "Rm1St7Dr3Cmd"=326, "Rm1St8Dr3Cmd"=327, "fwRmTempSP"=328, "fwRmHumSP"=329, "fwCoolTempSP"=330, "fwDehumTempSP"=331, "fwRmRun"=332, "fwRmOk"=333, "fwTesting"=334, "fwRmDryP"=335, "fwRmDryI"=336, "fwRmHumP"=337, "fwRmHumI"=338, "fwRmHeatP"=339, "fwRmHeatI"=340, "fwCoolTempP"=341, "fwCoolTempI"=342, "fwDehumTempP"=343, "fwDehumTempI"=344, "fwGndLeak1"=345, "fwGndLeak2"=346, "fwGndLeak3"=347, "fwGndLeak4"=348, "fwGndLeak5"=349, "fwGndLeak6"=350, "fwGndLeak7"=351, "fwGndLeak8"=352, "Rm1OpenerCmd"=353] ("Ring")
            n118 = event-data() -> ("NewVal"=w376:T10)  [unwired: 1 in, 5 out]
            n119 = call-dynamic "Write Single Holding Register.vi"("error in"=w378, "register to write"=w376, "address"=w379, "Modbus master in"=w375) -> ("error out"=w377:errorcluster)  [unwired: 6 in, 1 out]
          }
          event Value Change {
            w386 = T27 297 items=["fwS1Volt1"=0, "fwS1Volt2"=1, "fwS2Volt1"=2, "fwS2Volt2"=3, "fwS3Volt1"=4, "fwS3Volt2"=5, "fwS4Volt1"=6, "fwS4Volt2"=7, "fwS5Volt1"=8, "fwS5Volt2"=9, "fwS6Volt1"=10, "fwS6Volt2 "=11, "fwS7Volt1"=12, "fwS7Volt2"=13, "fwS8Volt1"=14, "fwS8Volt2"=15, "fwRoomHum"=16, "fwRoomTemp"=17, "fwAISpare1"=18, "fwAISpare2"=19, "fwSuppTemp"=20, "fwCoolTemp"=21, "fwDehumTemp"=22, "fwUnused"=23, "Bool Inputs"=24, "gwVoltRate1"=256, "gwVoltRate2"=257, "gwVoltRate3"=258, "gwVoltRate4"=259, "gwVoltRate5"=260, "gwVoltRate6"=261, "gwVoltRate7"=262, "gwVoltRate8"=263, "gwVoltWindow5/1"=264, "gwVoltWindow6/2"=265, "gwVoltWindow7/3"=266, "gwVoltWindow8/4"=267, "fwVoltSet1"=272, "fwVoltSet2"=273, "fwVoltSet3"=274, "fwVoltSet4"=275, "fwVoltSet5"=276, "fwVoltSet6"=277, "fwVoltSet7"=278, "fwVoltSet8"=279, "fwVoltRng1"=280, "fwVoltRng2"=281, "fwVoltRng3"=282, "fwVoltRng4"=283, "fwVoltRng5"=284, "fwVoltRng6"=285, "fwVoltRng7"=286, "fwVoltRng8"=287, "fwVoltPol1"=296, "fwVoltPol2"=297, "fwVoltPol3"=298, "fwVoltPol4"=299, "fwVoltPol5"=300, "fwVoltPol6"=301, "fwVoltPol7"=302, "fwVoltPol8"=303, "Rm1St1Dr1Cmd"=304, "Rm1St2Dr1Cmd"=305, "Rm1St3Dr1Cmd"=306, "Rm1St4Dr1Cmd"=307, "Rm1St5Dr1Cmd"=308, "Rm1St6Dr1Cmd"=309, "Rm1St7Dr1Cmd"=310, "Rm1St8Dr1Cmd"=311, "Rm1St1Dr2Cmd"=312, "Rm1St2Dr2Cmd"=313, "Rm1St3Dr2Cmd"=314, "Rm1St4Dr2Cmd"=315, "Rm1St5Dr2Cmd"=316, "Rm1St6Dr2Cmd"=317, "Rm1St7Dr2Cmd"=318, "Rm1St8Dr2Cmd"=319, "Rm1St1Dr3Cmd"=320, "Rm1St2Dr3Cmd"=321, "Rm1St3Dr3Cmd"=322, "Rm1St4Dr3Cmd"=323, "Rm1St5Dr3Cmd"=324, "Rm1St6Dr3Cmd"=325, "Rm1St7Dr3Cmd"=326, "Rm1St8Dr3Cmd"=327, "fwRmTempSP"=328, "fwRmHumSP"=329, "fwCoolTempSP"=330, "fwDehumTempSP"=331, "fwRmRun"=332, "fwRmOk"=333, "fwTesting"=334, "fwRmDryP"=335, "fwRmDryI"=336, "fwRmHumP"=337, "fwRmHumI"=338, "fwRmHeatP"=339, "fwRmHeatI"=340, "fwCoolTempP"=341, "fwCoolTempI"=342, "fwDehumTempP"=343, "fwDehumTempI"=344, "fwGndLeak1"=345, "fwGndLeak2"=346, "fwGndLeak3"=347, "fwGndLeak4"=348, "fwGndLeak5"=349, "fwGndLeak6"=350, "fwGndLeak7"=351, "fwGndLeak8"=352, "Rm1OpenerCmd"=353] ("Ring")
            n120 = event-data() -> ("NewVal"=w383:T10)  [unwired: 1 in, 5 out]
            n121 = call-dynamic "Write Single Holding Register.vi"("error in"=w385, "register to write"=w383, "address"=w386, "Modbus master in"=w382) -> ("error out"=w384:errorcluster)  [unwired: 6 in, 1 out]
          }
          event Value Change {
            w393 = T27 298 items=["fwS1Volt1"=0, "fwS1Volt2"=1, "fwS2Volt1"=2, "fwS2Volt2"=3, "fwS3Volt1"=4, "fwS3Volt2"=5, "fwS4Volt1"=6, "fwS4Volt2"=7, "fwS5Volt1"=8, "fwS5Volt2"=9, "fwS6Volt1"=10, "fwS6Volt2 "=11, "fwS7Volt1"=12, "fwS7Volt2"=13, "fwS8Volt1"=14, "fwS8Volt2"=15, "fwRoomHum"=16, "fwRoomTemp"=17, "fwAISpare1"=18, "fwAISpare2"=19, "fwSuppTemp"=20, "fwCoolTemp"=21, "fwDehumTemp"=22, "fwUnused"=23, "Bool Inputs"=24, "gwVoltRate1"=256, "gwVoltRate2"=257, "gwVoltRate3"=258, "gwVoltRate4"=259, "gwVoltRate5"=260, "gwVoltRate6"=261, "gwVoltRate7"=262, "gwVoltRate8"=263, "gwVoltWindow5/1"=264, "gwVoltWindow6/2"=265, "gwVoltWindow7/3"=266, "gwVoltWindow8/4"=267, "fwVoltSet1"=272, "fwVoltSet2"=273, "fwVoltSet3"=274, "fwVoltSet4"=275, "fwVoltSet5"=276, "fwVoltSet6"=277, "fwVoltSet7"=278, "fwVoltSet8"=279, "fwVoltRng1"=280, "fwVoltRng2"=281, "fwVoltRng3"=282, "fwVoltRng4"=283, "fwVoltRng5"=284, "fwVoltRng6"=285, "fwVoltRng7"=286, "fwVoltRng8"=287, "fwVoltPol1"=296, "fwVoltPol2"=297, "fwVoltPol3"=298, "fwVoltPol4"=299, "fwVoltPol5"=300, "fwVoltPol6"=301, "fwVoltPol7"=302, "fwVoltPol8"=303, "Rm1St1Dr1Cmd"=304, "Rm1St2Dr1Cmd"=305, "Rm1St3Dr1Cmd"=306, "Rm1St4Dr1Cmd"=307, "Rm1St5Dr1Cmd"=308, "Rm1St6Dr1Cmd"=309, "Rm1St7Dr1Cmd"=310, "Rm1St8Dr1Cmd"=311, "Rm1St1Dr2Cmd"=312, "Rm1St2Dr2Cmd"=313, "Rm1St3Dr2Cmd"=314, "Rm1St4Dr2Cmd"=315, "Rm1St5Dr2Cmd"=316, "Rm1St6Dr2Cmd"=317, "Rm1St7Dr2Cmd"=318, "Rm1St8Dr2Cmd"=319, "Rm1St1Dr3Cmd"=320, "Rm1St2Dr3Cmd"=321, "Rm1St3Dr3Cmd"=322, "Rm1St4Dr3Cmd"=323, "Rm1St5Dr3Cmd"=324, "Rm1St6Dr3Cmd"=325, "Rm1St7Dr3Cmd"=326, "Rm1St8Dr3Cmd"=327, "fwRmTempSP"=328, "fwRmHumSP"=329, "fwCoolTempSP"=330, "fwDehumTempSP"=331, "fwRmRun"=332, "fwRmOk"=333, "fwTesting"=334, "fwRmDryP"=335, "fwRmDryI"=336, "fwRmHumP"=337, "fwRmHumI"=338, "fwRmHeatP"=339, "fwRmHeatI"=340, "fwCoolTempP"=341, "fwCoolTempI"=342, "fwDehumTempP"=343, "fwDehumTempI"=344, "fwGndLeak1"=345, "fwGndLeak2"=346, "fwGndLeak3"=347, "fwGndLeak4"=348, "fwGndLeak5"=349, "fwGndLeak6"=350, "fwGndLeak7"=351, "fwGndLeak8"=352, "Rm1OpenerCmd"=353] ("Ring")
            n122 = event-data() -> ("NewVal"=w389:T10)  [unwired: 1 in, 5 out]
            n123 = call-dynamic "Write Single Holding Register.vi"("error in"=w392, "register to write"=w389, "address"=w393, "Modbus master in"=w390) -> ("error out"=w391:errorcluster)  [unwired: 6 in, 1 out]
          }
          event Value Change {
            w400 = T27 299 items=["fwS1Volt1"=0, "fwS1Volt2"=1, "fwS2Volt1"=2, "fwS2Volt2"=3, "fwS3Volt1"=4, "fwS3Volt2"=5, "fwS4Volt1"=6, "fwS4Volt2"=7, "fwS5Volt1"=8, "fwS5Volt2"=9, "fwS6Volt1"=10, "fwS6Volt2 "=11, "fwS7Volt1"=12, "fwS7Volt2"=13, "fwS8Volt1"=14, "fwS8Volt2"=15, "fwRoomHum"=16, "fwRoomTemp"=17, "fwAISpare1"=18, "fwAISpare2"=19, "fwSuppTemp"=20, "fwCoolTemp"=21, "fwDehumTemp"=22, "fwUnused"=23, "Bool Inputs"=24, "gwVoltRate1"=256, "gwVoltRate2"=257, "gwVoltRate3"=258, "gwVoltRate4"=259, "gwVoltRate5"=260, "gwVoltRate6"=261, "gwVoltRate7"=262, "gwVoltRate8"=263, "gwVoltWindow5/1"=264, "gwVoltWindow6/2"=265, "gwVoltWindow7/3"=266, "gwVoltWindow8/4"=267, "fwVoltSet1"=272, "fwVoltSet2"=273, "fwVoltSet3"=274, "fwVoltSet4"=275, "fwVoltSet5"=276, "fwVoltSet6"=277, "fwVoltSet7"=278, "fwVoltSet8"=279, "fwVoltRng1"=280, "fwVoltRng2"=281, "fwVoltRng3"=282, "fwVoltRng4"=283, "fwVoltRng5"=284, "fwVoltRng6"=285, "fwVoltRng7"=286, "fwVoltRng8"=287, "fwVoltPol1"=296, "fwVoltPol2"=297, "fwVoltPol3"=298, "fwVoltPol4"=299, "fwVoltPol5"=300, "fwVoltPol6"=301, "fwVoltPol7"=302, "fwVoltPol8"=303, "Rm1St1Dr1Cmd"=304, "Rm1St2Dr1Cmd"=305, "Rm1St3Dr1Cmd"=306, "Rm1St4Dr1Cmd"=307, "Rm1St5Dr1Cmd"=308, "Rm1St6Dr1Cmd"=309, "Rm1St7Dr1Cmd"=310, "Rm1St8Dr1Cmd"=311, "Rm1St1Dr2Cmd"=312, "Rm1St2Dr2Cmd"=313, "Rm1St3Dr2Cmd"=314, "Rm1St4Dr2Cmd"=315, "Rm1St5Dr2Cmd"=316, "Rm1St6Dr2Cmd"=317, "Rm1St7Dr2Cmd"=318, "Rm1St8Dr2Cmd"=319, "Rm1St1Dr3Cmd"=320, "Rm1St2Dr3Cmd"=321, "Rm1St3Dr3Cmd"=322, "Rm1St4Dr3Cmd"=323, "Rm1St5Dr3Cmd"=324, "Rm1St6Dr3Cmd"=325, "Rm1St7Dr3Cmd"=326, "Rm1St8Dr3Cmd"=327, "fwRmTempSP"=328, "fwRmHumSP"=329, "fwCoolTempSP"=330, "fwDehumTempSP"=331, "fwRmRun"=332, "fwRmOk"=333, "fwTesting"=334, "fwRmDryP"=335, "fwRmDryI"=336, "fwRmHumP"=337, "fwRmHumI"=338, "fwRmHeatP"=339, "fwRmHeatI"=340, "fwCoolTempP"=341, "fwCoolTempI"=342, "fwDehumTempP"=343, "fwDehumTempI"=344, "fwGndLeak1"=345, "fwGndLeak2"=346, "fwGndLeak3"=347, "fwGndLeak4"=348, "fwGndLeak5"=349, "fwGndLeak6"=350, "fwGndLeak7"=351, "fwGndLeak8"=352, "Rm1OpenerCmd"=353] ("Ring")
            n124 = event-data() -> ("NewVal"=w396:T10)  [unwired: 1 in, 5 out]
            n125 = call-dynamic "Write Single Holding Register.vi"("error in"=w399, "register to write"=w396, "address"=w400, "Modbus master in"=w397) -> ("error out"=w398:errorcluster)  [unwired: 6 in, 1 out]
          }
          event Value Change {
            w407 = T27 300 items=["fwS1Volt1"=0, "fwS1Volt2"=1, "fwS2Volt1"=2, "fwS2Volt2"=3, "fwS3Volt1"=4, "fwS3Volt2"=5, "fwS4Volt1"=6, "fwS4Volt2"=7, "fwS5Volt1"=8, "fwS5Volt2"=9, "fwS6Volt1"=10, "fwS6Volt2 "=11, "fwS7Volt1"=12, "fwS7Volt2"=13, "fwS8Volt1"=14, "fwS8Volt2"=15, "fwRoomHum"=16, "fwRoomTemp"=17, "fwAISpare1"=18, "fwAISpare2"=19, "fwSuppTemp"=20, "fwCoolTemp"=21, "fwDehumTemp"=22, "fwUnused"=23, "Bool Inputs"=24, "gwVoltRate1"=256, "gwVoltRate2"=257, "gwVoltRate3"=258, "gwVoltRate4"=259, "gwVoltRate5"=260, "gwVoltRate6"=261, "gwVoltRate7"=262, "gwVoltRate8"=263, "gwVoltWindow5/1"=264, "gwVoltWindow6/2"=265, "gwVoltWindow7/3"=266, "gwVoltWindow8/4"=267, "fwVoltSet1"=272, "fwVoltSet2"=273, "fwVoltSet3"=274, "fwVoltSet4"=275, "fwVoltSet5"=276, "fwVoltSet6"=277, "fwVoltSet7"=278, "fwVoltSet8"=279, "fwVoltRng1"=280, "fwVoltRng2"=281, "fwVoltRng3"=282, "fwVoltRng4"=283, "fwVoltRng5"=284, "fwVoltRng6"=285, "fwVoltRng7"=286, "fwVoltRng8"=287, "fwVoltPol1"=296, "fwVoltPol2"=297, "fwVoltPol3"=298, "fwVoltPol4"=299, "fwVoltPol5"=300, "fwVoltPol6"=301, "fwVoltPol7"=302, "fwVoltPol8"=303, "Rm1St1Dr1Cmd"=304, "Rm1St2Dr1Cmd"=305, "Rm1St3Dr1Cmd"=306, "Rm1St4Dr1Cmd"=307, "Rm1St5Dr1Cmd"=308, "Rm1St6Dr1Cmd"=309, "Rm1St7Dr1Cmd"=310, "Rm1St8Dr1Cmd"=311, "Rm1St1Dr2Cmd"=312, "Rm1St2Dr2Cmd"=313, "Rm1St3Dr2Cmd"=314, "Rm1St4Dr2Cmd"=315, "Rm1St5Dr2Cmd"=316, "Rm1St6Dr2Cmd"=317, "Rm1St7Dr2Cmd"=318, "Rm1St8Dr2Cmd"=319, "Rm1St1Dr3Cmd"=320, "Rm1St2Dr3Cmd"=321, "Rm1St3Dr3Cmd"=322, "Rm1St4Dr3Cmd"=323, "Rm1St5Dr3Cmd"=324, "Rm1St6Dr3Cmd"=325, "Rm1St7Dr3Cmd"=326, "Rm1St8Dr3Cmd"=327, "fwRmTempSP"=328, "fwRmHumSP"=329, "fwCoolTempSP"=330, "fwDehumTempSP"=331, "fwRmRun"=332, "fwRmOk"=333, "fwTesting"=334, "fwRmDryP"=335, "fwRmDryI"=336, "fwRmHumP"=337, "fwRmHumI"=338, "fwRmHeatP"=339, "fwRmHeatI"=340, "fwCoolTempP"=341, "fwCoolTempI"=342, "fwDehumTempP"=343, "fwDehumTempI"=344, "fwGndLeak1"=345, "fwGndLeak2"=346, "fwGndLeak3"=347, "fwGndLeak4"=348, "fwGndLeak5"=349, "fwGndLeak6"=350, "fwGndLeak7"=351, "fwGndLeak8"=352, "Rm1OpenerCmd"=353] ("Ring")
            n126 = event-data() -> ("NewVal"=w403:T10)  [unwired: 1 in, 5 out]
            n127 = call-dynamic "Write Single Holding Register.vi"("error in"=w406, "register to write"=w403, "address"=w407, "Modbus master in"=w404) -> ("error out"=w405:errorcluster)  [unwired: 6 in, 1 out]
          }
          event Value Change {
            w414 = T27 301 items=["fwS1Volt1"=0, "fwS1Volt2"=1, "fwS2Volt1"=2, "fwS2Volt2"=3, "fwS3Volt1"=4, "fwS3Volt2"=5, "fwS4Volt1"=6, "fwS4Volt2"=7, "fwS5Volt1"=8, "fwS5Volt2"=9, "fwS6Volt1"=10, "fwS6Volt2 "=11, "fwS7Volt1"=12, "fwS7Volt2"=13, "fwS8Volt1"=14, "fwS8Volt2"=15, "fwRoomHum"=16, "fwRoomTemp"=17, "fwAISpare1"=18, "fwAISpare2"=19, "fwSuppTemp"=20, "fwCoolTemp"=21, "fwDehumTemp"=22, "fwUnused"=23, "Bool Inputs"=24, "gwVoltRate1"=256, "gwVoltRate2"=257, "gwVoltRate3"=258, "gwVoltRate4"=259, "gwVoltRate5"=260, "gwVoltRate6"=261, "gwVoltRate7"=262, "gwVoltRate8"=263, "gwVoltWindow5/1"=264, "gwVoltWindow6/2"=265, "gwVoltWindow7/3"=266, "gwVoltWindow8/4"=267, "fwVoltSet1"=272, "fwVoltSet2"=273, "fwVoltSet3"=274, "fwVoltSet4"=275, "fwVoltSet5"=276, "fwVoltSet6"=277, "fwVoltSet7"=278, "fwVoltSet8"=279, "fwVoltRng1"=280, "fwVoltRng2"=281, "fwVoltRng3"=282, "fwVoltRng4"=283, "fwVoltRng5"=284, "fwVoltRng6"=285, "fwVoltRng7"=286, "fwVoltRng8"=287, "fwVoltPol1"=296, "fwVoltPol2"=297, "fwVoltPol3"=298, "fwVoltPol4"=299, "fwVoltPol5"=300, "fwVoltPol6"=301, "fwVoltPol7"=302, "fwVoltPol8"=303, "Rm1St1Dr1Cmd"=304, "Rm1St2Dr1Cmd"=305, "Rm1St3Dr1Cmd"=306, "Rm1St4Dr1Cmd"=307, "Rm1St5Dr1Cmd"=308, "Rm1St6Dr1Cmd"=309, "Rm1St7Dr1Cmd"=310, "Rm1St8Dr1Cmd"=311, "Rm1St1Dr2Cmd"=312, "Rm1St2Dr2Cmd"=313, "Rm1St3Dr2Cmd"=314, "Rm1St4Dr2Cmd"=315, "Rm1St5Dr2Cmd"=316, "Rm1St6Dr2Cmd"=317, "Rm1St7Dr2Cmd"=318, "Rm1St8Dr2Cmd"=319, "Rm1St1Dr3Cmd"=320, "Rm1St2Dr3Cmd"=321, "Rm1St3Dr3Cmd"=322, "Rm1St4Dr3Cmd"=323, "Rm1St5Dr3Cmd"=324, "Rm1St6Dr3Cmd"=325, "Rm1St7Dr3Cmd"=326, "Rm1St8Dr3Cmd"=327, "fwRmTempSP"=328, "fwRmHumSP"=329, "fwCoolTempSP"=330, "fwDehumTempSP"=331, "fwRmRun"=332, "fwRmOk"=333, "fwTesting"=334, "fwRmDryP"=335, "fwRmDryI"=336, "fwRmHumP"=337, "fwRmHumI"=338, "fwRmHeatP"=339, "fwRmHeatI"=340, "fwCoolTempP"=341, "fwCoolTempI"=342, "fwDehumTempP"=343, "fwDehumTempI"=344, "fwGndLeak1"=345, "fwGndLeak2"=346, "fwGndLeak3"=347, "fwGndLeak4"=348, "fwGndLeak5"=349, "fwGndLeak6"=350, "fwGndLeak7"=351, "fwGndLeak8"=352, "Rm1OpenerCmd"=353] ("Ring")
            n128 = event-data() -> ("NewVal"=w410:T10)  [unwired: 1 in, 5 out]
            n129 = call-dynamic "Write Single Holding Register.vi"("error in"=w413, "register to write"=w410, "address"=w414, "Modbus master in"=w411) -> ("error out"=w412:errorcluster)  [unwired: 6 in, 1 out]
          }
          event Value Change {
            w421 = T27 302 items=["fwS1Volt1"=0, "fwS1Volt2"=1, "fwS2Volt1"=2, "fwS2Volt2"=3, "fwS3Volt1"=4, "fwS3Volt2"=5, "fwS4Volt1"=6, "fwS4Volt2"=7, "fwS5Volt1"=8, "fwS5Volt2"=9, "fwS6Volt1"=10, "fwS6Volt2 "=11, "fwS7Volt1"=12, "fwS7Volt2"=13, "fwS8Volt1"=14, "fwS8Volt2"=15, "fwRoomHum"=16, "fwRoomTemp"=17, "fwAISpare1"=18, "fwAISpare2"=19, "fwSuppTemp"=20, "fwCoolTemp"=21, "fwDehumTemp"=22, "fwUnused"=23, "Bool Inputs"=24, "gwVoltRate1"=256, "gwVoltRate2"=257, "gwVoltRate3"=258, "gwVoltRate4"=259, "gwVoltRate5"=260, "gwVoltRate6"=261, "gwVoltRate7"=262, "gwVoltRate8"=263, "gwVoltWindow5/1"=264, "gwVoltWindow6/2"=265, "gwVoltWindow7/3"=266, "gwVoltWindow8/4"=267, "fwVoltSet1"=272, "fwVoltSet2"=273, "fwVoltSet3"=274, "fwVoltSet4"=275, "fwVoltSet5"=276, "fwVoltSet6"=277, "fwVoltSet7"=278, "fwVoltSet8"=279, "fwVoltRng1"=280, "fwVoltRng2"=281, "fwVoltRng3"=282, "fwVoltRng4"=283, "fwVoltRng5"=284, "fwVoltRng6"=285, "fwVoltRng7"=286, "fwVoltRng8"=287, "fwVoltPol1"=296, "fwVoltPol2"=297, "fwVoltPol3"=298, "fwVoltPol4"=299, "fwVoltPol5"=300, "fwVoltPol6"=301, "fwVoltPol7"=302, "fwVoltPol8"=303, "Rm1St1Dr1Cmd"=304, "Rm1St2Dr1Cmd"=305, "Rm1St3Dr1Cmd"=306, "Rm1St4Dr1Cmd"=307, "Rm1St5Dr1Cmd"=308, "Rm1St6Dr1Cmd"=309, "Rm1St7Dr1Cmd"=310, "Rm1St8Dr1Cmd"=311, "Rm1St1Dr2Cmd"=312, "Rm1St2Dr2Cmd"=313, "Rm1St3Dr2Cmd"=314, "Rm1St4Dr2Cmd"=315, "Rm1St5Dr2Cmd"=316, "Rm1St6Dr2Cmd"=317, "Rm1St7Dr2Cmd"=318, "Rm1St8Dr2Cmd"=319, "Rm1St1Dr3Cmd"=320, "Rm1St2Dr3Cmd"=321, "Rm1St3Dr3Cmd"=322, "Rm1St4Dr3Cmd"=323, "Rm1St5Dr3Cmd"=324, "Rm1St6Dr3Cmd"=325, "Rm1St7Dr3Cmd"=326, "Rm1St8Dr3Cmd"=327, "fwRmTempSP"=328, "fwRmHumSP"=329, "fwCoolTempSP"=330, "fwDehumTempSP"=331, "fwRmRun"=332, "fwRmOk"=333, "fwTesting"=334, "fwRmDryP"=335, "fwRmDryI"=336, "fwRmHumP"=337, "fwRmHumI"=338, "fwRmHeatP"=339, "fwRmHeatI"=340, "fwCoolTempP"=341, "fwCoolTempI"=342, "fwDehumTempP"=343, "fwDehumTempI"=344, "fwGndLeak1"=345, "fwGndLeak2"=346, "fwGndLeak3"=347, "fwGndLeak4"=348, "fwGndLeak5"=349, "fwGndLeak6"=350, "fwGndLeak7"=351, "fwGndLeak8"=352, "Rm1OpenerCmd"=353] ("Ring")
            n130 = event-data() -> ("NewVal"=w417:T10)  [unwired: 1 in, 5 out]
            n131 = call-dynamic "Write Single Holding Register.vi"("error in"=w420, "register to write"=w417, "address"=w421, "Modbus master in"=w418) -> ("error out"=w419:errorcluster)  [unwired: 6 in, 1 out]
          }
          event Value Change {
            w430 = T27 303 items=["fwS1Volt1"=0, "fwS1Volt2"=1, "fwS2Volt1"=2, "fwS2Volt2"=3, "fwS3Volt1"=4, "fwS3Volt2"=5, "fwS4Volt1"=6, "fwS4Volt2"=7, "fwS5Volt1"=8, "fwS5Volt2"=9, "fwS6Volt1"=10, "fwS6Volt2 "=11, "fwS7Volt1"=12, "fwS7Volt2"=13, "fwS8Volt1"=14, "fwS8Volt2"=15, "fwRoomHum"=16, "fwRoomTemp"=17, "fwAISpare1"=18, "fwAISpare2"=19, "fwSuppTemp"=20, "fwCoolTemp"=21, "fwDehumTemp"=22, "fwUnused"=23, "Bool Inputs"=24, "gwVoltRate1"=256, "gwVoltRate2"=257, "gwVoltRate3"=258, "gwVoltRate4"=259, "gwVoltRate5"=260, "gwVoltRate6"=261, "gwVoltRate7"=262, "gwVoltRate8"=263, "gwVoltWindow5/1"=264, "gwVoltWindow6/2"=265, "gwVoltWindow7/3"=266, "gwVoltWindow8/4"=267, "fwVoltSet1"=272, "fwVoltSet2"=273, "fwVoltSet3"=274, "fwVoltSet4"=275, "fwVoltSet5"=276, "fwVoltSet6"=277, "fwVoltSet7"=278, "fwVoltSet8"=279, "fwVoltRng1"=280, "fwVoltRng2"=281, "fwVoltRng3"=282, "fwVoltRng4"=283, "fwVoltRng5"=284, "fwVoltRng6"=285, "fwVoltRng7"=286, "fwVoltRng8"=287, "fwVoltPol1"=296, "fwVoltPol2"=297, "fwVoltPol3"=298, "fwVoltPol4"=299, "fwVoltPol5"=300, "fwVoltPol6"=301, "fwVoltPol7"=302, "fwVoltPol8"=303, "Rm1St1Dr1Cmd"=304, "Rm1St2Dr1Cmd"=305, "Rm1St3Dr1Cmd"=306, "Rm1St4Dr1Cmd"=307, "Rm1St5Dr1Cmd"=308, "Rm1St6Dr1Cmd"=309, "Rm1St7Dr1Cmd"=310, "Rm1St8Dr1Cmd"=311, "Rm1St1Dr2Cmd"=312, "Rm1St2Dr2Cmd"=313, "Rm1St3Dr2Cmd"=314, "Rm1St4Dr2Cmd"=315, "Rm1St5Dr2Cmd"=316, "Rm1St6Dr2Cmd"=317, "Rm1St7Dr2Cmd"=318, "Rm1St8Dr2Cmd"=319, "Rm1St1Dr3Cmd"=320, "Rm1St2Dr3Cmd"=321, "Rm1St3Dr3Cmd"=322, "Rm1St4Dr3Cmd"=323, "Rm1St5Dr3Cmd"=324, "Rm1St6Dr3Cmd"=325, "Rm1St7Dr3Cmd"=326, "Rm1St8Dr3Cmd"=327, "fwRmTempSP"=328, "fwRmHumSP"=329, "fwCoolTempSP"=330, "fwDehumTempSP"=331, "fwRmRun"=332, "fwRmOk"=333, "fwTesting"=334, "fwRmDryP"=335, "fwRmDryI"=336, "fwRmHumP"=337, "fwRmHumI"=338, "fwRmHeatP"=339, "fwRmHeatI"=340, "fwCoolTempP"=341, "fwCoolTempI"=342, "fwDehumTempP"=343, "fwDehumTempI"=344, "fwGndLeak1"=345, "fwGndLeak2"=346, "fwGndLeak3"=347, "fwGndLeak4"=348, "fwGndLeak5"=349, "fwGndLeak6"=350, "fwGndLeak7"=351, "fwGndLeak8"=352, "Rm1OpenerCmd"=353] ("Ring")
            n132 = event-data() -> ("NewVal"=w426:T10)  [unwired: 1 in, 5 out]
            n133 = call-dynamic "Write Single Holding Register.vi"("error in"=w427, "register to write"=w426, "address"=w430, "Modbus master in"=w428) -> ("error out"=w429:errorcluster)  [unwired: 6 in, 1 out]
          }
          event "Station Voltage Send 1": Value Change {
            n134 = event-data() -> ()  [unwired: 1 in, 6 out]
            n135 = call "RTS Voltage Frequency Selector.vi"("Frequency"="Frequency", "Station Number"=u16 1, "Voltage"="Voltage", "error in (no error)"=w436, "Modbus Master in"=w435) -> ("error out"=w434:errorcluster)  [unwired: 5 in, 1 out]
          }
          event "Station Voltage Send 2": Value Change {
            n136 = event-data() -> ()  [unwired: 1 in, 6 out]
            n137 = call "RTS Voltage Frequency Selector.vi"("Frequency"="Frequency 2", "Station Number"=u16 2, "Voltage"="Voltage 2", "error in (no error)"=w443, "Modbus Master in"=w441) -> ("error out"=w442:errorcluster)  [unwired: 5 in, 1 out]
          }
          event "Station Voltage Send 3": Value Change {
            n138 = event-data() -> ()  [unwired: 1 in, 6 out]
            n139 = call "RTS Voltage Frequency Selector.vi"("Frequency"="Frequency 3", "Station Number"=u16 3, "Voltage"="Voltage 3", "error in (no error)"=w451, "Modbus Master in"=w449) -> ("error out"=w450:errorcluster)  [unwired: 5 in, 1 out]
          }
          event "Station Voltage Send 4": Value Change {
            n140 = event-data() -> ()  [unwired: 1 in, 6 out]
            n141 = call "RTS Voltage Frequency Selector.vi"("Frequency"="Frequency 4", "Station Number"=u16 4, "Voltage"="Voltage 4", "error in (no error)"=w459, "Modbus Master in"=w460) -> ("error out"=w458:errorcluster)  [unwired: 5 in, 1 out]
          }
          event "Station Voltage Send 5": Value Change {
            n142 = event-data() -> ()  [unwired: 1 in, 6 out]
            n143 = call "RTS Voltage Frequency Selector.vi"("Frequency"="Frequency 5", "Station Number"=u16 5, "Voltage"="Voltage 5", "error in (no error)"=w467, "Modbus Master in"=w465) -> ("error out"=w466:errorcluster)  [unwired: 5 in, 1 out]
          }
          event "Station Voltage Send 6": Value Change {
            n144 = event-data() -> ()  [unwired: 1 in, 6 out]
            n145 = call "RTS Voltage Frequency Selector.vi"("Frequency"="Frequency 6", "Station Number"=u16 6, "Voltage"="Voltage 6", "error in (no error)"=w472, "Modbus Master in"=w475) -> ("error out"=w471:errorcluster)  [unwired: 5 in, 1 out]
          }
          event "Station Voltage Send 7": Value Change {
            n146 = event-data() -> ()  [unwired: 1 in, 6 out]
            n147 = call "RTS Voltage Frequency Selector.vi"("Frequency"="Frequency 7", "Station Number"=u16 7, "Voltage"="Voltage 7", "error in (no error)"=w480, "Modbus Master in"=w483) -> ("error out"=w479:errorcluster)  [unwired: 5 in, 1 out]
          }
          event "Station Voltage Send 8": Value Change {
            n148 = event-data() -> ()  [unwired: 1 in, 6 out]
            n149 = call "RTS Voltage Frequency Selector.vi"("Frequency"="Frequency 8", "Station Number"=u16 8, "Voltage"="Voltage 8", "error in (no error)"=w488, "Modbus Master in"=w491) -> ("error out"=w487:errorcluster)  [unwired: 5 in, 1 out]
          }
          event "Station 4 CMD": Value Change {
            w506 = T27 323 items=["fwS1Volt1"=0, "fwS1Volt2"=1, "fwS2Volt1"=2, "fwS2Volt2"=3, "fwS3Volt1"=4, "fwS3Volt2"=5, "fwS4Volt1"=6, "fwS4Volt2"=7, "fwS5Volt1"=8, "fwS5Volt2"=9, "fwS6Volt1"=10, "fwS6Volt2 "=11, "fwS7Volt1"=12, "fwS7Volt2"=13, "fwS8Volt1"=14, "fwS8Volt2"=15, "fwRoomHum"=16, "fwRoomTemp"=17, "fwAISpare1"=18, "fwAISpare2"=19, "fwSuppTemp"=20, "fwCoolTemp"=21, "fwDehumTemp"=22, "fwUnused"=23, "Bool Inputs"=24, "gwVoltRate1"=256, "gwVoltRate2"=257, "gwVoltRate3"=258, "gwVoltRate4"=259, "gwVoltRate5"=260, "gwVoltRate6"=261, "gwVoltRate7"=262, "gwVoltRate8"=263, "gwVoltWindow5/1"=264, "gwVoltWindow6/2"=265, "gwVoltWindow7/3"=266, "gwVoltWindow8/4"=267, "fwVoltSet1"=272, "fwVoltSet2"=273, "fwVoltSet3"=274, "fwVoltSet4"=275, "fwVoltSet5"=276, "fwVoltSet6"=277, "fwVoltSet7"=278, "fwVoltSet8"=279, "fwVoltRng1"=280, "fwVoltRng2"=281, "fwVoltRng3"=282, "fwVoltRng4"=283, "fwVoltRng5"=284, "fwVoltRng6"=285, "fwVoltRng7"=286, "fwVoltRng8"=287, "fwVoltPol1"=296, "fwVoltPol2"=297, "fwVoltPol3"=298, "fwVoltPol4"=299, "fwVoltPol5"=300, "fwVoltPol6"=301, "fwVoltPol7"=302, "fwVoltPol8"=303, "Rm1St1Dr1Cmd"=304, "Rm1St2Dr1Cmd"=305, "Rm1St3Dr1Cmd"=306, "Rm1St4Dr1Cmd"=307, "Rm1St5Dr1Cmd"=308, "Rm1St6Dr1Cmd"=309, "Rm1St7Dr1Cmd"=310, "Rm1St8Dr1Cmd"=311, "Rm1St1Dr2Cmd"=312, "Rm1St2Dr2Cmd"=313, "Rm1St3Dr2Cmd"=314, "Rm1St4Dr2Cmd"=315, "Rm1St5Dr2Cmd"=316, "Rm1St6Dr2Cmd"=317, "Rm1St7Dr2Cmd"=318, "Rm1St8Dr2Cmd"=319, "Rm1St1Dr3Cmd"=320, "Rm1St2Dr3Cmd"=321, "Rm1St3Dr3Cmd"=322, "Rm1St4Dr3Cmd"=323, "Rm1St5Dr3Cmd"=324, "Rm1St6Dr3Cmd"=325, "Rm1St7Dr3Cmd"=326, "Rm1St8Dr3Cmd"=327, "fwRmTempSP"=328, "fwRmHumSP"=329, "fwCoolTempSP"=330, "fwDehumTempSP"=331, "fwRmRun"=332, "fwRmOk"=333, "fwTesting"=334, "fwRmDryP"=335, "fwRmDryI"=336, "fwRmHumP"=337, "fwRmHumI"=338, "fwRmHeatP"=339, "fwRmHeatI"=340, "fwCoolTempP"=341, "fwCoolTempI"=342, "fwDehumTempP"=343, "fwDehumTempI"=344, "fwGndLeak1"=345, "fwGndLeak2"=346, "fwGndLeak3"=347, "fwGndLeak4"=348, "fwGndLeak5"=349, "fwGndLeak6"=350, "fwGndLeak7"=351, "fwGndLeak8"=352, "Rm1OpenerCmd"=353] ("Ring")
            w507 = T27 315 items=["fwS1Volt1"=0, "fwS1Volt2"=1, "fwS2Volt1"=2, "fwS2Volt2"=3, "fwS3Volt1"=4, "fwS3Volt2"=5, "fwS4Volt1"=6, "fwS4Volt2"=7, "fwS5Volt1"=8, "fwS5Volt2"=9, "fwS6Volt1"=10, "fwS6Volt2 "=11, "fwS7Volt1"=12, "fwS7Volt2"=13, "fwS8Volt1"=14, "fwS8Volt2"=15, "fwRoomHum"=16, "fwRoomTemp"=17, "fwAISpare1"=18, "fwAISpare2"=19, "fwSuppTemp"=20, "fwCoolTemp"=21, "fwDehumTemp"=22, "fwUnused"=23, "Bool Inputs"=24, "gwVoltRate1"=256, "gwVoltRate2"=257, "gwVoltRate3"=258, "gwVoltRate4"=259, "gwVoltRate5"=260, "gwVoltRate6"=261, "gwVoltRate7"=262, "gwVoltRate8"=263, "gwVoltWindow5/1"=264, "gwVoltWindow6/2"=265, "gwVoltWindow7/3"=266, "gwVoltWindow8/4"=267, "fwVoltSet1"=272, "fwVoltSet2"=273, "fwVoltSet3"=274, "fwVoltSet4"=275, "fwVoltSet5"=276, "fwVoltSet6"=277, "fwVoltSet7"=278, "fwVoltSet8"=279, "fwVoltRng1"=280, "fwVoltRng2"=281, "fwVoltRng3"=282, "fwVoltRng4"=283, "fwVoltRng5"=284, "fwVoltRng6"=285, "fwVoltRng7"=286, "fwVoltRng8"=287, "fwVoltPol1"=296, "fwVoltPol2"=297, "fwVoltPol3"=298, "fwVoltPol4"=299, "fwVoltPol5"=300, "fwVoltPol6"=301, "fwVoltPol7"=302, "fwVoltPol8"=303, "Rm1St1Dr1Cmd"=304, "Rm1St2Dr1Cmd"=305, "Rm1St3Dr1Cmd"=306, "Rm1St4Dr1Cmd"=307, "Rm1St5Dr1Cmd"=308, "Rm1St6Dr1Cmd"=309, "Rm1St7Dr1Cmd"=310, "Rm1St8Dr1Cmd"=311, "Rm1St1Dr2Cmd"=312, "Rm1St2Dr2Cmd"=313, "Rm1St3Dr2Cmd"=314, "Rm1St4Dr2Cmd"=315, "Rm1St5Dr2Cmd"=316, "Rm1St6Dr2Cmd"=317, "Rm1St7Dr2Cmd"=318, "Rm1St8Dr2Cmd"=319, "Rm1St1Dr3Cmd"=320, "Rm1St2Dr3Cmd"=321, "Rm1St3Dr3Cmd"=322, "Rm1St4Dr3Cmd"=323, "Rm1St5Dr3Cmd"=324, "Rm1St6Dr3Cmd"=325, "Rm1St7Dr3Cmd"=326, "Rm1St8Dr3Cmd"=327, "fwRmTempSP"=328, "fwRmHumSP"=329, "fwCoolTempSP"=330, "fwDehumTempSP"=331, "fwRmRun"=332, "fwRmOk"=333, "fwTesting"=334, "fwRmDryP"=335, "fwRmDryI"=336, "fwRmHumP"=337, "fwRmHumI"=338, "fwRmHeatP"=339, "fwRmHeatI"=340, "fwCoolTempP"=341, "fwCoolTempI"=342, "fwDehumTempP"=343, "fwDehumTempI"=344, "fwGndLeak1"=345, "fwGndLeak2"=346, "fwGndLeak3"=347, "fwGndLeak4"=348, "fwGndLeak5"=349, "fwGndLeak6"=350, "fwGndLeak7"=351, "fwGndLeak8"=352, "Rm1OpenerCmd"=353] ("Ring")
            w508 = T27 307 items=["fwS1Volt1"=0, "fwS1Volt2"=1, "fwS2Volt1"=2, "fwS2Volt2"=3, "fwS3Volt1"=4, "fwS3Volt2"=5, "fwS4Volt1"=6, "fwS4Volt2"=7, "fwS5Volt1"=8, "fwS5Volt2"=9, "fwS6Volt1"=10, "fwS6Volt2 "=11, "fwS7Volt1"=12, "fwS7Volt2"=13, "fwS8Volt1"=14, "fwS8Volt2"=15, "fwRoomHum"=16, "fwRoomTemp"=17, "fwAISpare1"=18, "fwAISpare2"=19, "fwSuppTemp"=20, "fwCoolTemp"=21, "fwDehumTemp"=22, "fwUnused"=23, "Bool Inputs"=24, "gwVoltRate1"=256, "gwVoltRate2"=257, "gwVoltRate3"=258, "gwVoltRate4"=259, "gwVoltRate5"=260, "gwVoltRate6"=261, "gwVoltRate7"=262, "gwVoltRate8"=263, "gwVoltWindow5/1"=264, "gwVoltWindow6/2"=265, "gwVoltWindow7/3"=266, "gwVoltWindow8/4"=267, "fwVoltSet1"=272, "fwVoltSet2"=273, "fwVoltSet3"=274, "fwVoltSet4"=275, "fwVoltSet5"=276, "fwVoltSet6"=277, "fwVoltSet7"=278, "fwVoltSet8"=279, "fwVoltRng1"=280, "fwVoltRng2"=281, "fwVoltRng3"=282, "fwVoltRng4"=283, "fwVoltRng5"=284, "fwVoltRng6"=285, "fwVoltRng7"=286, "fwVoltRng8"=287, "fwVoltPol1"=296, "fwVoltPol2"=297, "fwVoltPol3"=298, "fwVoltPol4"=299, "fwVoltPol5"=300, "fwVoltPol6"=301, "fwVoltPol7"=302, "fwVoltPol8"=303, "Rm1St1Dr1Cmd"=304, "Rm1St2Dr1Cmd"=305, "Rm1St3Dr1Cmd"=306, "Rm1St4Dr1Cmd"=307, "Rm1St5Dr1Cmd"=308, "Rm1St6Dr1Cmd"=309, "Rm1St7Dr1Cmd"=310, "Rm1St8Dr1Cmd"=311, "Rm1St1Dr2Cmd"=312, "Rm1St2Dr2Cmd"=313, "Rm1St3Dr2Cmd"=314, "Rm1St4Dr2Cmd"=315, "Rm1St5Dr2Cmd"=316, "Rm1St6Dr2Cmd"=317, "Rm1St7Dr2Cmd"=318, "Rm1St8Dr2Cmd"=319, "Rm1St1Dr3Cmd"=320, "Rm1St2Dr3Cmd"=321, "Rm1St3Dr3Cmd"=322, "Rm1St4Dr3Cmd"=323, "Rm1St5Dr3Cmd"=324, "Rm1St6Dr3Cmd"=325, "Rm1St7Dr3Cmd"=326, "Rm1St8Dr3Cmd"=327, "fwRmTempSP"=328, "fwRmHumSP"=329, "fwCoolTempSP"=330, "fwDehumTempSP"=331, "fwRmRun"=332, "fwRmOk"=333, "fwTesting"=334, "fwRmDryP"=335, "fwRmDryI"=336, "fwRmHumP"=337, "fwRmHumI"=338, "fwRmHeatP"=339, "fwRmHeatI"=340, "fwCoolTempP"=341, "fwCoolTempI"=342, "fwDehumTempP"=343, "fwDehumTempI"=344, "fwGndLeak1"=345, "fwGndLeak2"=346, "fwGndLeak3"=347, "fwGndLeak4"=348, "fwGndLeak5"=349, "fwGndLeak6"=350, "fwGndLeak7"=351, "fwGndLeak8"=352, "Rm1OpenerCmd"=353] ("Ring")
            n150 = event-data() -> ()  [unwired: 1 in, 6 out]
            n151 = local read "Door Settings"() -> (w498:T11)
            n152 = Unbundle By Name(w498) -> ("Station 4.Slide"=w501:T13, "Station 4.Cab"=w502:T13, "Station 4.Freezer"=w503:T13)
            n153 = call-dynamic "Write Single Holding Register.vi"("error in"=w496, "register to write"=w503, "address"=w508, "Modbus master in"=w495) -> ("error out"=w500:errorcluster, "Modbus master out"=w505:refnum<class "Modbus Master.lvclass">)  [unwired: 6 in]
            n154 = call-dynamic "Write Single Holding Register.vi"("error in"=w500, "register to write"=w502, "address"=w507, "Modbus master in"=w505) -> ("error out"=w499:errorcluster, "Modbus master out"=w504:refnum<class "Modbus Master.lvclass">)  [unwired: 6 in]
            n155 = call-dynamic "Write Single Holding Register.vi"("error in"=w499, "register to write"=w501, "address"=w506, "Modbus master in"=w504) -> ("error out"=w497:errorcluster)  [unwired: 6 in, 1 out]
          }
          event "Station 5 CMD": Value Change {
            w524 = T27 324 items=["fwS1Volt1"=0, "fwS1Volt2"=1, "fwS2Volt1"=2, "fwS2Volt2"=3, "fwS3Volt1"=4, "fwS3Volt2"=5, "fwS4Volt1"=6, "fwS4Volt2"=7, "fwS5Volt1"=8, "fwS5Volt2"=9, "fwS6Volt1"=10, "fwS6Volt2 "=11, "fwS7Volt1"=12, "fwS7Volt2"=13, "fwS8Volt1"=14, "fwS8Volt2"=15, "fwRoomHum"=16, "fwRoomTemp"=17, "fwAISpare1"=18, "fwAISpare2"=19, "fwSuppTemp"=20, "fwCoolTemp"=21, "fwDehumTemp"=22, "fwUnused"=23, "Bool Inputs"=24, "gwVoltRate1"=256, "gwVoltRate2"=257, "gwVoltRate3"=258, "gwVoltRate4"=259, "gwVoltRate5"=260, "gwVoltRate6"=261, "gwVoltRate7"=262, "gwVoltRate8"=263, "gwVoltWindow5/1"=264, "gwVoltWindow6/2"=265, "gwVoltWindow7/3"=266, "gwVoltWindow8/4"=267, "fwVoltSet1"=272, "fwVoltSet2"=273, "fwVoltSet3"=274, "fwVoltSet4"=275, "fwVoltSet5"=276, "fwVoltSet6"=277, "fwVoltSet7"=278, "fwVoltSet8"=279, "fwVoltRng1"=280, "fwVoltRng2"=281, "fwVoltRng3"=282, "fwVoltRng4"=283, "fwVoltRng5"=284, "fwVoltRng6"=285, "fwVoltRng7"=286, "fwVoltRng8"=287, "fwVoltPol1"=296, "fwVoltPol2"=297, "fwVoltPol3"=298, "fwVoltPol4"=299, "fwVoltPol5"=300, "fwVoltPol6"=301, "fwVoltPol7"=302, "fwVoltPol8"=303, "Rm1St1Dr1Cmd"=304, "Rm1St2Dr1Cmd"=305, "Rm1St3Dr1Cmd"=306, "Rm1St4Dr1Cmd"=307, "Rm1St5Dr1Cmd"=308, "Rm1St6Dr1Cmd"=309, "Rm1St7Dr1Cmd"=310, "Rm1St8Dr1Cmd"=311, "Rm1St1Dr2Cmd"=312, "Rm1St2Dr2Cmd"=313, "Rm1St3Dr2Cmd"=314, "Rm1St4Dr2Cmd"=315, "Rm1St5Dr2Cmd"=316, "Rm1St6Dr2Cmd"=317, "Rm1St7Dr2Cmd"=318, "Rm1St8Dr2Cmd"=319, "Rm1St1Dr3Cmd"=320, "Rm1St2Dr3Cmd"=321, "Rm1St3Dr3Cmd"=322, "Rm1St4Dr3Cmd"=323, "Rm1St5Dr3Cmd"=324, "Rm1St6Dr3Cmd"=325, "Rm1St7Dr3Cmd"=326, "Rm1St8Dr3Cmd"=327, "fwRmTempSP"=328, "fwRmHumSP"=329, "fwCoolTempSP"=330, "fwDehumTempSP"=331, "fwRmRun"=332, "fwRmOk"=333, "fwTesting"=334, "fwRmDryP"=335, "fwRmDryI"=336, "fwRmHumP"=337, "fwRmHumI"=338, "fwRmHeatP"=339, "fwRmHeatI"=340, "fwCoolTempP"=341, "fwCoolTempI"=342, "fwDehumTempP"=343, "fwDehumTempI"=344, "fwGndLeak1"=345, "fwGndLeak2"=346, "fwGndLeak3"=347, "fwGndLeak4"=348, "fwGndLeak5"=349, "fwGndLeak6"=350, "fwGndLeak7"=351, "fwGndLeak8"=352, "Rm1OpenerCmd"=353] ("Ring")
            w525 = T27 316 items=["fwS1Volt1"=0, "fwS1Volt2"=1, "fwS2Volt1"=2, "fwS2Volt2"=3, "fwS3Volt1"=4, "fwS3Volt2"=5, "fwS4Volt1"=6, "fwS4Volt2"=7, "fwS5Volt1"=8, "fwS5Volt2"=9, "fwS6Volt1"=10, "fwS6Volt2 "=11, "fwS7Volt1"=12, "fwS7Volt2"=13, "fwS8Volt1"=14, "fwS8Volt2"=15, "fwRoomHum"=16, "fwRoomTemp"=17, "fwAISpare1"=18, "fwAISpare2"=19, "fwSuppTemp"=20, "fwCoolTemp"=21, "fwDehumTemp"=22, "fwUnused"=23, "Bool Inputs"=24, "gwVoltRate1"=256, "gwVoltRate2"=257, "gwVoltRate3"=258, "gwVoltRate4"=259, "gwVoltRate5"=260, "gwVoltRate6"=261, "gwVoltRate7"=262, "gwVoltRate8"=263, "gwVoltWindow5/1"=264, "gwVoltWindow6/2"=265, "gwVoltWindow7/3"=266, "gwVoltWindow8/4"=267, "fwVoltSet1"=272, "fwVoltSet2"=273, "fwVoltSet3"=274, "fwVoltSet4"=275, "fwVoltSet5"=276, "fwVoltSet6"=277, "fwVoltSet7"=278, "fwVoltSet8"=279, "fwVoltRng1"=280, "fwVoltRng2"=281, "fwVoltRng3"=282, "fwVoltRng4"=283, "fwVoltRng5"=284, "fwVoltRng6"=285, "fwVoltRng7"=286, "fwVoltRng8"=287, "fwVoltPol1"=296, "fwVoltPol2"=297, "fwVoltPol3"=298, "fwVoltPol4"=299, "fwVoltPol5"=300, "fwVoltPol6"=301, "fwVoltPol7"=302, "fwVoltPol8"=303, "Rm1St1Dr1Cmd"=304, "Rm1St2Dr1Cmd"=305, "Rm1St3Dr1Cmd"=306, "Rm1St4Dr1Cmd"=307, "Rm1St5Dr1Cmd"=308, "Rm1St6Dr1Cmd"=309, "Rm1St7Dr1Cmd"=310, "Rm1St8Dr1Cmd"=311, "Rm1St1Dr2Cmd"=312, "Rm1St2Dr2Cmd"=313, "Rm1St3Dr2Cmd"=314, "Rm1St4Dr2Cmd"=315, "Rm1St5Dr2Cmd"=316, "Rm1St6Dr2Cmd"=317, "Rm1St7Dr2Cmd"=318, "Rm1St8Dr2Cmd"=319, "Rm1St1Dr3Cmd"=320, "Rm1St2Dr3Cmd"=321, "Rm1St3Dr3Cmd"=322, "Rm1St4Dr3Cmd"=323, "Rm1St5Dr3Cmd"=324, "Rm1St6Dr3Cmd"=325, "Rm1St7Dr3Cmd"=326, "Rm1St8Dr3Cmd"=327, "fwRmTempSP"=328, "fwRmHumSP"=329, "fwCoolTempSP"=330, "fwDehumTempSP"=331, "fwRmRun"=332, "fwRmOk"=333, "fwTesting"=334, "fwRmDryP"=335, "fwRmDryI"=336, "fwRmHumP"=337, "fwRmHumI"=338, "fwRmHeatP"=339, "fwRmHeatI"=340, "fwCoolTempP"=341, "fwCoolTempI"=342, "fwDehumTempP"=343, "fwDehumTempI"=344, "fwGndLeak1"=345, "fwGndLeak2"=346, "fwGndLeak3"=347, "fwGndLeak4"=348, "fwGndLeak5"=349, "fwGndLeak6"=350, "fwGndLeak7"=351, "fwGndLeak8"=352, "Rm1OpenerCmd"=353] ("Ring")
            w526 = T27 308 items=["fwS1Volt1"=0, "fwS1Volt2"=1, "fwS2Volt1"=2, "fwS2Volt2"=3, "fwS3Volt1"=4, "fwS3Volt2"=5, "fwS4Volt1"=6, "fwS4Volt2"=7, "fwS5Volt1"=8, "fwS5Volt2"=9, "fwS6Volt1"=10, "fwS6Volt2 "=11, "fwS7Volt1"=12, "fwS7Volt2"=13, "fwS8Volt1"=14, "fwS8Volt2"=15, "fwRoomHum"=16, "fwRoomTemp"=17, "fwAISpare1"=18, "fwAISpare2"=19, "fwSuppTemp"=20, "fwCoolTemp"=21, "fwDehumTemp"=22, "fwUnused"=23, "Bool Inputs"=24, "gwVoltRate1"=256, "gwVoltRate2"=257, "gwVoltRate3"=258, "gwVoltRate4"=259, "gwVoltRate5"=260, "gwVoltRate6"=261, "gwVoltRate7"=262, "gwVoltRate8"=263, "gwVoltWindow5/1"=264, "gwVoltWindow6/2"=265, "gwVoltWindow7/3"=266, "gwVoltWindow8/4"=267, "fwVoltSet1"=272, "fwVoltSet2"=273, "fwVoltSet3"=274, "fwVoltSet4"=275, "fwVoltSet5"=276, "fwVoltSet6"=277, "fwVoltSet7"=278, "fwVoltSet8"=279, "fwVoltRng1"=280, "fwVoltRng2"=281, "fwVoltRng3"=282, "fwVoltRng4"=283, "fwVoltRng5"=284, "fwVoltRng6"=285, "fwVoltRng7"=286, "fwVoltRng8"=287, "fwVoltPol1"=296, "fwVoltPol2"=297, "fwVoltPol3"=298, "fwVoltPol4"=299, "fwVoltPol5"=300, "fwVoltPol6"=301, "fwVoltPol7"=302, "fwVoltPol8"=303, "Rm1St1Dr1Cmd"=304, "Rm1St2Dr1Cmd"=305, "Rm1St3Dr1Cmd"=306, "Rm1St4Dr1Cmd"=307, "Rm1St5Dr1Cmd"=308, "Rm1St6Dr1Cmd"=309, "Rm1St7Dr1Cmd"=310, "Rm1St8Dr1Cmd"=311, "Rm1St1Dr2Cmd"=312, "Rm1St2Dr2Cmd"=313, "Rm1St3Dr2Cmd"=314, "Rm1St4Dr2Cmd"=315, "Rm1St5Dr2Cmd"=316, "Rm1St6Dr2Cmd"=317, "Rm1St7Dr2Cmd"=318, "Rm1St8Dr2Cmd"=319, "Rm1St1Dr3Cmd"=320, "Rm1St2Dr3Cmd"=321, "Rm1St3Dr3Cmd"=322, "Rm1St4Dr3Cmd"=323, "Rm1St5Dr3Cmd"=324, "Rm1St6Dr3Cmd"=325, "Rm1St7Dr3Cmd"=326, "Rm1St8Dr3Cmd"=327, "fwRmTempSP"=328, "fwRmHumSP"=329, "fwCoolTempSP"=330, "fwDehumTempSP"=331, "fwRmRun"=332, "fwRmOk"=333, "fwTesting"=334, "fwRmDryP"=335, "fwRmDryI"=336, "fwRmHumP"=337, "fwRmHumI"=338, "fwRmHeatP"=339, "fwRmHeatI"=340, "fwCoolTempP"=341, "fwCoolTempI"=342, "fwDehumTempP"=343, "fwDehumTempI"=344, "fwGndLeak1"=345, "fwGndLeak2"=346, "fwGndLeak3"=347, "fwGndLeak4"=348, "fwGndLeak5"=349, "fwGndLeak6"=350, "fwGndLeak7"=351, "fwGndLeak8"=352, "Rm1OpenerCmd"=353] ("Ring")
            n156 = event-data() -> ()  [unwired: 1 in, 6 out]
            n157 = local read "Door Settings"() -> (w516:T11)
            n158 = Unbundle By Name(w516) -> ("Station 5.Slide"=w519:T13, "Station 5.Cab"=w520:T13, "Station 5.Freezer"=w521:T13)
            n159 = call-dynamic "Write Single Holding Register.vi"("error in"=w514, "register to write"=w521, "address"=w526, "Modbus master in"=w513) -> ("error out"=w518:errorcluster, "Modbus master out"=w523:refnum<class "Modbus Master.lvclass">)  [unwired: 6 in]
            n160 = call-dynamic "Write Single Holding Register.vi"("error in"=w518, "register to write"=w520, "address"=w525, "Modbus master in"=w523) -> ("error out"=w517:errorcluster, "Modbus master out"=w522:refnum<class "Modbus Master.lvclass">)  [unwired: 6 in]
            n161 = call-dynamic "Write Single Holding Register.vi"("error in"=w517, "register to write"=w519, "address"=w524, "Modbus master in"=w522) -> ("error out"=w515:errorcluster)  [unwired: 6 in, 1 out]
          }
          event "Station 6 CMD": Value Change {
            w538 = T27 325 items=["fwS1Volt1"=0, "fwS1Volt2"=1, "fwS2Volt1"=2, "fwS2Volt2"=3, "fwS3Volt1"=4, "fwS3Volt2"=5, "fwS4Volt1"=6, "fwS4Volt2"=7, "fwS5Volt1"=8, "fwS5Volt2"=9, "fwS6Volt1"=10, "fwS6Volt2 "=11, "fwS7Volt1"=12, "fwS7Volt2"=13, "fwS8Volt1"=14, "fwS8Volt2"=15, "fwRoomHum"=16, "fwRoomTemp"=17, "fwAISpare1"=18, "fwAISpare2"=19, "fwSuppTemp"=20, "fwCoolTemp"=21, "fwDehumTemp"=22, "fwUnused"=23, "Bool Inputs"=24, "gwVoltRate1"=256, "gwVoltRate2"=257, "gwVoltRate3"=258, "gwVoltRate4"=259, "gwVoltRate5"=260, "gwVoltRate6"=261, "gwVoltRate7"=262, "gwVoltRate8"=263, "gwVoltWindow5/1"=264, "gwVoltWindow6/2"=265, "gwVoltWindow7/3"=266, "gwVoltWindow8/4"=267, "fwVoltSet1"=272, "fwVoltSet2"=273, "fwVoltSet3"=274, "fwVoltSet4"=275, "fwVoltSet5"=276, "fwVoltSet6"=277, "fwVoltSet7"=278, "fwVoltSet8"=279, "fwVoltRng1"=280, "fwVoltRng2"=281, "fwVoltRng3"=282, "fwVoltRng4"=283, "fwVoltRng5"=284, "fwVoltRng6"=285, "fwVoltRng7"=286, "fwVoltRng8"=287, "fwVoltPol1"=296, "fwVoltPol2"=297, "fwVoltPol3"=298, "fwVoltPol4"=299, "fwVoltPol5"=300, "fwVoltPol6"=301, "fwVoltPol7"=302, "fwVoltPol8"=303, "Rm1St1Dr1Cmd"=304, "Rm1St2Dr1Cmd"=305, "Rm1St3Dr1Cmd"=306, "Rm1St4Dr1Cmd"=307, "Rm1St5Dr1Cmd"=308, "Rm1St6Dr1Cmd"=309, "Rm1St7Dr1Cmd"=310, "Rm1St8Dr1Cmd"=311, "Rm1St1Dr2Cmd"=312, "Rm1St2Dr2Cmd"=313, "Rm1St3Dr2Cmd"=314, "Rm1St4Dr2Cmd"=315, "Rm1St5Dr2Cmd"=316, "Rm1St6Dr2Cmd"=317, "Rm1St7Dr2Cmd"=318, "Rm1St8Dr2Cmd"=319, "Rm1St1Dr3Cmd"=320, "Rm1St2Dr3Cmd"=321, "Rm1St3Dr3Cmd"=322, "Rm1St4Dr3Cmd"=323, "Rm1St5Dr3Cmd"=324, "Rm1St6Dr3Cmd"=325, "Rm1St7Dr3Cmd"=326, "Rm1St8Dr3Cmd"=327, "fwRmTempSP"=328, "fwRmHumSP"=329, "fwCoolTempSP"=330, "fwDehumTempSP"=331, "fwRmRun"=332, "fwRmOk"=333, "fwTesting"=334, "fwRmDryP"=335, "fwRmDryI"=336, "fwRmHumP"=337, "fwRmHumI"=338, "fwRmHeatP"=339, "fwRmHeatI"=340, "fwCoolTempP"=341, "fwCoolTempI"=342, "fwDehumTempP"=343, "fwDehumTempI"=344, "fwGndLeak1"=345, "fwGndLeak2"=346, "fwGndLeak3"=347, "fwGndLeak4"=348, "fwGndLeak5"=349, "fwGndLeak6"=350, "fwGndLeak7"=351, "fwGndLeak8"=352, "Rm1OpenerCmd"=353] ("Ring")
            w539 = T27 317 items=["fwS1Volt1"=0, "fwS1Volt2"=1, "fwS2Volt1"=2, "fwS2Volt2"=3, "fwS3Volt1"=4, "fwS3Volt2"=5, "fwS4Volt1"=6, "fwS4Volt2"=7, "fwS5Volt1"=8, "fwS5Volt2"=9, "fwS6Volt1"=10, "fwS6Volt2 "=11, "fwS7Volt1"=12, "fwS7Volt2"=13, "fwS8Volt1"=14, "fwS8Volt2"=15, "fwRoomHum"=16, "fwRoomTemp"=17, "fwAISpare1"=18, "fwAISpare2"=19, "fwSuppTemp"=20, "fwCoolTemp"=21, "fwDehumTemp"=22, "fwUnused"=23, "Bool Inputs"=24, "gwVoltRate1"=256, "gwVoltRate2"=257, "gwVoltRate3"=258, "gwVoltRate4"=259, "gwVoltRate5"=260, "gwVoltRate6"=261, "gwVoltRate7"=262, "gwVoltRate8"=263, "gwVoltWindow5/1"=264, "gwVoltWindow6/2"=265, "gwVoltWindow7/3"=266, "gwVoltWindow8/4"=267, "fwVoltSet1"=272, "fwVoltSet2"=273, "fwVoltSet3"=274, "fwVoltSet4"=275, "fwVoltSet5"=276, "fwVoltSet6"=277, "fwVoltSet7"=278, "fwVoltSet8"=279, "fwVoltRng1"=280, "fwVoltRng2"=281, "fwVoltRng3"=282, "fwVoltRng4"=283, "fwVoltRng5"=284, "fwVoltRng6"=285, "fwVoltRng7"=286, "fwVoltRng8"=287, "fwVoltPol1"=296, "fwVoltPol2"=297, "fwVoltPol3"=298, "fwVoltPol4"=299, "fwVoltPol5"=300, "fwVoltPol6"=301, "fwVoltPol7"=302, "fwVoltPol8"=303, "Rm1St1Dr1Cmd"=304, "Rm1St2Dr1Cmd"=305, "Rm1St3Dr1Cmd"=306, "Rm1St4Dr1Cmd"=307, "Rm1St5Dr1Cmd"=308, "Rm1St6Dr1Cmd"=309, "Rm1St7Dr1Cmd"=310, "Rm1St8Dr1Cmd"=311, "Rm1St1Dr2Cmd"=312, "Rm1St2Dr2Cmd"=313, "Rm1St3Dr2Cmd"=314, "Rm1St4Dr2Cmd"=315, "Rm1St5Dr2Cmd"=316, "Rm1St6Dr2Cmd"=317, "Rm1St7Dr2Cmd"=318, "Rm1St8Dr2Cmd"=319, "Rm1St1Dr3Cmd"=320, "Rm1St2Dr3Cmd"=321, "Rm1St3Dr3Cmd"=322, "Rm1St4Dr3Cmd"=323, "Rm1St5Dr3Cmd"=324, "Rm1St6Dr3Cmd"=325, "Rm1St7Dr3Cmd"=326, "Rm1St8Dr3Cmd"=327, "fwRmTempSP"=328, "fwRmHumSP"=329, "fwCoolTempSP"=330, "fwDehumTempSP"=331, "fwRmRun"=332, "fwRmOk"=333, "fwTesting"=334, "fwRmDryP"=335, "fwRmDryI"=336, "fwRmHumP"=337, "fwRmHumI"=338, "fwRmHeatP"=339, "fwRmHeatI"=340, "fwCoolTempP"=341, "fwCoolTempI"=342, "fwDehumTempP"=343, "fwDehumTempI"=344, "fwGndLeak1"=345, "fwGndLeak2"=346, "fwGndLeak3"=347, "fwGndLeak4"=348, "fwGndLeak5"=349, "fwGndLeak6"=350, "fwGndLeak7"=351, "fwGndLeak8"=352, "Rm1OpenerCmd"=353] ("Ring")
            w540 = T27 309 items=["fwS1Volt1"=0, "fwS1Volt2"=1, "fwS2Volt1"=2, "fwS2Volt2"=3, "fwS3Volt1"=4, "fwS3Volt2"=5, "fwS4Volt1"=6, "fwS4Volt2"=7, "fwS5Volt1"=8, "fwS5Volt2"=9, "fwS6Volt1"=10, "fwS6Volt2 "=11, "fwS7Volt1"=12, "fwS7Volt2"=13, "fwS8Volt1"=14, "fwS8Volt2"=15, "fwRoomHum"=16, "fwRoomTemp"=17, "fwAISpare1"=18, "fwAISpare2"=19, "fwSuppTemp"=20, "fwCoolTemp"=21, "fwDehumTemp"=22, "fwUnused"=23, "Bool Inputs"=24, "gwVoltRate1"=256, "gwVoltRate2"=257, "gwVoltRate3"=258, "gwVoltRate4"=259, "gwVoltRate5"=260, "gwVoltRate6"=261, "gwVoltRate7"=262, "gwVoltRate8"=263, "gwVoltWindow5/1"=264, "gwVoltWindow6/2"=265, "gwVoltWindow7/3"=266, "gwVoltWindow8/4"=267, "fwVoltSet1"=272, "fwVoltSet2"=273, "fwVoltSet3"=274, "fwVoltSet4"=275, "fwVoltSet5"=276, "fwVoltSet6"=277, "fwVoltSet7"=278, "fwVoltSet8"=279, "fwVoltRng1"=280, "fwVoltRng2"=281, "fwVoltRng3"=282, "fwVoltRng4"=283, "fwVoltRng5"=284, "fwVoltRng6"=285, "fwVoltRng7"=286, "fwVoltRng8"=287, "fwVoltPol1"=296, "fwVoltPol2"=297, "fwVoltPol3"=298, "fwVoltPol4"=299, "fwVoltPol5"=300, "fwVoltPol6"=301, "fwVoltPol7"=302, "fwVoltPol8"=303, "Rm1St1Dr1Cmd"=304, "Rm1St2Dr1Cmd"=305, "Rm1St3Dr1Cmd"=306, "Rm1St4Dr1Cmd"=307, "Rm1St5Dr1Cmd"=308, "Rm1St6Dr1Cmd"=309, "Rm1St7Dr1Cmd"=310, "Rm1St8Dr1Cmd"=311, "Rm1St1Dr2Cmd"=312, "Rm1St2Dr2Cmd"=313, "Rm1St3Dr2Cmd"=314, "Rm1St4Dr2Cmd"=315, "Rm1St5Dr2Cmd"=316, "Rm1St6Dr2Cmd"=317, "Rm1St7Dr2Cmd"=318, "Rm1St8Dr2Cmd"=319, "Rm1St1Dr3Cmd"=320, "Rm1St2Dr3Cmd"=321, "Rm1St3Dr3Cmd"=322, "Rm1St4Dr3Cmd"=323, "Rm1St5Dr3Cmd"=324, "Rm1St6Dr3Cmd"=325, "Rm1St7Dr3Cmd"=326, "Rm1St8Dr3Cmd"=327, "fwRmTempSP"=328, "fwRmHumSP"=329, "fwCoolTempSP"=330, "fwDehumTempSP"=331, "fwRmRun"=332, "fwRmOk"=333, "fwTesting"=334, "fwRmDryP"=335, "fwRmDryI"=336, "fwRmHumP"=337, "fwRmHumI"=338, "fwRmHeatP"=339, "fwRmHeatI"=340, "fwCoolTempP"=341, "fwCoolTempI"=342, "fwDehumTempP"=343, "fwDehumTempI"=344, "fwGndLeak1"=345, "fwGndLeak2"=346, "fwGndLeak3"=347, "fwGndLeak4"=348, "fwGndLeak5"=349, "fwGndLeak6"=350, "fwGndLeak7"=351, "fwGndLeak8"=352, "Rm1OpenerCmd"=353] ("Ring")
            n162 = event-data() -> ()  [unwired: 1 in, 6 out]
            n163 = local read "Door Settings"() -> (w530:T11)
            n164 = Unbundle By Name(w530) -> ("Station 6.Slide"=w533:T13, "Station 6.Cab"=w534:T13, "Station 6.Freezer"=w535:T13)
            n165 = call-dynamic "Write Single Holding Register.vi"("error in"=w528, "register to write"=w535, "address"=w540, "Modbus master in"=w527) -> ("error out"=w532:errorcluster, "Modbus master out"=w537:refnum<class "Modbus Master.lvclass">)  [unwired: 6 in]
            n166 = call-dynamic "Write Single Holding Register.vi"("error in"=w532, "register to write"=w534, "address"=w539, "Modbus master in"=w537) -> ("error out"=w531:errorcluster, "Modbus master out"=w536:refnum<class "Modbus Master.lvclass">)  [unwired: 6 in]
            n167 = call-dynamic "Write Single Holding Register.vi"("error in"=w531, "register to write"=w533, "address"=w538, "Modbus master in"=w536) -> ("error out"=w529:errorcluster)  [unwired: 6 in, 1 out]
          }
          event "Station 7 CMD": Value Change {
            w554 = T27 326 items=["fwS1Volt1"=0, "fwS1Volt2"=1, "fwS2Volt1"=2, "fwS2Volt2"=3, "fwS3Volt1"=4, "fwS3Volt2"=5, "fwS4Volt1"=6, "fwS4Volt2"=7, "fwS5Volt1"=8, "fwS5Volt2"=9, "fwS6Volt1"=10, "fwS6Volt2 "=11, "fwS7Volt1"=12, "fwS7Volt2"=13, "fwS8Volt1"=14, "fwS8Volt2"=15, "fwRoomHum"=16, "fwRoomTemp"=17, "fwAISpare1"=18, "fwAISpare2"=19, "fwSuppTemp"=20, "fwCoolTemp"=21, "fwDehumTemp"=22, "fwUnused"=23, "Bool Inputs"=24, "gwVoltRate1"=256, "gwVoltRate2"=257, "gwVoltRate3"=258, "gwVoltRate4"=259, "gwVoltRate5"=260, "gwVoltRate6"=261, "gwVoltRate7"=262, "gwVoltRate8"=263, "gwVoltWindow5/1"=264, "gwVoltWindow6/2"=265, "gwVoltWindow7/3"=266, "gwVoltWindow8/4"=267, "fwVoltSet1"=272, "fwVoltSet2"=273, "fwVoltSet3"=274, "fwVoltSet4"=275, "fwVoltSet5"=276, "fwVoltSet6"=277, "fwVoltSet7"=278, "fwVoltSet8"=279, "fwVoltRng1"=280, "fwVoltRng2"=281, "fwVoltRng3"=282, "fwVoltRng4"=283, "fwVoltRng5"=284, "fwVoltRng6"=285, "fwVoltRng7"=286, "fwVoltRng8"=287, "fwVoltPol1"=296, "fwVoltPol2"=297, "fwVoltPol3"=298, "fwVoltPol4"=299, "fwVoltPol5"=300, "fwVoltPol6"=301, "fwVoltPol7"=302, "fwVoltPol8"=303, "Rm1St1Dr1Cmd"=304, "Rm1St2Dr1Cmd"=305, "Rm1St3Dr1Cmd"=306, "Rm1St4Dr1Cmd"=307, "Rm1St5Dr1Cmd"=308, "Rm1St6Dr1Cmd"=309, "Rm1St7Dr1Cmd"=310, "Rm1St8Dr1Cmd"=311, "Rm1St1Dr2Cmd"=312, "Rm1St2Dr2Cmd"=313, "Rm1St3Dr2Cmd"=314, "Rm1St4Dr2Cmd"=315, "Rm1St5Dr2Cmd"=316, "Rm1St6Dr2Cmd"=317, "Rm1St7Dr2Cmd"=318, "Rm1St8Dr2Cmd"=319, "Rm1St1Dr3Cmd"=320, "Rm1St2Dr3Cmd"=321, "Rm1St3Dr3Cmd"=322, "Rm1St4Dr3Cmd"=323, "Rm1St5Dr3Cmd"=324, "Rm1St6Dr3Cmd"=325, "Rm1St7Dr3Cmd"=326, "Rm1St8Dr3Cmd"=327, "fwRmTempSP"=328, "fwRmHumSP"=329, "fwCoolTempSP"=330, "fwDehumTempSP"=331, "fwRmRun"=332, "fwRmOk"=333, "fwTesting"=334, "fwRmDryP"=335, "fwRmDryI"=336, "fwRmHumP"=337, "fwRmHumI"=338, "fwRmHeatP"=339, "fwRmHeatI"=340, "fwCoolTempP"=341, "fwCoolTempI"=342, "fwDehumTempP"=343, "fwDehumTempI"=344, "fwGndLeak1"=345, "fwGndLeak2"=346, "fwGndLeak3"=347, "fwGndLeak4"=348, "fwGndLeak5"=349, "fwGndLeak6"=350, "fwGndLeak7"=351, "fwGndLeak8"=352, "Rm1OpenerCmd"=353] ("Ring")
            w555 = T27 318 items=["fwS1Volt1"=0, "fwS1Volt2"=1, "fwS2Volt1"=2, "fwS2Volt2"=3, "fwS3Volt1"=4, "fwS3Volt2"=5, "fwS4Volt1"=6, "fwS4Volt2"=7, "fwS5Volt1"=8, "fwS5Volt2"=9, "fwS6Volt1"=10, "fwS6Volt2 "=11, "fwS7Volt1"=12, "fwS7Volt2"=13, "fwS8Volt1"=14, "fwS8Volt2"=15, "fwRoomHum"=16, "fwRoomTemp"=17, "fwAISpare1"=18, "fwAISpare2"=19, "fwSuppTemp"=20, "fwCoolTemp"=21, "fwDehumTemp"=22, "fwUnused"=23, "Bool Inputs"=24, "gwVoltRate1"=256, "gwVoltRate2"=257, "gwVoltRate3"=258, "gwVoltRate4"=259, "gwVoltRate5"=260, "gwVoltRate6"=261, "gwVoltRate7"=262, "gwVoltRate8"=263, "gwVoltWindow5/1"=264, "gwVoltWindow6/2"=265, "gwVoltWindow7/3"=266, "gwVoltWindow8/4"=267, "fwVoltSet1"=272, "fwVoltSet2"=273, "fwVoltSet3"=274, "fwVoltSet4"=275, "fwVoltSet5"=276, "fwVoltSet6"=277, "fwVoltSet7"=278, "fwVoltSet8"=279, "fwVoltRng1"=280, "fwVoltRng2"=281, "fwVoltRng3"=282, "fwVoltRng4"=283, "fwVoltRng5"=284, "fwVoltRng6"=285, "fwVoltRng7"=286, "fwVoltRng8"=287, "fwVoltPol1"=296, "fwVoltPol2"=297, "fwVoltPol3"=298, "fwVoltPol4"=299, "fwVoltPol5"=300, "fwVoltPol6"=301, "fwVoltPol7"=302, "fwVoltPol8"=303, "Rm1St1Dr1Cmd"=304, "Rm1St2Dr1Cmd"=305, "Rm1St3Dr1Cmd"=306, "Rm1St4Dr1Cmd"=307, "Rm1St5Dr1Cmd"=308, "Rm1St6Dr1Cmd"=309, "Rm1St7Dr1Cmd"=310, "Rm1St8Dr1Cmd"=311, "Rm1St1Dr2Cmd"=312, "Rm1St2Dr2Cmd"=313, "Rm1St3Dr2Cmd"=314, "Rm1St4Dr2Cmd"=315, "Rm1St5Dr2Cmd"=316, "Rm1St6Dr2Cmd"=317, "Rm1St7Dr2Cmd"=318, "Rm1St8Dr2Cmd"=319, "Rm1St1Dr3Cmd"=320, "Rm1St2Dr3Cmd"=321, "Rm1St3Dr3Cmd"=322, "Rm1St4Dr3Cmd"=323, "Rm1St5Dr3Cmd"=324, "Rm1St6Dr3Cmd"=325, "Rm1St7Dr3Cmd"=326, "Rm1St8Dr3Cmd"=327, "fwRmTempSP"=328, "fwRmHumSP"=329, "fwCoolTempSP"=330, "fwDehumTempSP"=331, "fwRmRun"=332, "fwRmOk"=333, "fwTesting"=334, "fwRmDryP"=335, "fwRmDryI"=336, "fwRmHumP"=337, "fwRmHumI"=338, "fwRmHeatP"=339, "fwRmHeatI"=340, "fwCoolTempP"=341, "fwCoolTempI"=342, "fwDehumTempP"=343, "fwDehumTempI"=344, "fwGndLeak1"=345, "fwGndLeak2"=346, "fwGndLeak3"=347, "fwGndLeak4"=348, "fwGndLeak5"=349, "fwGndLeak6"=350, "fwGndLeak7"=351, "fwGndLeak8"=352, "Rm1OpenerCmd"=353] ("Ring")
            w556 = T27 310 items=["fwS1Volt1"=0, "fwS1Volt2"=1, "fwS2Volt1"=2, "fwS2Volt2"=3, "fwS3Volt1"=4, "fwS3Volt2"=5, "fwS4Volt1"=6, "fwS4Volt2"=7, "fwS5Volt1"=8, "fwS5Volt2"=9, "fwS6Volt1"=10, "fwS6Volt2 "=11, "fwS7Volt1"=12, "fwS7Volt2"=13, "fwS8Volt1"=14, "fwS8Volt2"=15, "fwRoomHum"=16, "fwRoomTemp"=17, "fwAISpare1"=18, "fwAISpare2"=19, "fwSuppTemp"=20, "fwCoolTemp"=21, "fwDehumTemp"=22, "fwUnused"=23, "Bool Inputs"=24, "gwVoltRate1"=256, "gwVoltRate2"=257, "gwVoltRate3"=258, "gwVoltRate4"=259, "gwVoltRate5"=260, "gwVoltRate6"=261, "gwVoltRate7"=262, "gwVoltRate8"=263, "gwVoltWindow5/1"=264, "gwVoltWindow6/2"=265, "gwVoltWindow7/3"=266, "gwVoltWindow8/4"=267, "fwVoltSet1"=272, "fwVoltSet2"=273, "fwVoltSet3"=274, "fwVoltSet4"=275, "fwVoltSet5"=276, "fwVoltSet6"=277, "fwVoltSet7"=278, "fwVoltSet8"=279, "fwVoltRng1"=280, "fwVoltRng2"=281, "fwVoltRng3"=282, "fwVoltRng4"=283, "fwVoltRng5"=284, "fwVoltRng6"=285, "fwVoltRng7"=286, "fwVoltRng8"=287, "fwVoltPol1"=296, "fwVoltPol2"=297, "fwVoltPol3"=298, "fwVoltPol4"=299, "fwVoltPol5"=300, "fwVoltPol6"=301, "fwVoltPol7"=302, "fwVoltPol8"=303, "Rm1St1Dr1Cmd"=304, "Rm1St2Dr1Cmd"=305, "Rm1St3Dr1Cmd"=306, "Rm1St4Dr1Cmd"=307, "Rm1St5Dr1Cmd"=308, "Rm1St6Dr1Cmd"=309, "Rm1St7Dr1Cmd"=310, "Rm1St8Dr1Cmd"=311, "Rm1St1Dr2Cmd"=312, "Rm1St2Dr2Cmd"=313, "Rm1St3Dr2Cmd"=314, "Rm1St4Dr2Cmd"=315, "Rm1St5Dr2Cmd"=316, "Rm1St6Dr2Cmd"=317, "Rm1St7Dr2Cmd"=318, "Rm1St8Dr2Cmd"=319, "Rm1St1Dr3Cmd"=320, "Rm1St2Dr3Cmd"=321, "Rm1St3Dr3Cmd"=322, "Rm1St4Dr3Cmd"=323, "Rm1St5Dr3Cmd"=324, "Rm1St6Dr3Cmd"=325, "Rm1St7Dr3Cmd"=326, "Rm1St8Dr3Cmd"=327, "fwRmTempSP"=328, "fwRmHumSP"=329, "fwCoolTempSP"=330, "fwDehumTempSP"=331, "fwRmRun"=332, "fwRmOk"=333, "fwTesting"=334, "fwRmDryP"=335, "fwRmDryI"=336, "fwRmHumP"=337, "fwRmHumI"=338, "fwRmHeatP"=339, "fwRmHeatI"=340, "fwCoolTempP"=341, "fwCoolTempI"=342, "fwDehumTempP"=343, "fwDehumTempI"=344, "fwGndLeak1"=345, "fwGndLeak2"=346, "fwGndLeak3"=347, "fwGndLeak4"=348, "fwGndLeak5"=349, "fwGndLeak6"=350, "fwGndLeak7"=351, "fwGndLeak8"=352, "Rm1OpenerCmd"=353] ("Ring")
            n168 = event-data() -> ()  [unwired: 1 in, 6 out]
            n169 = local read "Door Settings"() -> (w546:T11)
            n170 = Unbundle By Name(w546) -> ("Station 7.Slide"=w549:T13, "Station 7.Cab"=w550:T13, "Station 7.Freezer"=w551:T13)
            n171 = call-dynamic "Write Single Holding Register.vi"("error in"=w544, "register to write"=w551, "address"=w556, "Modbus master in"=w543) -> ("error out"=w548:errorcluster, "Modbus master out"=w553:refnum<class "Modbus Master.lvclass">)  [unwired: 6 in]
            n172 = call-dynamic "Write Single Holding Register.vi"("error in"=w548, "register to write"=w550, "address"=w555, "Modbus master in"=w553) -> ("error out"=w547:errorcluster, "Modbus master out"=w552:refnum<class "Modbus Master.lvclass">)  [unwired: 6 in]
            n173 = call-dynamic "Write Single Holding Register.vi"("error in"=w547, "register to write"=w549, "address"=w554, "Modbus master in"=w552) -> ("error out"=w545:errorcluster)  [unwired: 6 in, 1 out]
          }
          event "Station 8 CMD": Value Change {
            w561 = T27 327 items=["fwS1Volt1"=0, "fwS1Volt2"=1, "fwS2Volt1"=2, "fwS2Volt2"=3, "fwS3Volt1"=4, "fwS3Volt2"=5, "fwS4Volt1"=6, "fwS4Volt2"=7, "fwS5Volt1"=8, "fwS5Volt2"=9, "fwS6Volt1"=10, "fwS6Volt2 "=11, "fwS7Volt1"=12, "fwS7Volt2"=13, "fwS8Volt1"=14, "fwS8Volt2"=15, "fwRoomHum"=16, "fwRoomTemp"=17, "fwAISpare1"=18, "fwAISpare2"=19, "fwSuppTemp"=20, "fwCoolTemp"=21, "fwDehumTemp"=22, "fwUnused"=23, "Bool Inputs"=24, "gwVoltRate1"=256, "gwVoltRate2"=257, "gwVoltRate3"=258, "gwVoltRate4"=259, "gwVoltRate5"=260, "gwVoltRate6"=261, "gwVoltRate7"=262, "gwVoltRate8"=263, "gwVoltWindow5/1"=264, "gwVoltWindow6/2"=265, "gwVoltWindow7/3"=266, "gwVoltWindow8/4"=267, "fwVoltSet1"=272, "fwVoltSet2"=273, "fwVoltSet3"=274, "fwVoltSet4"=275, "fwVoltSet5"=276, "fwVoltSet6"=277, "fwVoltSet7"=278, "fwVoltSet8"=279, "fwVoltRng1"=280, "fwVoltRng2"=281, "fwVoltRng3"=282, "fwVoltRng4"=283, "fwVoltRng5"=284, "fwVoltRng6"=285, "fwVoltRng7"=286, "fwVoltRng8"=287, "fwVoltPol1"=296, "fwVoltPol2"=297, "fwVoltPol3"=298, "fwVoltPol4"=299, "fwVoltPol5"=300, "fwVoltPol6"=301, "fwVoltPol7"=302, "fwVoltPol8"=303, "Rm1St1Dr1Cmd"=304, "Rm1St2Dr1Cmd"=305, "Rm1St3Dr1Cmd"=306, "Rm1St4Dr1Cmd"=307, "Rm1St5Dr1Cmd"=308, "Rm1St6Dr1Cmd"=309, "Rm1St7Dr1Cmd"=310, "Rm1St8Dr1Cmd"=311, "Rm1St1Dr2Cmd"=312, "Rm1St2Dr2Cmd"=313, "Rm1St3Dr2Cmd"=314, "Rm1St4Dr2Cmd"=315, "Rm1St5Dr2Cmd"=316, "Rm1St6Dr2Cmd"=317, "Rm1St7Dr2Cmd"=318, "Rm1St8Dr2Cmd"=319, "Rm1St1Dr3Cmd"=320, "Rm1St2Dr3Cmd"=321, "Rm1St3Dr3Cmd"=322, "Rm1St4Dr3Cmd"=323, "Rm1St5Dr3Cmd"=324, "Rm1St6Dr3Cmd"=325, "Rm1St7Dr3Cmd"=326, "Rm1St8Dr3Cmd"=327, "fwRmTempSP"=328, "fwRmHumSP"=329, "fwCoolTempSP"=330, "fwDehumTempSP"=331, "fwRmRun"=332, "fwRmOk"=333, "fwTesting"=334, "fwRmDryP"=335, "fwRmDryI"=336, "fwRmHumP"=337, "fwRmHumI"=338, "fwRmHeatP"=339, "fwRmHeatI"=340, "fwCoolTempP"=341, "fwCoolTempI"=342, "fwDehumTempP"=343, "fwDehumTempI"=344, "fwGndLeak1"=345, "fwGndLeak2"=346, "fwGndLeak3"=347, "fwGndLeak4"=348, "fwGndLeak5"=349, "fwGndLeak6"=350, "fwGndLeak7"=351, "fwGndLeak8"=352, "Rm1OpenerCmd"=353] ("Ring")
            w562 = T27 319 items=["fwS1Volt1"=0, "fwS1Volt2"=1, "fwS2Volt1"=2, "fwS2Volt2"=3, "fwS3Volt1"=4, "fwS3Volt2"=5, "fwS4Volt1"=6, "fwS4Volt2"=7, "fwS5Volt1"=8, "fwS5Volt2"=9, "fwS6Volt1"=10, "fwS6Volt2 "=11, "fwS7Volt1"=12, "fwS7Volt2"=13, "fwS8Volt1"=14, "fwS8Volt2"=15, "fwRoomHum"=16, "fwRoomTemp"=17, "fwAISpare1"=18, "fwAISpare2"=19, "fwSuppTemp"=20, "fwCoolTemp"=21, "fwDehumTemp"=22, "fwUnused"=23, "Bool Inputs"=24, "gwVoltRate1"=256, "gwVoltRate2"=257, "gwVoltRate3"=258, "gwVoltRate4"=259, "gwVoltRate5"=260, "gwVoltRate6"=261, "gwVoltRate7"=262, "gwVoltRate8"=263, "gwVoltWindow5/1"=264, "gwVoltWindow6/2"=265, "gwVoltWindow7/3"=266, "gwVoltWindow8/4"=267, "fwVoltSet1"=272, "fwVoltSet2"=273, "fwVoltSet3"=274, "fwVoltSet4"=275, "fwVoltSet5"=276, "fwVoltSet6"=277, "fwVoltSet7"=278, "fwVoltSet8"=279, "fwVoltRng1"=280, "fwVoltRng2"=281, "fwVoltRng3"=282, "fwVoltRng4"=283, "fwVoltRng5"=284, "fwVoltRng6"=285, "fwVoltRng7"=286, "fwVoltRng8"=287, "fwVoltPol1"=296, "fwVoltPol2"=297, "fwVoltPol3"=298, "fwVoltPol4"=299, "fwVoltPol5"=300, "fwVoltPol6"=301, "fwVoltPol7"=302, "fwVoltPol8"=303, "Rm1St1Dr1Cmd"=304, "Rm1St2Dr1Cmd"=305, "Rm1St3Dr1Cmd"=306, "Rm1St4Dr1Cmd"=307, "Rm1St5Dr1Cmd"=308, "Rm1St6Dr1Cmd"=309, "Rm1St7Dr1Cmd"=310, "Rm1St8Dr1Cmd"=311, "Rm1St1Dr2Cmd"=312, "Rm1St2Dr2Cmd"=313, "Rm1St3Dr2Cmd"=314, "Rm1St4Dr2Cmd"=315, "Rm1St5Dr2Cmd"=316, "Rm1St6Dr2Cmd"=317, "Rm1St7Dr2Cmd"=318, "Rm1St8Dr2Cmd"=319, "Rm1St1Dr3Cmd"=320, "Rm1St2Dr3Cmd"=321, "Rm1St3Dr3Cmd"=322, "Rm1St4Dr3Cmd"=323, "Rm1St5Dr3Cmd"=324, "Rm1St6Dr3Cmd"=325, "Rm1St7Dr3Cmd"=326, "Rm1St8Dr3Cmd"=327, "fwRmTempSP"=328, "fwRmHumSP"=329, "fwCoolTempSP"=330, "fwDehumTempSP"=331, "fwRmRun"=332, "fwRmOk"=333, "fwTesting"=334, "fwRmDryP"=335, "fwRmDryI"=336, "fwRmHumP"=337, "fwRmHumI"=338, "fwRmHeatP"=339, "fwRmHeatI"=340, "fwCoolTempP"=341, "fwCoolTempI"=342, "fwDehumTempP"=343, "fwDehumTempI"=344, "fwGndLeak1"=345, "fwGndLeak2"=346, "fwGndLeak3"=347, "fwGndLeak4"=348, "fwGndLeak5"=349, "fwGndLeak6"=350, "fwGndLeak7"=351, "fwGndLeak8"=352, "Rm1OpenerCmd"=353] ("Ring")
            w574 = T27 311 items=["fwS1Volt1"=0, "fwS1Volt2"=1, "fwS2Volt1"=2, "fwS2Volt2"=3, "fwS3Volt1"=4, "fwS3Volt2"=5, "fwS4Volt1"=6, "fwS4Volt2"=7, "fwS5Volt1"=8, "fwS5Volt2"=9, "fwS6Volt1"=10, "fwS6Volt2 "=11, "fwS7Volt1"=12, "fwS7Volt2"=13, "fwS8Volt1"=14, "fwS8Volt2"=15, "fwRoomHum"=16, "fwRoomTemp"=17, "fwAISpare1"=18, "fwAISpare2"=19, "fwSuppTemp"=20, "fwCoolTemp"=21, "fwDehumTemp"=22, "fwUnused"=23, "Bool Inputs"=24, "gwVoltRate1"=256, "gwVoltRate2"=257, "gwVoltRate3"=258, "gwVoltRate4"=259, "gwVoltRate5"=260, "gwVoltRate6"=261, "gwVoltRate7"=262, "gwVoltRate8"=263, "gwVoltWindow5/1"=264, "gwVoltWindow6/2"=265, "gwVoltWindow7/3"=266, "gwVoltWindow8/4"=267, "fwVoltSet1"=272, "fwVoltSet2"=273, "fwVoltSet3"=274, "fwVoltSet4"=275, "fwVoltSet5"=276, "fwVoltSet6"=277, "fwVoltSet7"=278, "fwVoltSet8"=279, "fwVoltRng1"=280, "fwVoltRng2"=281, "fwVoltRng3"=282, "fwVoltRng4"=283, "fwVoltRng5"=284, "fwVoltRng6"=285, "fwVoltRng7"=286, "fwVoltRng8"=287, "fwVoltPol1"=296, "fwVoltPol2"=297, "fwVoltPol3"=298, "fwVoltPol4"=299, "fwVoltPol5"=300, "fwVoltPol6"=301, "fwVoltPol7"=302, "fwVoltPol8"=303, "Rm1St1Dr1Cmd"=304, "Rm1St2Dr1Cmd"=305, "Rm1St3Dr1Cmd"=306, "Rm1St4Dr1Cmd"=307, "Rm1St5Dr1Cmd"=308, "Rm1St6Dr1Cmd"=309, "Rm1St7Dr1Cmd"=310, "Rm1St8Dr1Cmd"=311, "Rm1St1Dr2Cmd"=312, "Rm1St2Dr2Cmd"=313, "Rm1St3Dr2Cmd"=314, "Rm1St4Dr2Cmd"=315, "Rm1St5Dr2Cmd"=316, "Rm1St6Dr2Cmd"=317, "Rm1St7Dr2Cmd"=318, "Rm1St8Dr2Cmd"=319, "Rm1St1Dr3Cmd"=320, "Rm1St2Dr3Cmd"=321, "Rm1St3Dr3Cmd"=322, "Rm1St4Dr3Cmd"=323, "Rm1St5Dr3Cmd"=324, "Rm1St6Dr3Cmd"=325, "Rm1St7Dr3Cmd"=326, "Rm1St8Dr3Cmd"=327, "fwRmTempSP"=328, "fwRmHumSP"=329, "fwCoolTempSP"=330, "fwDehumTempSP"=331, "fwRmRun"=332, "fwRmOk"=333, "fwTesting"=334, "fwRmDryP"=335, "fwRmDryI"=336, "fwRmHumP"=337, "fwRmHumI"=338, "fwRmHeatP"=339, "fwRmHeatI"=340, "fwCoolTempP"=341, "fwCoolTempI"=342, "fwDehumTempP"=343, "fwDehumTempI"=344, "fwGndLeak1"=345, "fwGndLeak2"=346, "fwGndLeak3"=347, "fwGndLeak4"=348, "fwGndLeak5"=349, "fwGndLeak6"=350, "fwGndLeak7"=351, "fwGndLeak8"=352, "Rm1OpenerCmd"=353] ("Ring")
            n174 = event-data() -> ()  [unwired: 1 in, 6 out]
            n175 = local read "Door Settings"() -> (w568:T11)
            n176 = Unbundle By Name(w568) -> ("Station 8.Slide"=w570:T13, "Station 8.Cab"=w571:T13, "Station 8.Freezer"=w572:T13)
            n177 = call-dynamic "Write Single Holding Register.vi"("error in"=w565, "register to write"=w572, "address"=w574, "Modbus master in"=w566) -> ("error out"=w569:errorcluster, "Modbus master out"=w573:refnum<class "Modbus Master.lvclass">)  [unwired: 6 in]
            n178 = call-dynamic "Write Single Holding Register.vi"("error in"=w569, "register to write"=w571, "address"=w562, "Modbus master in"=w573) -> ("error out"=w559:errorcluster, "Modbus master out"=w560:refnum<class "Modbus Master.lvclass">)  [unwired: 6 in]
            n179 = call-dynamic "Write Single Holding Register.vi"("error in"=w559, "register to write"=w570, "address"=w561, "Modbus master in"=w560) -> ("error out"=w567:errorcluster)  [unwired: 6 in, 1 out]
          }
          event Value Change {
            w579 = T27 353 items=["fwS1Volt1"=0, "fwS1Volt2"=1, "fwS2Volt1"=2, "fwS2Volt2"=3, "fwS3Volt1"=4, "fwS3Volt2"=5, "fwS4Volt1"=6, "fwS4Volt2"=7, "fwS5Volt1"=8, "fwS5Volt2"=9, "fwS6Volt1"=10, "fwS6Volt2 "=11, "fwS7Volt1"=12, "fwS7Volt2"=13, "fwS8Volt1"=14, "fwS8Volt2"=15, "fwRoomHum"=16, "fwRoomTemp"=17, "fwAISpare1"=18, "fwAISpare2"=19, "fwSuppTemp"=20, "fwCoolTemp"=21, "fwDehumTemp"=22, "fwUnused"=23, "Bool Inputs"=24, "gwVoltRate1"=256, "gwVoltRate2"=257, "gwVoltRate3"=258, "gwVoltRate4"=259, "gwVoltRate5"=260, "gwVoltRate6"=261, "gwVoltRate7"=262, "gwVoltRate8"=263, "gwVoltWindow5/1"=264, "gwVoltWindow6/2"=265, "gwVoltWindow7/3"=266, "gwVoltWindow8/4"=267, "fwVoltSet1"=272, "fwVoltSet2"=273, "fwVoltSet3"=274, "fwVoltSet4"=275, "fwVoltSet5"=276, "fwVoltSet6"=277, "fwVoltSet7"=278, "fwVoltSet8"=279, "fwVoltRng1"=280, "fwVoltRng2"=281, "fwVoltRng3"=282, "fwVoltRng4"=283, "fwVoltRng5"=284, "fwVoltRng6"=285, "fwVoltRng7"=286, "fwVoltRng8"=287, "fwVoltPol1"=296, "fwVoltPol2"=297, "fwVoltPol3"=298, "fwVoltPol4"=299, "fwVoltPol5"=300, "fwVoltPol6"=301, "fwVoltPol7"=302, "fwVoltPol8"=303, "Rm1St1Dr1Cmd"=304, "Rm1St2Dr1Cmd"=305, "Rm1St3Dr1Cmd"=306, "Rm1St4Dr1Cmd"=307, "Rm1St5Dr1Cmd"=308, "Rm1St6Dr1Cmd"=309, "Rm1St7Dr1Cmd"=310, "Rm1St8Dr1Cmd"=311, "Rm1St1Dr2Cmd"=312, "Rm1St2Dr2Cmd"=313, "Rm1St3Dr2Cmd"=314, "Rm1St4Dr2Cmd"=315, "Rm1St5Dr2Cmd"=316, "Rm1St6Dr2Cmd"=317, "Rm1St7Dr2Cmd"=318, "Rm1St8Dr2Cmd"=319, "Rm1St1Dr3Cmd"=320, "Rm1St2Dr3Cmd"=321, "Rm1St3Dr3Cmd"=322, "Rm1St4Dr3Cmd"=323, "Rm1St5Dr3Cmd"=324, "Rm1St6Dr3Cmd"=325, "Rm1St7Dr3Cmd"=326, "Rm1St8Dr3Cmd"=327, "fwRmTempSP"=328, "fwRmHumSP"=329, "fwCoolTempSP"=330, "fwDehumTempSP"=331, "fwRmRun"=332, "fwRmOk"=333, "fwTesting"=334, "fwRmDryP"=335, "fwRmDryI"=336, "fwRmHumP"=337, "fwRmHumI"=338, "fwRmHeatP"=339, "fwRmHeatI"=340, "fwCoolTempP"=341, "fwCoolTempI"=342, "fwDehumTempP"=343, "fwDehumTempI"=344, "fwGndLeak1"=345, "fwGndLeak2"=346, "fwGndLeak3"=347, "fwGndLeak4"=348, "fwGndLeak5"=349, "fwGndLeak6"=350, "fwGndLeak7"=351, "fwGndLeak8"=352, "Rm1OpenerCmd"=353] ("Ring")
            # "Enable the Door Openers"
            n180 = event-data() -> ("NewVal"=w575:T14)  [unwired: 1 in, 5 out]
            n181 = call-dynamic "Write Single Holding Register.vi"("error in"=w578, "register to write"=w575, "address"=w579, "Modbus master in"=w576) -> ("error out"=w577:errorcluster)  [unwired: 6 in, 1 out]
          }
          event Value Change {
            w583 = T27 333 items=["fwS1Volt1"=0, "fwS1Volt2"=1, "fwS2Volt1"=2, "fwS2Volt2"=3, "fwS3Volt1"=4, "fwS3Volt2"=5, "fwS4Volt1"=6, "fwS4Volt2"=7, "fwS5Volt1"=8, "fwS5Volt2"=9, "fwS6Volt1"=10, "fwS6Volt2 "=11, "fwS7Volt1"=12, "fwS7Volt2"=13, "fwS8Volt1"=14, "fwS8Volt2"=15, "fwRoomHum"=16, "fwRoomTemp"=17, "fwAISpare1"=18, "fwAISpare2"=19, "fwSuppTemp"=20, "fwCoolTemp"=21, "fwDehumTemp"=22, "fwUnused"=23, "Bool Inputs"=24, "gwVoltRate1"=256, "gwVoltRate2"=257, "gwVoltRate3"=258, "gwVoltRate4"=259, "gwVoltRate5"=260, "gwVoltRate6"=261, "gwVoltRate7"=262, "gwVoltRate8"=263, "gwVoltWindow5/1"=264, "gwVoltWindow6/2"=265, "gwVoltWindow7/3"=266, "gwVoltWindow8/4"=267, "fwVoltSet1"=272, "fwVoltSet2"=273, "fwVoltSet3"=274, "fwVoltSet4"=275, "fwVoltSet5"=276, "fwVoltSet6"=277, "fwVoltSet7"=278, "fwVoltSet8"=279, "fwVoltRng1"=280, "fwVoltRng2"=281, "fwVoltRng3"=282, "fwVoltRng4"=283, "fwVoltRng5"=284, "fwVoltRng6"=285, "fwVoltRng7"=286, "fwVoltRng8"=287, "fwVoltPol1"=296, "fwVoltPol2"=297, "fwVoltPol3"=298, "fwVoltPol4"=299, "fwVoltPol5"=300, "fwVoltPol6"=301, "fwVoltPol7"=302, "fwVoltPol8"=303, "Rm1St1Dr1Cmd"=304, "Rm1St2Dr1Cmd"=305, "Rm1St3Dr1Cmd"=306, "Rm1St4Dr1Cmd"=307, "Rm1St5Dr1Cmd"=308, "Rm1St6Dr1Cmd"=309, "Rm1St7Dr1Cmd"=310, "Rm1St8Dr1Cmd"=311, "Rm1St1Dr2Cmd"=312, "Rm1St2Dr2Cmd"=313, "Rm1St3Dr2Cmd"=314, "Rm1St4Dr2Cmd"=315, "Rm1St5Dr2Cmd"=316, "Rm1St6Dr2Cmd"=317, "Rm1St7Dr2Cmd"=318, "Rm1St8Dr2Cmd"=319, "Rm1St1Dr3Cmd"=320, "Rm1St2Dr3Cmd"=321, "Rm1St3Dr3Cmd"=322, "Rm1St4Dr3Cmd"=323, "Rm1St5Dr3Cmd"=324, "Rm1St6Dr3Cmd"=325, "Rm1St7Dr3Cmd"=326, "Rm1St8Dr3Cmd"=327, "fwRmTempSP"=328, "fwRmHumSP"=329, "fwCoolTempSP"=330, "fwDehumTempSP"=331, "fwRmRun"=332, "fwRmOk"=333, "fwTesting"=334, "fwRmDryP"=335, "fwRmDryI"=336, "fwRmHumP"=337, "fwRmHumI"=338, "fwRmHeatP"=339, "fwRmHeatI"=340, "fwCoolTempP"=341, "fwCoolTempI"=342, "fwDehumTempP"=343, "fwDehumTempI"=344, "fwGndLeak1"=345, "fwGndLeak2"=346, "fwGndLeak3"=347, "fwGndLeak4"=348, "fwGndLeak5"=349, "fwGndLeak6"=350, "fwGndLeak7"=351, "fwGndLeak8"=352, "Rm1OpenerCmd"=353] ("Ring")
            n182 = event-data() -> ("NewVal"=w584:T4)  [unwired: 1 in, 5 out]
            n183 = call-dynamic "Write Single Holding Register.vi"("error in"=w586, "register to write"=w584, "address"=w583, "Modbus master in"=w582) -> ("error out"=w585:errorcluster)  [unwired: 6 in, 1 out]
          }
          event Value Change {
            w593 = T27 332 items=["fwS1Volt1"=0, "fwS1Volt2"=1, "fwS2Volt1"=2, "fwS2Volt2"=3, "fwS3Volt1"=4, "fwS3Volt2"=5, "fwS4Volt1"=6, "fwS4Volt2"=7, "fwS5Volt1"=8, "fwS5Volt2"=9, "fwS6Volt1"=10, "fwS6Volt2 "=11, "fwS7Volt1"=12, "fwS7Volt2"=13, "fwS8Volt1"=14, "fwS8Volt2"=15, "fwRoomHum"=16, "fwRoomTemp"=17, "fwAISpare1"=18, "fwAISpare2"=19, "fwSuppTemp"=20, "fwCoolTemp"=21, "fwDehumTemp"=22, "fwUnused"=23, "Bool Inputs"=24, "gwVoltRate1"=256, "gwVoltRate2"=257, "gwVoltRate3"=258, "gwVoltRate4"=259, "gwVoltRate5"=260, "gwVoltRate6"=261, "gwVoltRate7"=262, "gwVoltRate8"=263, "gwVoltWindow5/1"=264, "gwVoltWindow6/2"=265, "gwVoltWindow7/3"=266, "gwVoltWindow8/4"=267, "fwVoltSet1"=272, "fwVoltSet2"=273, "fwVoltSet3"=274, "fwVoltSet4"=275, "fwVoltSet5"=276, "fwVoltSet6"=277, "fwVoltSet7"=278, "fwVoltSet8"=279, "fwVoltRng1"=280, "fwVoltRng2"=281, "fwVoltRng3"=282, "fwVoltRng4"=283, "fwVoltRng5"=284, "fwVoltRng6"=285, "fwVoltRng7"=286, "fwVoltRng8"=287, "fwVoltPol1"=296, "fwVoltPol2"=297, "fwVoltPol3"=298, "fwVoltPol4"=299, "fwVoltPol5"=300, "fwVoltPol6"=301, "fwVoltPol7"=302, "fwVoltPol8"=303, "Rm1St1Dr1Cmd"=304, "Rm1St2Dr1Cmd"=305, "Rm1St3Dr1Cmd"=306, "Rm1St4Dr1Cmd"=307, "Rm1St5Dr1Cmd"=308, "Rm1St6Dr1Cmd"=309, "Rm1St7Dr1Cmd"=310, "Rm1St8Dr1Cmd"=311, "Rm1St1Dr2Cmd"=312, "Rm1St2Dr2Cmd"=313, "Rm1St3Dr2Cmd"=314, "Rm1St4Dr2Cmd"=315, "Rm1St5Dr2Cmd"=316, "Rm1St6Dr2Cmd"=317, "Rm1St7Dr2Cmd"=318, "Rm1St8Dr2Cmd"=319, "Rm1St1Dr3Cmd"=320, "Rm1St2Dr3Cmd"=321, "Rm1St3Dr3Cmd"=322, "Rm1St4Dr3Cmd"=323, "Rm1St5Dr3Cmd"=324, "Rm1St6Dr3Cmd"=325, "Rm1St7Dr3Cmd"=326, "Rm1St8Dr3Cmd"=327, "fwRmTempSP"=328, "fwRmHumSP"=329, "fwCoolTempSP"=330, "fwDehumTempSP"=331, "fwRmRun"=332, "fwRmOk"=333, "fwTesting"=334, "fwRmDryP"=335, "fwRmDryI"=336, "fwRmHumP"=337, "fwRmHumI"=338, "fwRmHeatP"=339, "fwRmHeatI"=340, "fwCoolTempP"=341, "fwCoolTempI"=342, "fwDehumTempP"=343, "fwDehumTempI"=344, "fwGndLeak1"=345, "fwGndLeak2"=346, "fwGndLeak3"=347, "fwGndLeak4"=348, "fwGndLeak5"=349, "fwGndLeak6"=350, "fwGndLeak7"=351, "fwGndLeak8"=352, "Rm1OpenerCmd"=353] ("Ring")
            n184 = event-data() -> ("NewVal"=w589:T5)  [unwired: 1 in, 5 out]
            n185 = call-dynamic "Write Single Holding Register.vi"("error in"=w592, "register to write"=w589, "address"=w593, "Modbus master in"=w590) -> ("error out"=w591:errorcluster)  [unwired: 6 in, 1 out]
          }
          event "Update Voltage Adjustment Parameters": Value Change {
            n186 = event-data() -> ()  [unwired: 1 in, 6 out]
            n187 = call "Wago Update Voltage Adjustment Parameters.vi"("error in (no error)"=w599, "Voltage Adjustment Parameters"="Voltage Adjustment Parameters", "Modbus Master in"=w597) -> ("error out"=w598:errorcluster)  [unwired: 7 in, 1 out]
          }
          event "Room PID Parameters": Value Change {
            n188 = event-data() -> ()  [unwired: 1 in, 6 out]
            n189 = call <vilib>:"Add State(s) to Queue__jki_lib_state_machine.vi"("State(s) in Front (\"\")"="Set Room PIDs" ("State(s) in Front (\"\")"), "State(s) in (\"\")"=w604) -> ("States Out"=w603:string)  [unwired: 13 in]
          }
          event "Chamber Setpoint": Value Change {
            n190 = event-data() -> ()  [unwired: 1 in, 6 out]
            n191 = call "Wago Chamber Setpoints.vi"("error in (no error)"=w610, "Room Setpoints"="Room Setpoints", "Modbus Master in"=w608) -> ("error out"=w609:errorcluster)  [unwired: 7 in, 1 out]
          }
          event "OK": Value Change {
            # "Exit Button Value Change (pressed) Event\n(this executes Macro: Exit to terminate the VI)"
            n192 = event-data() -> ()  [unwired: 1 in, 1 out]
            n193 = call <vilib>:"Add State(s) to Queue__jki_lib_state_machine.vi"("State(s) in Front (\"\")"="Macro: Exit", "State(s) in (\"\")"=w617) -> ("States Out"=w616:string)  [unwired: 13 in]
          }
          event Panel Close? {
            # "Discard the event because we'll close the front panel ourselves in Macro: Exit"
            # "Close Panel button (pressed) Event\n(this executes Macro: Exit to terminate the VI)"
            n194 = event-data() -> ()  [unwired: 1 in, 1 out]
            n195 = event-data("Discard?"=TRUE) -> ()  [unwired: 1 in, 1 out]
            n196 = call <vilib>:"Add State(s) to Queue__jki_lib_state_machine.vi"("State(s) in Front (\"\")"="Macro: Exit", "State(s) in (\"\")"=w623) -> ("States Out"=w622:string)  [unwired: 13 in]
          }
        }
      }
      frame "---------- Core ----------" {
        # "Do not put any code in this frame.\n(it is a separator no-op)"
        n197 = call <vilib>:"Add State(s) to Queue__jki_lib_state_machine.vi"("State(s) in (\"\")"=w627) -> ("States Out"=w626:string)  [unwired: 14 in]
      }
      frame Default {
        w637 = 42 items=["No error", "Argument error", "Memory is full", "Out of zone", "End of file", "File already open", "Generic file I/O error", "File not found", "File permission error", "Disk is full", "Duplicate path", "Too many files open", "System feature not enabled", "Resource file not found", "Cannot add resource", "Resource not found", "Image not found", "Image memory error", "Pen does not exist", "Config type invalid", "Config token not found", "Config parse error", "Config memory error", "Bad external code format", "Bad external code offset", "External code not present", "Null window", "Destroy window error", "Null menu", "Print aborted", "Bad print record", "Print driver error", "Windows error during printing", "Memory error during printing", "Print dialog error", "Generic print error", "Invalid device refnum", "Device not found", "Device parameter error", "Device unit error", "Cannot open device", "Device call aborted", "Generic error", "Cancelled by user", "Object ID too low", "Object ID too high", "Object not in heap", "Unknown heap", "Unknown object (invalid DefProc)", "Unknown object (DefProc not in table)", "Message out of range", "Invalid (null) method", "Unknown message", "Manager call not supported", "Bad address", "Network operation in progress", "Network operation timed out", "Connection is busy", "Network attribute not supported", "Network error", "Address in use", "System out of memory", "Connection aborted", "Connection refused", "Not connected", "Already connected", "Connection closed", "Initialization error (interapplication manager)", "Bad occurrence", "Wait on unbound occurrence handler", "Occurrence queue overflow", "Datalog type conflict", "Unused", "Unrecognized type (interapplication manager)", "Memory corrupt", "Failed to make temporary DLL", "Old CIN version", "Drag socket not found", "Failed to load drop-object", "Failed to register OLE object", "Failed to release OLE object", "Format specifier type mismatch", "Unknown format specifier", "Too few format specifiers", "Too many format specifiers", "Scan failed", "Newer CIN version", "Error converting to variant", "Runtime menu error", "Password tampered", "Variant attribute not found", "Incompatible variant data type", "Event data is not available", "Event Store is not present", "Occurrence is not found", "Event Queue is not created", "Event info is not available", "Refnum passed is NULL", "Error retrieving Class GUID", "Error retrieving CoClass GUID", "Error retrieving TypeLib GUID.", "Bad built application magic bytes.", "Specific driver is different from the specific driver associated with the Logical Name.", "There is no session opened to the class driver.", "Max Error", "MAX - Error with config objects", "MAX - Error loading configuration", "MAX - Group not supported"]
        # "Current State"
        # "Do not delete, rename, or modify this frame.\n(this is used to capture unhandled states and typos)"
        # "Handle mistyped state name (developer tool)"
        n198 = Format Into String(format string="Software Exception: Unhandled State \"%s\"." ("message"), error in=w633, w628) -> (resulting string=w636:string, error out=w635:errorcluster)  [unwired: 1 in]
        n199 = call <vilib>:"Error Cluster From Error Code.vi"("show call chain? (False)"=TRUE, "error in (no error)"=w635, "error message (\"\")"=w636, "error code (0)"=w637) -> ("error out"=w634:errorcluster)  [unwired: 5 in]
        n200 = call <vilib>:"Add State(s) to Queue__jki_lib_state_machine.vi"("State(s) in (\"\")"=w632) -> ("States Out"=w631:string)  [unwired: 14 in]
      }
      frame "Initialize Core Data" {
        # "Do not delete, rename, or modify this frame.\n(this is used to determine panel behavior on exit)"
        # "originally closed?"
        # "exe?"
        # "If panel starts closed or is an EXE, then close it when we exit"
        n201 = property class="VI"() -> ("Front Panel.Open"=w646:bool)  [unwired: 2 in, 2 out]
        n202 = property class="App"() -> ("App.Kind"=w645:T23)  [unwired: 2 in, 2 out]
        n203 = control-ref of="Current VI Reference"() -> (w639:refnum<vi>)
        n204 = Not(x=w646) -> (.not. x?=w643:bool)
        n205 = Equal?(x=w645, y=T23."Run Time System" ("Application:Kind")) -> (x = y?=w642:bool)
        n206 = Or(x=w643, y=w642) -> (x .or. y?=w640:bool)
        n207 = Bundle By Name(cluster=w641, "Core.Current VI Reference"=w639, "Core.Close Panel on Exit?"=w640) -> (w648:T28)
        n208 = call <vilib>:"Add State(s) to Queue__jki_lib_state_machine.vi"("State(s) in (\"\")"=w650) -> ("States Out"=w649:string)  [unwired: 14 in]
      }
      frame "Error Handler" {
        # "Unhandled Error -- Display it"
        # "Handle any errors here.\nYou can also output any states to clean-up after errors occur"
        # "Clear error"
        n209 = call <vilib>:"General Error Handler.vi"("error in (no error)"=w652) -> ()  [unwired: 10 in, 5 out]
        n210 = call <vilib>:"Add State(s) to Queue__jki_lib_state_machine.vi"("State(s) in Front (\"\")"="/* Post Error States", "State(s) in (\"\")"=w656) -> ("States Out"=w655:string)  [unwired: 13 in]
      }
      frame "Exit" {
        # "Do not put any code in this frame.\n(No errors that occur here will be handled.)"
        n211 = call <vilib>:"Add State(s) to Queue__jki_lib_state_machine.vi"("State(s) in (\"\")"=w661) -> ("States Out"=w660:string)  [unwired: 14 in]
      }
      frame "---------- Data ----------" {
        # "Do not put any code in this frame.\n(It is a separator no-op. You can make a copy of this frame to create a new Data frame)"
        n212 = call <vilib>:"Add State(s) to Queue__jki_lib_state_machine.vi"("State(s) in (\"\")"=w665) -> ("States Out"=w664:string)  [unwired: 14 in]
      }
      frame "Data: Initialize" {
        w666 = T26 {"Current VI Reference"=refnum, "Close Panel on Exit?"=FALSE}  # Core
        w668 = TRUE  # Your Boolean data
        w667 = ""  # Your string data
        # "do not delete - used by framework"
        # "Expand Bundle to add new data elements to shift register data."
        # "Add new data here."
        # "Data names and types of shift register data are defined by this bundle."
        # "Initialize the shift-register data, here.\n(data names are defined by what you wire into the bundle function)"
        n213 = Bundle("Core"=w666, "Your Boolean data"=w668, "Your string data"=w667) -> (w670:T28)  [unwired: 1 in]
        n214 = call <vilib>:"Add State(s) to Queue__jki_lib_state_machine.vi"("State(s) in (\"\")"=w672) -> ("States Out"=w671:string)  [unwired: 14 in]
      }
      frame "Data: Cleanup" {
        # "Cleanup any data and references, here.\n(this is called automatically, by the Macro: Exit)"
        n215 = Unbundle By Name(w673) -> ("Core.Current VI Reference"=w676:refnum<vi>)
        n216 = Close Reference(reference=w676, error in (no error)=w675) -> (error out=w674:errorcluster)
        n217 = call <vilib>:"Add State(s) to Queue__jki_lib_state_machine.vi"("State(s) in (\"\")"=w678) -> ("States Out"=w677:string)  [unwired: 14 in]
      }
      frame "---------- UI ----------" {
        # "Do not put any code in this frame.\n(It is a separator no-op. You can make a copy of this frame to create a new UI frame)"
        n218 = call <vilib>:"Add State(s) to Queue__jki_lib_state_machine.vi"("State(s) in (\"\")"=w682) -> ("States Out"=w681:string)  [unwired: 14 in]
      }
      frame "UI: Initialize" {
        # "Initialize the User Interface, here.\n(this is called automatically, by the Macro: Init)"
        n219 = call <vilib>:"Add State(s) to Queue__jki_lib_state_machine.vi"("State(s) in (\"\")"=w686) -> ("States Out"=w685:string)  [unwired: 14 in]
      }
      frame "UI: Cursor Set" {
        # "Argument"
        # "Set and Unset Cursor Busy.\n(Usage: \"UI: Cursor Set >> Busy|Idle\")"
        n220 = case shown="\"Idle\", Default" w687 {
          tunnel: w689 -> [w694 w696]
          tunnel: [w693 w695] -> w688
          frame "Idle", Default {
            n221 = call <vilib>:"Unset Busy.vi"("error in (no error)"=w694) -> ("error out"=w693:errorcluster)  [unwired: 10 in]
          }
          frame "Busy" {
            n222 = call <vilib>:"Set Busy.vi"("error in (no error)"=w696) -> ("error out"=w695:errorcluster)  [unwired: 9 in, 1 out]
          }
        }
        n223 = call <vilib>:"Add State(s) to Queue__jki_lib_state_machine.vi"("State(s) in (\"\")"=w692) -> ("States Out"=w691:string)  [unwired: 14 in]
      }
      frame "UI: Front Panel State" {
        # "Argument"
        # "Set Front Panel Open or Closed\n(Usage: \"UI: Front Panel State >> Open|Close\")"
        n224 = Unbundle By Name(w699) -> ("Core.Current VI Reference"=w698:refnum<vi>)
        n225 = case shown="\"Open\", Default" w697 {
          tunnel: w701 -> [w707 w720]
          tunnel: [w709 w721] -> w700
          tunnel: w698 -> [w708 w718]
          frame "Open", Default {
            n226 = property class="VI"(reference=w708, error in=w707) -> (reference out=w705:refnum<vi>, error out=w706:errorcluster, "Front Panel.Open"=w704:bool)
            n227 = case shown="False" w704 {
              tunnel: [w712 w715] -> w709
              tunnel: w706 -> [w711 w715]
              tunnel: w705 -> [w710 _]
              frame False {
                n228 = invoke class="VI" method="FP.Open"(reference=w710, error in=w711, "Activate"=TRUE, "State"=T24."Standard") -> (error out=w712:errorcluster)  [unwired: 1 in, 4 out]
              }
              frame True {
              }
            }
          }
          frame "Close" {
            n229 = property class="VI"(reference=w718, error in=w720) -> (reference out=w717:refnum<vi>, error out=w719:errorcluster, "Front Panel.Open"=w716:bool)
            n230 = case shown="True" w716 {
              tunnel: [w722 w725] -> w721
              tunnel: w719 -> [w722 w724]
              tunnel: w717 -> [_ w723]
              frame False {
              }
              frame True {
                n231 = invoke class="VI" method="FP.Close"(reference=w723, error in=w724) -> (error out=w725:errorcluster)  [unwired: 1 in, 2 out]
              }
            }
          }
        }
        n232 = call <vilib>:"Add State(s) to Queue__jki_lib_state_machine.vi"("State(s) in (\"\")"=w703) -> ("States Out"=w702:string)  [unwired: 14 in]
      }
      frame "---------- Macro ----------" {
        # "Do not put any code in this frame.\n(It is a separator no-op. You can make a copy of this frame to create a new Macro frame)"
        n233 = call <vilib>:"Add State(s) to Queue__jki_lib_state_machine.vi"("State(s) in (\"\")"=w729) -> ("States Out"=w728:string)  [unwired: 14 in]
      }
      frame "Macro: Initialize" {
        w730 = "Data: Initialize\nInitialize Core Data\nUI: Initialize\nUI: Front Panel State >> Open"  # Data: Initialize Initialize Core Data UI: Initialize UI: Front Panel State >> Open
        # "Initialization Macro\n(This is called once, when the VI starts)"
        n234 = call <vilib>:"Add State(s) to Queue__jki_lib_state_machine.vi"("State(s) in Front (\"\")"=w730, "State(s) in (\"\")"=w734) -> ("States Out"=w733:string)  [unwired: 13 in]
      }
      frame "Macro: Exit" {
        # "Exit Macro\n(This is called once, when the VI exits)"
        n235 = Unbundle By Name(w741) -> ("Core.Close Panel on Exit?"=w740:bool)
        n236 = Select(t="UI: Front Panel State >> Close", s=w740, f="") -> (s? t:f=w737:string)
        n237 = call <vilib>:"Add State(s) to Queue__jki_lib_state_machine.vi"("State(s) in (\"\")"=w737, "State(s) at Back (\"\")"="Data: Cleanup\nExit") -> ("States Out"=w735:string)  [unwired: 13 in]
        n238 = call <vilib>:"Add State(s) to Queue__jki_lib_state_machine.vi"("State(s) in Front (\"\")"=w735, "State(s) in (\"\")"=w744) -> ("States Out"=w743:string)  [unwired: 13 in]
      }
      frame "---------- New Category ----------" {
        # "Template Separator\n(You can make a copy of, or modify, this frame)"
        n239 = call <vilib>:"Add State(s) to Queue__jki_lib_state_machine.vi"("State(s) in (\"\")"=w748) -> ("States Out"=w747:string)  [unwired: 14 in]
      }
      frame "Set Room PIDs" {
        n240 = call "Wago Room PID Setting SET.vi"("error in (no error)"=w751, "Room PID Settings"="Room PID Settings", "Modbus Master in"=w749) -> ("error out"=w750:errorcluster)  [unwired: 7 in, 1 out]
        n241 = call <vilib>:"Add State(s) to Queue__jki_lib_state_machine.vi"("State(s) in (\"\")"=w755) -> ("States Out"=w754:string)  [unwired: 14 in]
      }
      frame "New Category: 2" {
        # "Your code here.\n(You can make a copy of, or modify, this frame)"
        n242 = call <vilib>:"Add State(s) to Queue__jki_lib_state_machine.vi"("State(s) in (\"\")"=w759) -> ("States Out"=w758:string)  [unwired: 14 in]
      }
    }
  }
  n243 = call-dynamic "Shutdown.vi"("error in"=w6, "Modbus master in"=w5) -> ("error out"=w9:errorcluster)  [unwired: 9 in]
  n244 = call <vilib>:"Simple Error Handler.vi"("error in (no error)"=w9) -> ("error out"=→"Error Out":errorcluster)  [unwired: 1 in, 7 out]
